vi "界面-新.vi"() -> ()   [LabVIEW 2018]
panel:
  out "已开盖次数":dbl
  in  "保存文件名":string
  in  "保存路径":path
  out "状态记录":string
  in  "保存时间":bool
  out "关盖缓冲异常":bool
  out "字符串 9":string
  out "开盖缓冲异常":bool
  out "字符串 8":string
  in  "开盖次数设置":dbl
  in  "退出系统":bool
  in  "锁定":bool
  in  "压紧":bool
  in  "开盖":bool
  in  "关盖":bool
  in  "解锁":bool
  in  "松开":bool
  in  "井盖 8":bool
  in  "井盖 7":bool
  in  "井盖 6":bool
  in  "井盖 5":bool
  in  "井盖 4":bool
  in  "井盖 3":bool
  in  "井盖 2":bool
  in  "井盖1":bool
  out "字符串 7":string
  out "字符串 6":string
  out "字符串 5":string
  out "字符串 4":string
  out "字符串 3":string
  out "字符串 2":string
  out "解锁异常":bool
  out "压紧时间":dbl
  out "锁定时间":dbl
  out "松开时间":dbl
  out "开盖时间":dbl
  out "解锁时间":dbl
  out "关盖时间":dbl
  out "压紧异常":bool
  out "关盖异常":bool
  out "锁定异常":bool
  out "开盖异常":bool
  out "松开异常":bool
  in  "显示/保存数据":bool
  in  "numsamples":i32=1000
  in  "IP Port 2":string="22222" caption="IP Port"
  in  "IP Address 2":string="192.168.0.10" caption="IP Address"
  in  "间隔时间4s":bool
  in  "间隔时间3s":bool
  in  "间隔时间2s":bool
  in  "调试模式":bool
  in  "自动操作":bool
  in  "手动操作":bool
  in  "系统启动":bool
  out "压紧换向阀":bool
  out "压紧到位":bool
  out "锁定到位":bool
  out "松开换向阀":bool
  out "开盖指令2":bool
  out "开盖指令1":bool
  out "开盖换向阀":bool
  out "开盖缓冲":bool
  out "开盖到位2":bool
  out "解锁到位":bool
  out "关盖指令2":bool
  out "关盖指令1":bool
  out "关盖换向阀":bool
  out "关盖到位2":bool
  out "关盖到位1":bool
  out "松开到位":bool
  out "关盖缓冲":bool
  out "开盖到位1":bool
  out "时间":string
  out "日期":string
  # "数 据 分 析 平 台 监 控 界 面"
  # "动 作 指 令"
  # "状 态 显 示"
  # "报 警 信 息"
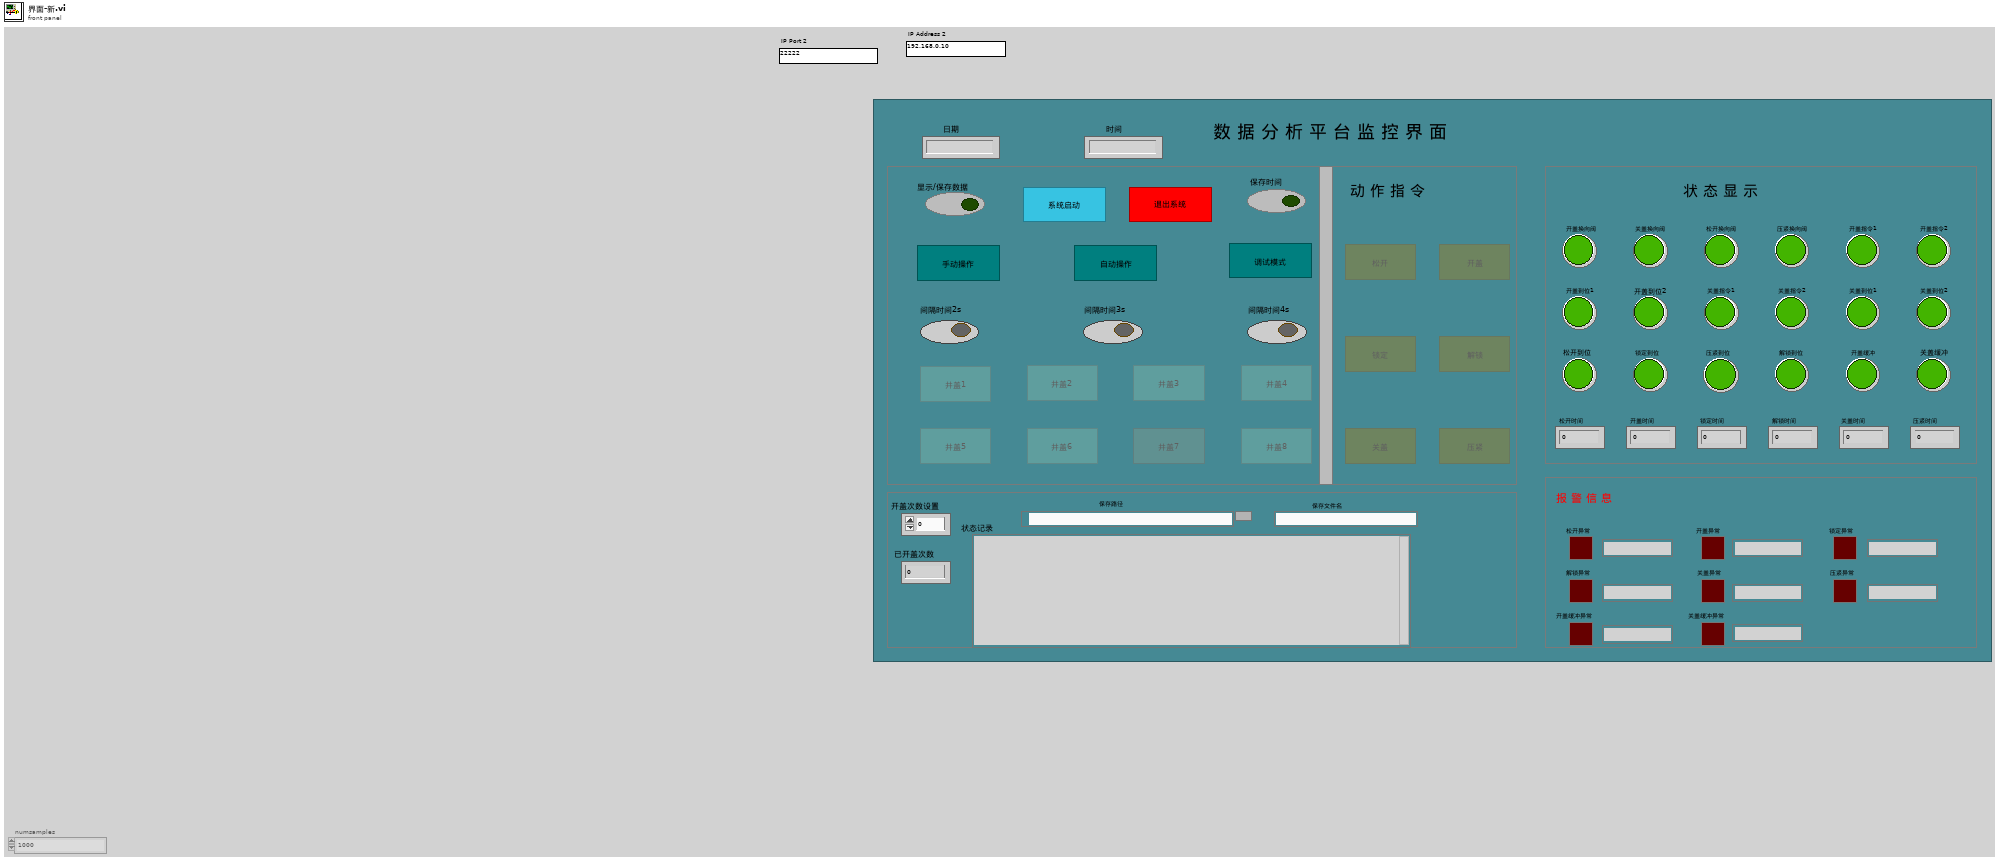
[diagram p1: front panel]
types:
  T1 = enum8{"Enabled", "Disabled", "Disabled and Grayed Out"}
  T2 = enum16{"open", "replace", "create", "open or create", "replace or create", "replace or create with confirmation"}
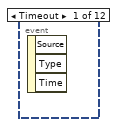
[diagram p17: hidden frame]
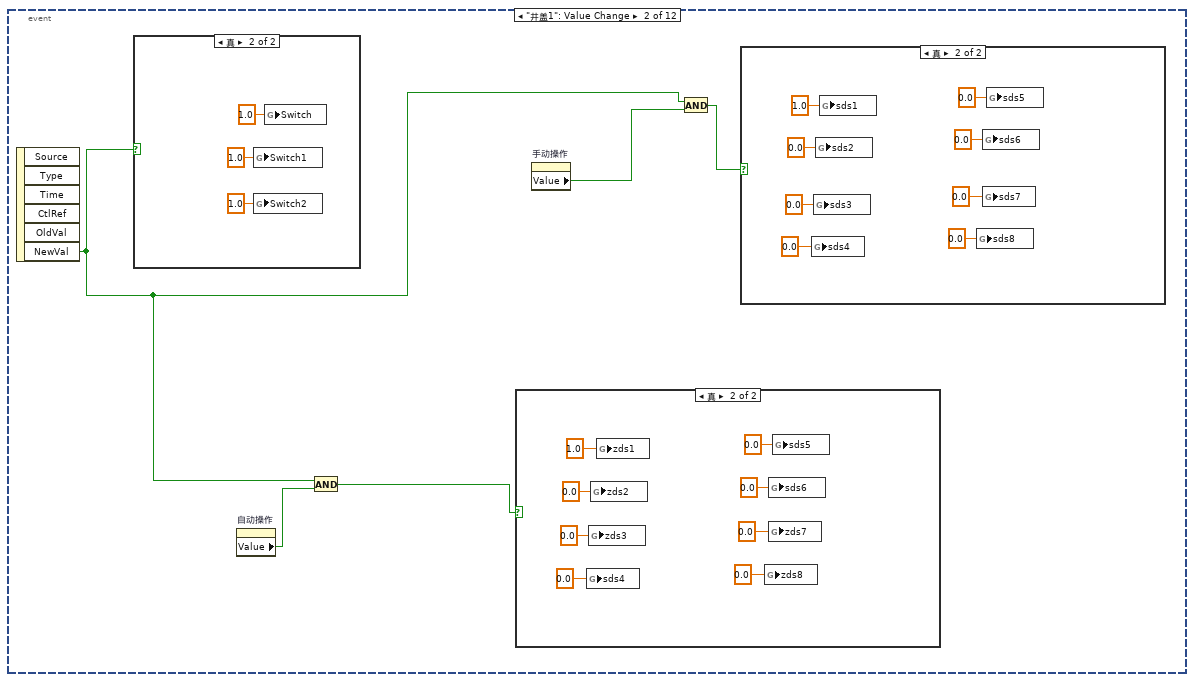
[diagram p18: hidden frame]
diagram:
  w182 = FALSE
  w181 = FALSE
  w171 = FALSE
  w172 = FALSE
  w173 = FALSE
  w174 = FALSE
  w199 = FALSE
  w175 = FALSE
  w176 = FALSE
  w177 = FALSE
  w178 = FALSE
  w179 = FALSE
  w180 = FALSE
  w201 = FALSE
  w202 = FALSE
  w203 = FALSE
  w204 = FALSE
  w205 = FALSE
  w206 = FALSE
  w207 = FALSE
  w200 = FALSE
  w208 = FALSE
  w209 = FALSE
  w210 = FALSE
  w211 = FALSE
  w212 = FALSE
  w213 = FALSE
  w214 = FALSE
  w215 = FALSE
  w216 = FALSE
  w217 = FALSE
  n1 = call "xPCOpenTcpIpPort.vi"("port"="IP Port 2", "address"="IP Address 2") -> ("error out"=w102:errorcluster, "Port"=w93:i32)
  n2 = Unbundle By Name(w102) -> ("status"=w106:bool)
  n3 = call "xPCLoadApp.vi"("pathstr"="C:\\Users\\zczg\\Desktop\\kaigguangai\\remake", "filename"="kaiguangai1108", "port"=w93) -> ("error out"=w103:errorcluster, "port copy"=w92:i32)  [unwired: 1 in]
  n4 = Unbundle By Name(w103) -> ()  [unwired: 1 out]
  n5 = Select(t="上下位机连接失败!" ("message"), s=w106, f="上下位机建立连接!" ("message")) -> ()  [unwired: 1 out]
  n6 = call "xPCStartApp.vi"("port"=w92) -> ("port copy"=w3:i32)  [unwired: 1 in, 1 out]
  n7 = call "xPCGetParamIdx.vi"("blockpath"="shoudongcaozuo/s6", "parametername"="Value", "port"=w3) -> ("identifier"=w382:i32, "port copy"=w383:i32)  [unwired: 1 in, 1 out]
  n8 = call "xPCGetParamIdx.vi"("blockpath"="shoudongcaozuo/s5", "parametername"="Value", "port"=w3) -> ("identifier"=w377:i32, "port copy"=w380:i32)  [unwired: 1 in, 1 out]
  n9 = call "xPCGetParamIdx.vi"("blockpath"="shoudongcaozuo/s3", "parametername"="Value", "port"=w3) -> ("identifier"=w6:i32, "port copy"=w7:i32)  [unwired: 1 in, 1 out]
  n10 = call "xPCGetParamIdx.vi"("blockpath"="shoudongcaozuo/s4", "parametername"="Value", "port"=w3) -> ("identifier"=w373:i32, "port copy"=w374:i32)  [unwired: 1 in, 1 out]
  n11 = for {
    N: 1 -> [_]
    tunnel: [w389] -> w2 mode=indexing
    tunnel: [w388] -> w1 mode=indexing
    tunnel: string[] ["Subsystem1/Data Type Conversion2", "", "", "", "", "", "", "", "", ""] -> [w387] mode=indexing
    tunnel: w3 -> [w386]
    n12 = call "xPCGetSigIdx.vi"("blockpath"=w387, "port"=w386) -> ("identifier"=w388:i32, "port copy"=w389:i32)  [unwired: 1 in, 1 out]
  }
  n13 = call "xPCGetParamIdx.vi"("blockpath"="shoudongcaozuo/s2", "parametername"="Value", "port"=w3) -> ("identifier"=w366:i32, "port copy"=w367:i32)  [unwired: 1 in, 1 out]
  n14 = for {
    N: 6 -> [_]
    tunnel: [w393] -> w114 mode=indexing
    tunnel: [w392] -> w113 mode=indexing
    tunnel: string[] ["Subsystem1/shoudong/Data Type Conversion7/s1", "Subsystem1/shoudong/Data Type Conversion7/s2", "Subsystem1/shoudong/Data Type Conversion7/s3", "Subsystem1/shoudong/Data Type Conversion7/s4", "Subsystem1/shoudong/Data Type Conversion7/s5", "Subsystem1/shoudong/Data Type Conversion7/s6", "", "", "", ""] -> [w391] mode=indexing
    tunnel: w3 -> [w390]
    n15 = call "xPCGetSigIdx.vi"("blockpath"=w391, "port"=w390) -> ("identifier"=w392:i32, "port copy"=w393:i32)  [unwired: 1 in, 1 out]
  }
  n16 = for {
    N: 6 -> [_]
    tunnel: [w397] -> w116 mode=indexing
    tunnel: [w396] -> w115 mode=indexing
    tunnel: string[] ["Subsystem1/shoudong/Data Type Conversion8/s1", "Subsystem1/shoudong/Data Type Conversion8/s2", "Subsystem1/shoudong/Data Type Conversion8/s3", "Subsystem1/shoudong/Data Type Conversion8/s4", "Subsystem1/shoudong/Data Type Conversion8/s5", "Subsystem1/shoudong/Data Type Conversion8/s6", "", "", "", ""] -> [w395] mode=indexing
    tunnel: w3 -> [w394]
    n17 = call "xPCGetSigIdx.vi"("blockpath"=w395, "port"=w394) -> ("identifier"=w396:i32, "port copy"=w397:i32)  [unwired: 1 in, 1 out]
  }
  n18 = for {
    N: 6 -> [_]
    tunnel: [w401] -> w118 mode=indexing
    tunnel: [w400] -> w117 mode=indexing
    tunnel: string[] ["Subsystem1/shoudong/Data Type Conversion9/s1", "Subsystem1/shoudong/Data Type Conversion9/s2", "Subsystem1/shoudong/Data Type Conversion9/s3", "Subsystem1/shoudong/Data Type Conversion9/s4", "Subsystem1/shoudong/Data Type Conversion9/s5", "Subsystem1/shoudong/Data Type Conversion9/s6", "", "", "", ""] -> [w399] mode=indexing
    tunnel: w3 -> [w398]
    n19 = call "xPCGetSigIdx.vi"("blockpath"=w399, "port"=w398) -> ("identifier"=w400:i32, "port copy"=w401:i32)  [unwired: 1 in, 1 out]
  }
  n20 = call "xPCGetParamIdx.vi"("blockpath"="tiaoshidongzuo/yajin", "parametername"="Value", "port"=w3) -> ("identifier"=w17:i32, "port copy"=w18:i32)  [unwired: 1 in, 1 out]
  n21 = for {
    N: 1 -> [_]
    tunnel: [w405] -> w13 mode=indexing
    tunnel: [w404] -> w12 mode=indexing
    tunnel: string[] ["Subsystem1/Data Type Conversion1", "", "", "", "", "", "", "", "", ""] -> [w403] mode=indexing
    tunnel: w3 -> [w402]
    n22 = call "xPCGetSigIdx.vi"("blockpath"=w403, "port"=w402) -> ("identifier"=w404:i32, "port copy"=w405:i32)  [unwired: 1 in, 1 out]
  }
  n23 = call "xPCGetParamIdx.vi"("blockpath"="shoudongcaozuo/s1", "parametername"="Value", "port"=w3) -> ("identifier"=w361:i32, "port copy"=w362:i32)  [unwired: 1 in, 1 out]
  n24 = for {
    N: 1 -> [_]
    tunnel: [w409] -> w9 mode=indexing
    tunnel: [w408] -> w8 mode=indexing
    tunnel: string[] ["Subsystem1/Data Type Conversion2", "", "", "", "", "", "", "", "", ""] -> [w407] mode=indexing
    tunnel: w3 -> [w406]
    n25 = call "xPCGetSigIdx.vi"("blockpath"=w407, "port"=w406) -> ("identifier"=w408:i32, "port copy"=w409:i32)  [unwired: 1 in, 1 out]
  }
  n26 = for {
    N: 6 -> [_]
    tunnel: [w413] -> w120 mode=indexing
    tunnel: [w412] -> w119 mode=indexing
    tunnel: string[] ["Subsystem1/shoudong/Data Type Conversion10/s1", "Subsystem1/shoudong/Data Type Conversion10/s2", "Subsystem1/shoudong/Data Type Conversion10/s3", "Subsystem1/shoudong/Data Type Conversion10/s4", "Subsystem1/shoudong/Data Type Conversion10/s5", "Subsystem1/shoudong/Data Type Conversion10/s6", "", "", "", ""] -> [w411] mode=indexing
    tunnel: w3 -> [w410]
    n27 = call "xPCGetSigIdx.vi"("blockpath"=w411, "port"=w410) -> ("identifier"=w412:i32, "port copy"=w413:i32)  [unwired: 1 in, 1 out]
  }
  n28 = call "xPCGetParamIdx.vi"("blockpath"="tiaoshidongzuo/jiesuo", "parametername"="Value", "port"=w3) -> ("identifier"=w29:i32, "port copy"=w30:i32)  [unwired: 1 in, 1 out]
  n29 = call "xPCGetParamIdx.vi"("blockpath"="shoudongcaozuo/s7", "parametername"="Value", "port"=w3) -> ("identifier"=w194:i32, "port copy"=w195:i32)  [unwired: 1 in, 1 out]
  n30 = call "xPCGetParamIdx.vi"("blockpath"="tiaoshidongzuo/kaigai", "parametername"="Value", "port"=w3) -> ("identifier"=w26:i32, "port copy"=w27:i32)  [unwired: 1 in, 1 out]
  n31 = for {
    N: 6 -> [_]
    tunnel: [w417] -> w112 mode=indexing
    tunnel: [w416] -> w111 mode=indexing
    tunnel: string[] ["Subsystem1/shoudong/Data Type Conversion6/s1", "Subsystem1/shoudong/Data Type Conversion6/s2", "Subsystem1/shoudong/Data Type Conversion6/s3", "Subsystem1/shoudong/Data Type Conversion6/s4", "Subsystem1/shoudong/Data Type Conversion6/s5", "Subsystem1/shoudong/Data Type Conversion6/s6", "", "", "", ""] -> [w415] mode=indexing
    tunnel: w3 -> [w414]
    n32 = call "xPCGetSigIdx.vi"("blockpath"=w415, "port"=w414) -> ("identifier"=w416:i32, "port copy"=w417:i32)  [unwired: 1 in, 1 out]
  }
  n33 = for {
    N: 6 -> [_]
    tunnel: [w421] -> w160 mode=indexing
    tunnel: [w420] -> w159 mode=indexing
    tunnel: string[] ["Subsystem1/zidong/Data Type Conversion3/s1", "Subsystem1/zidong/Data Type Conversion3/s2", "Subsystem1/zidong/Data Type Conversion3/s3", "Subsystem1/zidong/Data Type Conversion3/s4", "Subsystem1/zidong/Data Type Conversion3/s5", "Subsystem1/zidong/Data Type Conversion3/s6", "", "", "", ""] -> [w419] mode=indexing
    tunnel: w3 -> [w418]
    n34 = call "xPCGetSigIdx.vi"("blockpath"=w419, "port"=w418) -> ("identifier"=w420:i32, "port copy"=w421:i32)  [unwired: 1 in, 1 out]
  }
  n35 = for {
    N: 6 -> [_]
    tunnel: [w425] -> w144 mode=indexing
    tunnel: [w424] -> w143 mode=indexing
    tunnel: string[] ["Subsystem1/zidong/Data Type Conversion5/s1", "Subsystem1/zidong/Data Type Conversion5/s2", "Subsystem1/zidong/Data Type Conversion5/s3", "Subsystem1/zidong/Data Type Conversion5/s4", "Subsystem1/zidong/Data Type Conversion5/s5", "Subsystem1/zidong/Data Type Conversion5/s6", "", "", "", ""] -> [w423] mode=indexing
    tunnel: w3 -> [w422]
    n36 = call "xPCGetSigIdx.vi"("blockpath"=w423, "port"=w422) -> ("identifier"=w424:i32, "port copy"=w425:i32)  [unwired: 1 in, 1 out]
  }
  n37 = call "xPCGetParamIdx.vi"("blockpath"="tiaoshidongzuo/suoding", "parametername"="Value", "port"=w3) -> ("identifier"=w20:i32, "port copy"=w21:i32)  [unwired: 1 in, 1 out]
  n38 = call "xPCGetParamIdx.vi"("blockpath"="shoudongcaozuo/jiesuo", "parametername"="Value", "port"=w3) -> ("identifier"=w346:i32, "port copy"=w347:i32)  [unwired: 1 in, 1 out]
  n39 = call "xPCGetParamIdx.vi"("blockpath"="shoudongcaozuo/suoding", "parametername"="Value", "port"=w3) -> ("identifier"=w341:i32, "port copy"=w342:i32)  [unwired: 1 in, 1 out]
  n40 = for {
    N: 6 -> [_]
    tunnel: [w429] -> w138 mode=indexing
    tunnel: [w428] -> w137 mode=indexing
    tunnel: string[] ["Subsystem1/zidong/Data Type Conversion8/s1", "Subsystem1/zidong/Data Type Conversion8/s2", "Subsystem1/zidong/Data Type Conversion8/s3", "Subsystem1/zidong/Data Type Conversion8/s4", "Subsystem1/zidong/Data Type Conversion8/s5", "Subsystem1/zidong/Data Type Conversion8/s6", "", "", "", ""] -> [w427] mode=indexing
    tunnel: w3 -> [w426]
    n41 = call "xPCGetSigIdx.vi"("blockpath"=w427, "port"=w426) -> ("identifier"=w428:i32, "port copy"=w429:i32)  [unwired: 1 in, 1 out]
  }
  n42 = for {
    N: 6 -> [_]
    tunnel: [w433] -> w164 mode=indexing
    tunnel: [w432] -> w163 mode=indexing
    tunnel: string[] ["Subsystem1/zidong/Data Type Conversion1/s1", "Subsystem1/zidong/Data Type Conversion1/s2", "Subsystem1/zidong/Data Type Conversion1/s3", "Subsystem1/zidong/Data Type Conversion1/s4", "Subsystem1/zidong/Data Type Conversion1/s5", "Subsystem1/zidong/Data Type Conversion1/s6", "", "", "", ""] -> [w431] mode=indexing
    tunnel: w3 -> [w430]
    n43 = call "xPCGetSigIdx.vi"("blockpath"=w431, "port"=w430) -> ("identifier"=w432:i32, "port copy"=w433:i32)  [unwired: 1 in, 1 out]
  }
  n44 = for {
    N: 6 -> [_]
    tunnel: [w437] -> w156 mode=indexing
    tunnel: [w436] -> w155 mode=indexing
    tunnel: string[] ["Subsystem1/zidong/Data Type Conversion4/s1", "Subsystem1/zidong/Data Type Conversion4/s2", "Subsystem1/zidong/Data Type Conversion4/s3", "Subsystem1/zidong/Data Type Conversion4/s4", "Subsystem1/zidong/Data Type Conversion4/s5", "Subsystem1/zidong/Data Type Conversion4/s6", "", "", "", ""] -> [w435] mode=indexing
    tunnel: w3 -> [w434]
    n45 = call "xPCGetSigIdx.vi"("blockpath"=w435, "port"=w434) -> ("identifier"=w436:i32, "port copy"=w437:i32)  [unwired: 1 in, 1 out]
  }
  n46 = call "xPCGetParamIdx.vi"("blockpath"="shoudongcaozuo/yajin", "parametername"="Value", "port"=w3) -> ("identifier"=w355:i32, "port copy"=w356:i32)  [unwired: 1 in, 1 out]
  n47 = call "xPCGetParamIdx.vi"("blockpath"="shoudongcaozuo/kaigai", "parametername"="Value", "port"=w3) -> ("identifier"=w336:i32, "port copy"=w337:i32)  [unwired: 1 in, 1 out]
  n48 = for {
    N: 4 -> [_]
    tunnel: [w441] -> w219 mode=indexing
    tunnel: [w440] -> w218 mode=indexing
    tunnel: string[] ["Subsystem1/Data Type Conversion1/s1", "Subsystem1/Data Type Conversion1/s2", "Subsystem1/Data Type Conversion1/s3", "Subsystem1/Data Type Conversion1/s4"] -> [w439] mode=indexing
    tunnel: w3 -> [w438]
    n49 = call "xPCGetSigIdx.vi"("blockpath"=w439, "port"=w438) -> ("identifier"=w440:i32, "port copy"=w441:i32)  [unwired: 1 in, 1 out]
  }
  n50 = call "xPCGetParamIdx.vi"("blockpath"="shoudongcaozuo/guangai", "parametername"="Value", "port"=w3) -> ("identifier"=w352:i32, "port copy"=w353:i32)  [unwired: 1 in, 1 out]
  n51 = for {
    N: 6 -> [_]
    tunnel: [w445] -> w136 mode=indexing
    tunnel: [w444] -> w135 mode=indexing
    tunnel: string[] ["Subsystem1/shoudong/Data Type Conversion1/s1", "Subsystem1/shoudong/Data Type Conversion1/s2", "Subsystem1/shoudong/Data Type Conversion1/s3", "Subsystem1/shoudong/Data Type Conversion1/s4", "Subsystem1/shoudong/Data Type Conversion1/s5", "Subsystem1/shoudong/Data Type Conversion1/s6", "", "", "", ""] -> [w443] mode=indexing
    tunnel: w3 -> [w442]
    n52 = call "xPCGetSigIdx.vi"("blockpath"=w443, "port"=w442) -> ("identifier"=w444:i32, "port copy"=w445:i32)  [unwired: 1 in, 1 out]
  }
  n53 = for {
    N: 6 -> [_]
    tunnel: [w449] -> w140 mode=indexing
    tunnel: [w448] -> w139 mode=indexing
    tunnel: string[] ["Subsystem1/zidong/Data Type Conversion7/s1", "Subsystem1/zidong/Data Type Conversion7/s2", "Subsystem1/zidong/Data Type Conversion7/s3", "Subsystem1/zidong/Data Type Conversion7/s4", "Subsystem1/zidong/Data Type Conversion7/s5", "Subsystem1/zidong/Data Type Conversion7/s6", "", "", "", ""] -> [w447] mode=indexing
    tunnel: w3 -> [w446]
    n54 = call "xPCGetSigIdx.vi"("blockpath"=w447, "port"=w446) -> ("identifier"=w448:i32, "port copy"=w449:i32)  [unwired: 1 in, 1 out]
  }
  n55 = call "xPCGetParamIdx.vi"("blockpath"="tiaoshidongzuo/songkai", "parametername"="Value", "port"=w3) -> ("identifier"=w23:i32, "port copy"=w24:i32)  [unwired: 1 in, 1 out]
  n56 = for {
    N: 6 -> [_]
    tunnel: [w453] -> w142 mode=indexing
    tunnel: [w452] -> w141 mode=indexing
    tunnel: string[] ["Subsystem1/zidong/Data Type Conversion6/s1", "Subsystem1/zidong/Data Type Conversion6/s2", "Subsystem1/zidong/Data Type Conversion6/s3", "Subsystem1/zidong/Data Type Conversion6/s4", "Subsystem1/zidong/Data Type Conversion6/s5", "Subsystem1/zidong/Data Type Conversion6/s6", "", "", "", ""] -> [w451] mode=indexing
    tunnel: w3 -> [w450]
    n57 = call "xPCGetSigIdx.vi"("blockpath"=w451, "port"=w450) -> ("identifier"=w452:i32, "port copy"=w453:i32)  [unwired: 1 in, 1 out]
  }
  n58 = for {
    N: 6 -> [_]
    tunnel: [w457] -> w110 mode=indexing
    tunnel: [w456] -> w109 mode=indexing
    tunnel: string[] ["Subsystem1/shoudong/Data Type Conversion5/s1", "Subsystem1/shoudong/Data Type Conversion5/s2", "Subsystem1/shoudong/Data Type Conversion5/s3", "Subsystem1/shoudong/Data Type Conversion5/s4", "Subsystem1/shoudong/Data Type Conversion5/s5", "Subsystem1/shoudong/Data Type Conversion5/s6", "", "", "", ""] -> [w455] mode=indexing
    tunnel: w3 -> [w454]
    n59 = call "xPCGetSigIdx.vi"("blockpath"=w455, "port"=w454) -> ("identifier"=w456:i32, "port copy"=w457:i32)  [unwired: 1 in, 1 out]
  }
  n60 = call "xPCGetParamIdx.vi"("blockpath"="tiaoshidongzuo/guangai", "parametername"="Value", "port"=w3) -> ("identifier"=w32:i32, "port copy"=w33:i32)  [unwired: 1 in, 1 out]
  n61 = for {
    N: 6 -> [_]
    tunnel: [w461] -> w108 mode=indexing
    tunnel: [w460] -> w107 mode=indexing
    tunnel: string[] ["Subsystem1/shoudong/Data Type Conversion2/s1", "Subsystem1/shoudong/Data Type Conversion2/s2", "Subsystem1/shoudong/Data Type Conversion2/s3", "Subsystem1/shoudong/Data Type Conversion2/s4", "Subsystem1/shoudong/Data Type Conversion2/s5", "Subsystem1/shoudong/Data Type Conversion2/s6", "", "", "", ""] -> [w459] mode=indexing
    tunnel: w3 -> [w458]
    n62 = call "xPCGetSigIdx.vi"("blockpath"=w459, "port"=w458) -> ("identifier"=w460:i32, "port copy"=w461:i32)  [unwired: 1 in, 1 out]
  }
  n63 = call "xPCGetParamIdx.vi"("blockpath"="shoudongcaozuo/s8", "parametername"="Value", "port"=w3) -> ("identifier"=w95:i32, "port copy"=w96:i32)  [unwired: 1 in, 1 out]
  n64 = for {
    N: 4 -> [_]
    tunnel: [w465] -> w225 mode=indexing
    tunnel: [w464] -> w224 mode=indexing
    tunnel: string[] ["Data Type Conversion2/s1", "Data Type Conversion2/s2", "Data Type Conversion2/s3", "Data Type Conversion2/s4", "", "", "", ""] -> [w463] mode=indexing
    tunnel: w3 -> [w462]
    n65 = call "xPCGetSigIdx.vi"("blockpath"=w463, "port"=w462) -> ("identifier"=w464:i32, "port copy"=w465:i32)  [unwired: 1 in, 1 out]
  }
  n66 = for {
    N: 6 -> [_]
    tunnel: [w469] -> w222 mode=indexing
    tunnel: [w468] -> w221 mode=indexing
    tunnel: string[] ["Data Type Conversion/s1", "Data Type Conversion/s2", "Data Type Conversion/s3", "Data Type Conversion/s4", "Data Type Conversion/s5", "Data Type Conversion/s6"] -> [w467] mode=indexing
    tunnel: w3 -> [w466]
    n67 = call "xPCGetSigIdx.vi"("blockpath"=w467, "port"=w466) -> ("identifier"=w468:i32, "port copy"=w469:i32)  [unwired: 1 in, 1 out]
  }
  n68 = for {
    N: 6 -> [_]
    tunnel: [w473] -> w168 mode=indexing
    tunnel: [w472] -> w167 mode=indexing
    tunnel: string[] ["Subsystem1/zidong/Data Type Conversion2/s1", "Subsystem1/zidong/Data Type Conversion2/s2", "Subsystem1/zidong/Data Type Conversion2/s3", "Subsystem1/zidong/Data Type Conversion2/s4", "Subsystem1/zidong/Data Type Conversion2/s5", "Subsystem1/zidong/Data Type Conversion2/s6", "", "", "", ""] -> [w471] mode=indexing
    tunnel: w3 -> [w470]
    n69 = call "xPCGetSigIdx.vi"("blockpath"=w471, "port"=w470) -> ("identifier"=w472:i32, "port copy"=w473:i32)  [unwired: 1 in, 1 out]
  }
  n70 = call "xPCGetParamIdx.vi"("blockpath"="Switch2", "parametername"="Value", "port"=w3) -> ("identifier"=w327:i32, "port copy"=w328:i32)  [unwired: 1 in, 1 out]
  n71 = call "xPCGetParamIdx.vi"("blockpath"="tiaoshidongzuo/s3", "parametername"="Value", "port"=w3) -> ("identifier"=w62:i32, "port copy"=w63:i32)  [unwired: 1 in, 1 out]
  n72 = for {
    N: 10 -> [_]
    tunnel: [w477] -> w228 mode=indexing
    tunnel: [w476] -> w227 mode=indexing
    tunnel: string[] ["Data Type Conversion1/s1", "Data Type Conversion1/s2", "Data Type Conversion1/s3", "Data Type Conversion1/s4", "Data Type Conversion1/s5", "Data Type Conversion1/s6", "Data Type Conversion1/s7", "Data Type Conversion1/s8", "Data Type Conversion1/s9", "Data Type Conversion1/s10"] -> [w475] mode=indexing
    tunnel: w3 -> [w474]
    n73 = call "xPCGetSigIdx.vi"("blockpath"=w475, "port"=w474) -> ("identifier"=w476:i32, "port copy"=w477:i32)  [unwired: 1 in, 1 out]
  }
  n74 = call "xPCGetParamIdx.vi"("blockpath"="tiaoshidongzuo/s4", "parametername"="Value", "port"=w3) -> ("identifier"=w59:i32, "port copy"=w60:i32)  [unwired: 1 in, 1 out]
  n75 = call "xPCGetParamIdx.vi"("blockpath"="shoudongcaozuo/songkai", "parametername"="Value", "port"=w3) -> ("identifier"=w331:i32, "port copy"=w332:i32)  [unwired: 1 in, 1 out]
  n76 = call "xPCGetParamIdx.vi"("blockpath"="tiaoshidongzuo/s1", "parametername"="Value", "port"=w3) -> ("identifier"=w68:i32, "port copy"=w69:i32)  [unwired: 1 in, 1 out]
  n77 = call "xPCGetParamIdx.vi"("blockpath"="Switch1", "parametername"="Value", "port"=w3) -> ("identifier"=w323:i32, "port copy"=w324:i32)  [unwired: 1 in, 1 out]
  n78 = call "xPCGetParamIdx.vi"("blockpath"="tiaoshidongzuo/s2", "parametername"="Value", "port"=w3) -> ("identifier"=w65:i32, "port copy"=w66:i32)  [unwired: 1 in, 1 out]
  n79 = call "xPCGetParamIdx.vi"("blockpath"="Switch", "parametername"="Value", "port"=w3) -> ("identifier"=w317:i32, "port copy"=w318:i32)  [unwired: 1 in, 1 out]
  n80 = call "xPCGetParamIdx.vi"("blockpath"="tiaoshi", "parametername"="Value", "port"=w3) -> ("identifier"=w86:i32, "port copy"=w87:i32)  [unwired: 1 in, 1 out]
  n81 = call "xPCGetParamIdx.vi"("blockpath"="tiaoshidongzuo/s7", "parametername"="Value", "port"=w3) -> ("identifier"=w50:i32, "port copy"=w51:i32)  [unwired: 1 in, 1 out]
  n82 = call "xPCGetParamIdx.vi"("blockpath"="tiaoshidongzuo/s6", "parametername"="Value", "port"=w3) -> ("identifier"=w53:i32, "port copy"=w54:i32)  [unwired: 1 in, 1 out]
  n83 = call "xPCGetParamIdx.vi"("blockpath"="tiaoshidongzuo/s8", "parametername"="Value", "port"=w3) -> ("identifier"=w47:i32, "port copy"=w48:i32)  [unwired: 1 in, 1 out]
  n84 = call "xPCGetParamIdx.vi"("blockpath"="tiaoshidongzuo/s5", "parametername"="Value", "port"=w3) -> ("identifier"=w56:i32, "port copy"=w57:i32)  [unwired: 1 in, 1 out]
  n85 = call "xPCGetParamIdx.vi"("blockpath"="zidong_jiangeshijian/t1", "parametername"="Value", "port"=w3) -> ("identifier"=w313:i32, "port copy"=w314:i32)  [unwired: 1 in, 1 out]
  n86 = call "xPCGetParamIdx.vi"("blockpath"="zidong_jiangeshijian/t9", "parametername"="Value", "port"=w3) -> ("identifier"=w292:i32, "port copy"=w293:i32)  [unwired: 1 in, 1 out]
  n87 = call "xPCGetParamIdx.vi"("blockpath"="zidong_jiangeshijian/t7", "parametername"="Value", "port"=w3) -> ("identifier"=w295:i32, "port copy"=w296:i32)  [unwired: 1 in, 1 out]
  n88 = call "xPCGetParamIdx.vi"("blockpath"="zidong_jiangeshijian/t3", "parametername"="Value", "port"=w3) -> ("identifier"=w307:i32, "port copy"=w308:i32)  [unwired: 1 in, 1 out]
  n89 = call "xPCGetParamIdx.vi"("blockpath"="zidong_jiangeshijian/t5", "parametername"="Value", "port"=w3) -> ("identifier"=w302:i32, "port copy"=w303:i32)  [unwired: 1 in, 1 out]
  n90 = call "xPCGetParamIdx.vi"("blockpath"="zidong_jiangeshijian/t11", "parametername"="Value", "port"=w3) -> ("identifier"=w288:i32, "port copy"=w289:i32)  [unwired: 1 in, 1 out]
  n91 = call "xPCGetParamIdx.vi"("blockpath"="start", "parametername"="Value", "port"=w3) -> ("identifier"=w231:i32, "port copy"=w232:i32)  [unwired: 1 in, 1 out]
  n92 = call "xPCGetParamIdx.vi"("blockpath"="Subsystem1/jinggaixuanze/jinggai1", "parametername"="Value", "port"=w3) -> ("identifier"=w281:i32, "port copy"=w282:i32)  [unwired: 1 in, 1 out]
  n93 = call "xPCGetParamIdx.vi"("blockpath"="Subsystem1/jinggaixuanze/jinggai5", "parametername"="Value", "port"=w3) -> ("identifier"=w261:i32, "port copy"=w262:i32)  [unwired: 1 in, 1 out]
  n94 = call "xPCGetParamIdx.vi"("blockpath"="Subsystem1/jinggaixuanze/jinggai4", "parametername"="Value", "port"=w3) -> ("identifier"=w266:i32, "port copy"=w267:i32)  [unwired: 1 in, 1 out]
  n95 = call "xPCGetParamIdx.vi"("blockpath"="Subsystem1/jinggaixuanze/jinggai8", "parametername"="Value", "port"=w3) -> ("identifier"=w248:i32, "port copy"=w249:i32)  [unwired: 1 in, 1 out]
  n96 = call "xPCGetParamIdx.vi"("blockpath"="Subsystem1/jinggaixuanze/jinggai2", "parametername"="Value", "port"=w3) -> ("identifier"=w277:i32, "port copy"=w278:i32)  [unwired: 1 in, 1 out]
  n97 = call "xPCGetParamIdx.vi"("blockpath"="jieshu", "parametername"="Value", "port"=w3) -> ("identifier"=w241:i32, "port copy"=w242:i32)  [unwired: 1 in, 1 out]
  n98 = call "xPCGetParamIdx.vi"("blockpath"="Subsystem1/jinggaixuanze/jinggai6", "parametername"="Value", "port"=w3) -> ("identifier"=w256:i32, "port copy"=w257:i32)  [unwired: 1 in, 1 out]
  n99 = call "xPCGetParamIdx.vi"("blockpath"="qiehuan", "parametername"="Value", "port"=w3) -> ("identifier"=w184:i32, "port copy"=w185:i32)  [unwired: 1 in, 1 out]
  n100 = call "xPCGetParamIdx.vi"("blockpath"="zidong_shedingcishu", "parametername"="Value", "port"=w3) -> ("identifier"=w238:i32, "port copy"=w239:i32)  [unwired: 1 in, 1 out]
  n101 = call "xPCGetParamIdx.vi"("blockpath"="Subsystem1/jinggaixuanze/jinggai7", "parametername"="Value", "port"=w3) -> ("identifier"=w253:i32, "port copy"=w254:i32)  [unwired: 1 in, 1 out]
  n102 = call "xPCGetParamIdx.vi"("blockpath"="Subsystem1/jinggaixuanze/jinggai3", "parametername"="Value", "port"=w3) -> ("identifier"=w271:i32, "port copy"=w272:i32)  [unwired: 1 in, 1 out]
  n103 = while {
    tunnel: w69 -> [w564]
    tunnel: w68 -> [w563]
    shift-right: [w561] -> _
    shift-left: 0.0 -> [w562]
    tunnel: w66 -> [w560]
    tunnel: w65 -> [w559]
    shift-right: [w557] -> _
    shift-left: 0.0 -> [w558]
    tunnel: w63 -> [w556]
    tunnel: w62 -> [w555]
    shift-right: [w553] -> _
    shift-left: 0.0 -> [w554]
    tunnel: w60 -> [w552]
    tunnel: w59 -> [w551]
    shift-right: [w549] -> _
    shift-left: 0.0 -> [w550]
    tunnel: w57 -> [w548]
    tunnel: w56 -> [w547]
    shift-right: [w545] -> _
    shift-left: 0.0 -> [w546]
    tunnel: w54 -> [w544]
    tunnel: w53 -> [w543]
    shift-right: [w541] -> _
    shift-left: 0.0 -> [w542]
    tunnel: w51 -> [w540]
    tunnel: w50 -> [w539]
    shift-right: [w537] -> _
    shift-left: 0.0 -> [w538]
    tunnel: w48 -> [w536]
    tunnel: w47 -> [w535]
    shift-right: [w533] -> _
    shift-left: 0.0 -> [w534]
    tunnel: w33 -> [w520]
    tunnel: w32 -> [w519]
    shift-right: [w517] -> _
    shift-left: 0.0 -> [w518]
    tunnel: w30 -> [w516]
    tunnel: w29 -> [w515]
    shift-right: [w513] -> _
    shift-left: 0.0 -> [w514]
    tunnel: w27 -> [w512]
    tunnel: w26 -> [w511]
    shift-right: [w509] -> _
    shift-left: 0.0 -> [w510]
    tunnel: w24 -> [w508]
    tunnel: w23 -> [w507]
    shift-right: [w505] -> _
    shift-left: 0.0 -> [w506]
    tunnel: w21 -> [w504]
    tunnel: w20 -> [w503]
    shift-right: [w501] -> _
    shift-left: 0.0 -> [w502]
    tunnel: w18 -> [w500]
    tunnel: w17 -> [w499]
    shift-right: [w497] -> _
    shift-left: 0.0 -> [w498]
    tunnel: w13 -> [w491]
    tunnel: w12 -> [w490]
    tunnel: w9 -> [w484]
    tunnel: w8 -> [w483]
    tunnel: w2 -> [w479]
    tunnel: w1 -> [w478]
    stop <- w581 stop-if-true
    n104 = for {
      tunnel: [w591] -> w492 mode=indexing
      tunnel: w491 -> [w590] mode=indexing
      tunnel: w490 -> [w589] mode=indexing
      n105 = call "xPCGetSignal.vi"("signal"=w589, "port"=w590) -> ("Output Value"=w591:dbl)  [unwired: 1 in, 2 out]
    }
    n106 = for {
      tunnel: [w588] -> w485 mode=indexing
      tunnel: w484 -> [w587] mode=indexing
      tunnel: w483 -> [w586] mode=indexing
      n107 = call "xPCGetSignal.vi"("signal"=w586, "port"=w587) -> ("Output Value"=w588:dbl)  [unwired: 1 in, 2 out]
    }
    n108 = for {
      tunnel: [w585] -> w481 mode=indexing
      tunnel: w479 -> [w584] mode=indexing
      tunnel: w478 -> [w583] mode=indexing
      n109 = call "xPCGetSignal.vi"("signal"=w583, "port"=w584) -> ("Output Value"=w585:dbl)  [unwired: 1 in, 2 out]
    }
    n110 = global read "全局变量.vi" "tskaishi4"() -> (w549:dbl)
    n111 = Index Array(array=w492, index=0 ("索引")) -> (element=w495:dbl)
    n112 = global read "全局变量.vi" "tskaishi1"() -> (w561:dbl)
    n113 = global read "全局变量.vi" "tskaishi3"() -> (w553:dbl)
    n114 = global read "全局变量.vi" "tskaishi2"() -> (w557:dbl)
    n115 = Index Array(array=w485, index=0 ("索引")) -> (element=w488:dbl)
    n116 = global read "全局变量.vi" "tskaishi8"() -> (w533:dbl)
    n117 = Equal?(x=w495, y=1.0) -> (x = y?=w493:bool)
    n118 = global read "全局变量.vi" "tskaishi5"() -> (w545:dbl)
    n119 = global read "全局变量.vi" "tskaishi7"() -> (w537:dbl)
    n120 = global read "全局变量.vi" "tskaishi6"() -> (w541:dbl)
    n121 = global read "全局变量.vi" "tssongkai"() -> (w505:dbl)
    n122 = Equal?(x=w488, y=1.0) -> (x = y?=w486:bool)
    n123 = global read "全局变量.vi" "tsguangai"() -> (w517:dbl)
    n124 = Index Array(array=w481, index=0 ("索引")) -> (element=w480:dbl)
    n125 = global read "全局变量.vi" "tskaigai"() -> (w509:dbl)
    n126 = global read "全局变量.vi" "tsjiesuo"() -> (w513:dbl)
    n127 = global write "全局变量.vi" "开盖缓冲异常"(w493) -> ()
    n128 = Not Equal?(x=w550, y=w549) -> (x != y?=w574:bool)
    n129 = Not Equal?(x=w554, y=w553) -> (x != y?=w576:bool)
    n130 = Not Equal?(x=w558, y=w557) -> (x != y?=w578:bool)
    n131 = Not Equal?(x=w562, y=w561) -> (x != y?=w580:bool)
    n132 = global write "全局变量.vi" "关盖缓冲异常"(w486) -> ()
    n133 = global read "全局变量.vi" "tssuoding"() -> (w501:dbl)
    n134 = global read "全局变量.vi" "tsyajin"() -> (w497:dbl)
    n135 = global write "全局变量.vi" "已开盖次数"(w480) -> ()
    n136 = Not Equal?(x=w534, y=w533) -> (x != y?=w566:bool)
    n137 = Not Equal?(x=w538, y=w537) -> (x != y?=w568:bool)
    n138 = Not Equal?(x=w542, y=w541) -> (x != y?=w570:bool)
    n139 = Not Equal?(x=w546, y=w545) -> (x != y?=w572:bool)
    n140 = Build Array(w557) -> (w577:dbl[])
    n141 = Not Equal?(x=w506, y=w505) -> (x != y?=w526:bool)
    n142 = Not Equal?(x=w510, y=w509) -> (x != y?=w528:bool)
    n143 = Build Array(w553) -> (w575:dbl[])
    n144 = Not Equal?(x=w514, y=w513) -> (x != y?=w530:bool)
    n145 = Not Equal?(x=w518, y=w517) -> (x != y?=w532:bool)
    n146 = Build Array(w561) -> (w579:dbl[])
    n147 = Build Array(w549) -> (w573:dbl[])
    n148 = Build Array(w541) -> (w569:dbl[])
    n149 = Build Array(w537) -> (w567:dbl[])
    n150 = Not Equal?(x=w498, y=w497) -> (x != y?=w522:bool)
    n151 = case shown="真" w580 {
      tunnel: w579 -> [_ w633]
      tunnel: w564 -> [_ w632]
      tunnel: w563 -> [_ w631]
      frame False {
      }
      frame True {
        n152 = call "xPCSetParam.vi"("value"=w633, "index"=w631, "port"=w632) -> ()  [unwired: 1 in, 2 out]
      }
    }
    n153 = Not Equal?(x=w502, y=w501) -> (x != y?=w524:bool)
    n154 = Build Array(w513) -> (w529:dbl[])
    n155 = case shown="真" w578 {
      tunnel: w577 -> [_ w630]
      tunnel: w560 -> [_ w629]
      tunnel: w559 -> [_ w628]
      frame False {
      }
      frame True {
        n156 = call "xPCSetParam.vi"("value"=w630, "index"=w628, "port"=w629) -> ()  [unwired: 1 in, 2 out]
      }
    }
    n157 = Build Array(w545) -> (w571:dbl[])
    n158 = case shown="真" w574 {
      tunnel: w573 -> [_ w624]
      tunnel: w552 -> [_ w623]
      tunnel: w551 -> [_ w622]
      frame False {
      }
      frame True {
        n159 = call "xPCSetParam.vi"("value"=w624, "index"=w622, "port"=w623) -> ()  [unwired: 1 in, 2 out]
      }
    }
    n160 = case shown="真" w576 {
      tunnel: w575 -> [_ w627]
      tunnel: w556 -> [_ w626]
      tunnel: w555 -> [_ w625]
      frame False {
      }
      frame True {
        n161 = call "xPCSetParam.vi"("value"=w627, "index"=w625, "port"=w626) -> ()  [unwired: 1 in, 2 out]
      }
    }
    n162 = Build Array(w533) -> (w565:dbl[])
    n163 = Build Array(w509) -> (w527:dbl[])
    n164 = Build Array(w505) -> (w525:dbl[])
    n165 = Build Array(w517) -> (w531:dbl[])
    n166 = case shown="真" w572 {
      tunnel: w571 -> [_ w621]
      tunnel: w548 -> [_ w620]
      tunnel: w547 -> [_ w619]
      frame False {
      }
      frame True {
        n167 = call "xPCSetParam.vi"("value"=w621, "index"=w619, "port"=w620) -> ()  [unwired: 1 in, 2 out]
      }
    }
    n168 = Build Array(w497) -> (w521:dbl[])
    n169 = case shown="真" w570 {
      tunnel: w569 -> [_ w618]
      tunnel: w544 -> [_ w617]
      tunnel: w543 -> [_ w616]
      frame False {
      }
      frame True {
        n170 = call "xPCSetParam.vi"("value"=w618, "index"=w616, "port"=w617) -> ()  [unwired: 1 in, 2 out]
      }
    }
    n171 = case shown="真" w566 {
      tunnel: w565 -> [_ w612]
      tunnel: w536 -> [_ w611]
      tunnel: w535 -> [_ w610]
      frame False {
      }
      frame True {
        n172 = call "xPCSetParam.vi"("value"=w612, "index"=w610, "port"=w611) -> ()  [unwired: 1 in, 2 out]
      }
    }
    n173 = case shown="真" w568 {
      tunnel: w567 -> [_ w615]
      tunnel: w540 -> [_ w614]
      tunnel: w539 -> [_ w613]
      frame False {
      }
      frame True {
        n174 = call "xPCSetParam.vi"("value"=w615, "index"=w613, "port"=w614) -> ()  [unwired: 1 in, 2 out]
      }
    }
    n175 = case shown="真" w532 {
      tunnel: w531 -> [_ w609]
      tunnel: w520 -> [_ w608]
      tunnel: w519 -> [_ w607]
      frame False {
      }
      frame True {
        n176 = call "xPCSetParam.vi"("value"=w609, "index"=w607, "port"=w608) -> ()  [unwired: 1 in, 2 out]
      }
    }
    n177 = case shown="真" w530 {
      tunnel: w529 -> [_ w606]
      tunnel: w516 -> [_ w605]
      tunnel: w515 -> [_ w604]
      frame False {
      }
      frame True {
        n178 = call "xPCSetParam.vi"("value"=w606, "index"=w604, "port"=w605) -> ()  [unwired: 1 in, 2 out]
      }
    }
    n179 = Build Array(w501) -> (w523:dbl[])
    n180 = case shown="真" w526 {
      tunnel: w525 -> [_ w600]
      tunnel: w508 -> [_ w599]
      tunnel: w507 -> [_ w598]
      frame False {
      }
      frame True {
        n181 = call "xPCSetParam.vi"("value"=w600, "index"=w598, "port"=w599) -> ()  [unwired: 1 in, 2 out]
      }
    }
    n182 = case shown="真" w528 {
      tunnel: w527 -> [_ w603]
      tunnel: w512 -> [_ w602]
      tunnel: w511 -> [_ w601]
      frame False {
      }
      frame True {
        n183 = call "xPCSetParam.vi"("value"=w603, "index"=w601, "port"=w602) -> ()  [unwired: 1 in, 2 out]
      }
    }
    n184 = case shown="真" w524 {
      tunnel: w523 -> [_ w597]
      tunnel: w504 -> [_ w596]
      tunnel: w503 -> [_ w595]
      frame False {
      }
      frame True {
        n185 = call "xPCSetParam.vi"("value"=w597, "index"=w595, "port"=w596) -> ()  [unwired: 1 in, 2 out]
      }
    }
    n186 = case shown="真" w522 {
      tunnel: w521 -> [_ w594]
      tunnel: w500 -> [_ w593]
      tunnel: w499 -> [_ w592]
      frame False {
      }
      frame True {
        n187 = call "xPCSetParam.vi"("value"=w594, "index"=w592, "port"=w593) -> ()  [unwired: 1 in, 2 out]
      }
    }
    n188 = global read "全局变量.vi" "jieshu"() -> (w582:dbl)
    n189 = Not Equal To 0?(x=w582) -> (x != 0?=w581:bool)
  }
  n190 = while {
    tunnel: w383 -> [w1378]
    tunnel: w382 -> [w1377]
    shift-right: [w1375] -> _
    shift-left: 0.0 -> [w1376]
    tunnel: w380 -> [w639]
    shift-right: [w1371] -> _
    shift-left: 0.0 -> [w1374]
    tunnel: w377 -> [w1370]
    shift-right: [w1367] -> _
    shift-left: 0.0 -> [w1369]
    tunnel: w374 -> [w1365]
    tunnel: w373 -> [w1364]
    shift-right: [w1361] -> _
    shift-left: 0.0 -> [w1363]
    shift-right: [w1357] -> _
    shift-left: 0.0 -> [w1359]
    tunnel: w367 -> [w1355]
    tunnel: w366 -> [w1354]
    shift-right: [w1352] -> _
    shift-left: 0.0 -> [w1353]
    tunnel: w362 -> [w1349]
    tunnel: w361 -> [w1348]
    shift-right: [w1343] -> _
    shift-left: 0.0 -> [w1345]
    tunnel: w356 -> [w1347]
    tunnel: w355 -> [w1346]
    shift-right: [w1337] -> _
    shift-left: 0.0 -> [w1339]
    tunnel: w353 -> [w1341]
    tunnel: w352 -> [w1340]
    shift-right: [w1332] -> _
    shift-left: 0.0 -> [w1335]
    tunnel: w347 -> [w1331]
    tunnel: w346 -> [w1330]
    shift-right: [w1327] -> _
    shift-left: 0.0 -> [w1329]
    tunnel: w342 -> [w1301]
    tunnel: w341 -> [w1326]
    shift-right: [w1320] -> _
    shift-left: 0.0 -> [w1325]
    tunnel: w337 -> [w649]
    tunnel: w336 -> [w1321]
    shift-right: [w1315] -> _
    shift-left: 0.0 -> [w1319]
    tunnel: w332 -> [w1317]
    tunnel: w331 -> [w1316]
    shift-right: [w1309] -> _
    shift-left: 0.0 -> [w1311]
    tunnel: w328 -> [w1313]
    tunnel: w327 -> [w1312]
    shift-right: [w1305] -> _
    shift-left: 0.0 -> [w1307]
    tunnel: w324 -> [w1303]
    tunnel: w323 -> [w1302]
    shift-right: [w1296] -> _
    shift-left: 0.0 -> [w1298]
    tunnel: w318 -> [w1300]
    tunnel: w317 -> [w1299]
    shift-right: [w1291] -> _
    shift-left: 0.0 -> [w1294]
    tunnel: w314 -> [w1290]
    tunnel: w313 -> [w1289]
    shift-right: [w1284] -> _
    shift-left: _ -> [w1286]
    tunnel: w308 -> [w1288]
    tunnel: w307 -> [w1287]
    shift-right: [w1280] -> _
    shift-left: 0.0 -> [w1282]
    tunnel: w303 -> [w1279]
    tunnel: w302 -> [w1278]
    shift-right: [w1272] -> _
    shift-left: 0.0 -> [w1274]
    tunnel: w296 -> [w1276]
    tunnel: w295 -> [w1275]
    shift-right: [w1268] -> _
    shift-left: 0.0 -> [w1270]
    tunnel: w293 -> [w1267]
    tunnel: w292 -> [w1266]
    shift-right: [w1259] -> _
    shift-left: 0.0 -> [w1262]
    tunnel: w289 -> [w1264]
    tunnel: w288 -> [w1263]
    shift-right: [w1254] -> _
    shift-left: 0.0 -> [w1256]
    tunnel: w282 -> [w1258]
    tunnel: w281 -> [w1257]
    shift-right: [w1250] -> _
    shift-left: 0.0 -> [w1252]
    tunnel: w278 -> [w1249]
    tunnel: w277 -> [w1248]
    shift-right: [w1242] -> _
    shift-left: 0.0 -> [w1244]
    tunnel: w272 -> [w1246]
    tunnel: w271 -> [w1245]
    shift-right: [w1236] -> _
    shift-left: 0.0 -> [w1238]
    tunnel: w267 -> [w1240]
    tunnel: w266 -> [w1239]
    shift-right: [w1230] -> _
    shift-left: 0.0 -> [w1232]
    tunnel: w262 -> [w1234]
    tunnel: w261 -> [w1233]
    shift-right: [w1224] -> _
    shift-left: 0.0 -> [w1226]
    tunnel: w257 -> [w1228]
    tunnel: w256 -> [w1227]
    shift-right: [w1218] -> _
    shift-left: 0.0 -> [w1220]
    tunnel: w254 -> [w1222]
    tunnel: w253 -> [w1221]
    shift-right: [w1212] -> _
    shift-left: 0.0 -> [w1214]
    tunnel: w249 -> [w1216]
    tunnel: w248 -> [w1215]
    shift-right: [w1206] -> _
    shift-left: 0.0 -> [w1208]
    tunnel: w242 -> [w1210]
    tunnel: w241 -> [w1209]
    shift-right: [w1200] -> _
    shift-left: 0.0 -> [w1202]
    tunnel: w239 -> [w1204]
    tunnel: w238 -> [w1203]
    shift-right: [w1193] -> _
    shift-left: 0.0 -> [w1196]
    tunnel: w232 -> [w1198]
    tunnel: w231 -> [w1197]
    tunnel: w228 -> [w1192]
    tunnel: w227 -> [w1191]
    tunnel: w225 -> [w1152]
    tunnel: w224 -> [w1151]
    tunnel: w222 -> [w1134]
    tunnel: w221 -> [w1133]
    tunnel: w219 -> [w1118]
    tunnel: w218 -> [w1117]
    shift-right: [w1113] -> _
    shift-left: 0.0 -> [w1115]
    tunnel: w195 -> [w1111]
    tunnel: w194 -> [w1110]
    shift-right: [w1106] -> _
    shift-left: 0.0 -> [w1108]
    tunnel: w96 -> [w1105]
    tunnel: w95 -> [w1104]
    tunnel: w185 -> [w1101]
    tunnel: w184 -> [w1100]
    shift-right: [w1098] -> _
    shift-left: 0.0 -> [w1099]
    tunnel: w168 -> [w1056]
    tunnel: w167 -> [w1055]
    tunnel: w164 -> [w1029]
    tunnel: w163 -> [w1028]
    tunnel: w160 -> [w1002]
    tunnel: w159 -> [w1001]
    tunnel: w156 -> [w975]
    tunnel: w155 -> [w974]
    tunnel: w144 -> [w848]
    tunnel: w143 -> [w847]
    tunnel: w142 -> [w846]
    tunnel: w141 -> [w845]
    tunnel: w140 -> [w844]
    tunnel: w139 -> [w843]
    tunnel: w138 -> [w842]
    tunnel: w137 -> [w841]
    tunnel: w136 -> [w840]
    tunnel: w135 -> [w839]
    tunnel: w120 -> [w663]
    tunnel: w119 -> [w662]
    tunnel: w118 -> [w661]
    tunnel: w117 -> [w660]
    tunnel: w116 -> [w659]
    tunnel: w115 -> [w658]
    tunnel: w114 -> [w657]
    tunnel: w113 -> [w656]
    tunnel: w112 -> [w655]
    tunnel: w111 -> [w654]
    tunnel: w110 -> [w653]
    tunnel: w109 -> [w652]
    tunnel: w108 -> [w651]
    tunnel: w107 -> [w650]
    tunnel: [w649] -> w94
    shift-right: [w642] -> _
    shift-left: 0.0 -> [w643]
    tunnel: w87 -> [w641]
    tunnel: w86 -> [w640]
    tunnel: w7 -> [w638]
    tunnel: w6 -> [w637]
    stop <- w646 stop-if-true
    n191 = for {
      tunnel: [w1386] -> w664 mode=indexing
      tunnel: w663 -> [w1385] mode=indexing
      tunnel: w662 -> [w1384] mode=indexing
      n192 = call "xPCGetSignal.vi"("signal"=w1384, "port"=w1385) -> ("Output Value"=w1386:dbl)  [unwired: 1 in, 2 out]
    }
    n193 = for {
      tunnel: [w1401] -> w789 mode=indexing
      tunnel: w653 -> [w1400] mode=indexing
      tunnel: w652 -> [w1399] mode=indexing
      n194 = call "xPCGetSignal.vi"("signal"=w1399, "port"=w1400) -> ("Output Value"=w1401:dbl)  [unwired: 1 in, 2 out]
    }
    n195 = for {
      tunnel: [w1410] -> w874 mode=indexing
      tunnel: w842 -> [w1409] mode=indexing
      tunnel: w841 -> [w1408] mode=indexing
      n196 = call "xPCGetSignal.vi"("signal"=w1408, "port"=w1409) -> ("Output Value"=w1410:dbl)  [unwired: 1 in, 2 out]
    }
    n197 = for {
      tunnel: [w1407] -> w849 mode=indexing
      tunnel: w840 -> [w1406] mode=indexing
      tunnel: w839 -> [w1405] mode=indexing
      n198 = call "xPCGetSignal.vi"("signal"=w1405, "port"=w1406) -> ("Output Value"=w1407:dbl)  [unwired: 1 in, 2 out]
    }
    n199 = for {
      tunnel: [w1404] -> w814 mode=indexing
      tunnel: w651 -> [w1403] mode=indexing
      tunnel: w650 -> [w1402] mode=indexing
      n200 = call "xPCGetSignal.vi"("signal"=w1402, "port"=w1403) -> ("Output Value"=w1404:dbl)  [unwired: 1 in, 2 out]
    }
    n201 = for {
      tunnel: [w1419] -> w949 mode=indexing
      tunnel: w848 -> [w1418] mode=indexing
      tunnel: w847 -> [w1417] mode=indexing
      n202 = call "xPCGetSignal.vi"("signal"=w1417, "port"=w1418) -> ("Output Value"=w1419:dbl)  [unwired: 1 in, 2 out]
    }
    n203 = for {
      tunnel: [w1422] -> w976 mode=indexing
      tunnel: w975 -> [w1421] mode=indexing
      tunnel: w974 -> [w1420] mode=indexing
      n204 = call "xPCGetSignal.vi"("signal"=w1420, "port"=w1421) -> ("Output Value"=w1422:dbl)  [unwired: 1 in, 2 out]
    }
    n205 = for {
      tunnel: [w1389] -> w689 mode=indexing
      tunnel: w661 -> [w1388] mode=indexing
      tunnel: w660 -> [w1387] mode=indexing
      n206 = call "xPCGetSignal.vi"("signal"=w1387, "port"=w1388) -> ("Output Value"=w1389:dbl)  [unwired: 1 in, 2 out]
    }
    n207 = for {
      tunnel: [w1428] -> w1030 mode=indexing
      tunnel: w1029 -> [w1427] mode=indexing
      tunnel: w1028 -> [w1426] mode=indexing
      n208 = call "xPCGetSignal.vi"("signal"=w1426, "port"=w1427) -> ("Output Value"=w1428:dbl)  [unwired: 1 in, 2 out]
    }
    n209 = for {
      tunnel: [w1416] -> w924 mode=indexing
      tunnel: w846 -> [w1415] mode=indexing
      tunnel: w845 -> [w1414] mode=indexing
      n210 = call "xPCGetSignal.vi"("signal"=w1414, "port"=w1415) -> ("Output Value"=w1416:dbl)  [unwired: 1 in, 2 out]
    }
    n211 = Wait (ms)(milliseconds to wait=u32 40 ("等待时间（毫秒）")) -> ()  [unwired: 1 out]
    n212 = for {
      tunnel: [w1431] -> w1057 mode=indexing
      tunnel: w1056 -> [w1430] mode=indexing
      tunnel: w1055 -> [w1429] mode=indexing
      n213 = call "xPCGetSignal.vi"("signal"=w1429, "port"=w1430) -> ("Output Value"=w1431:dbl)  [unwired: 1 in, 2 out]
    }
    n214 = for {
      tunnel: [w1398] -> w764 mode=indexing
      tunnel: w655 -> [w1397] mode=indexing
      tunnel: w654 -> [w1396] mode=indexing
      n215 = call "xPCGetSignal.vi"("signal"=w1396, "port"=w1397) -> ("Output Value"=w1398:dbl)  [unwired: 1 in, 2 out]
    }
    n216 = for {
      tunnel: [w1395] -> w739 mode=indexing
      tunnel: w657 -> [w1394] mode=indexing
      tunnel: w656 -> [w1393] mode=indexing
      n217 = call "xPCGetSignal.vi"("signal"=w1393, "port"=w1394) -> ("Output Value"=w1395:dbl)  [unwired: 1 in, 2 out]
    }
    n218 = for {
      tunnel: [w1392] -> w714 mode=indexing
      tunnel: w659 -> [w1391] mode=indexing
      tunnel: w658 -> [w1390] mode=indexing
      n219 = call "xPCGetSignal.vi"("signal"=w1390, "port"=w1391) -> ("Output Value"=w1392:dbl)  [unwired: 1 in, 2 out]
    }
    n220 = for {
      tunnel: [w1413] -> w899 mode=indexing
      tunnel: w844 -> [w1412] mode=indexing
      tunnel: w843 -> [w1411] mode=indexing
      n221 = call "xPCGetSignal.vi"("signal"=w1411, "port"=w1412) -> ("Output Value"=w1413:dbl)  [unwired: 1 in, 2 out]
    }
    n222 = for {
      tunnel: [w1425] -> w1003 mode=indexing
      tunnel: w1002 -> [w1424] mode=indexing
      tunnel: w1001 -> [w1423] mode=indexing
      n223 = call "xPCGetSignal.vi"("signal"=w1423, "port"=w1424) -> ("Output Value"=w1425:dbl)  [unwired: 1 in, 2 out]
    }
    n224 = global read "全局变量.vi" "tiaoshimoshi"() -> (w642:dbl)
    n225 = Index Array(array=w664, index=2 ("索引")) -> (element=w679:dbl)
    n226 = Index Array(array=w789, index=2 ("索引")) -> (element=w804:dbl)
    n227 = Index Array(array=w874, index=2 ("索引")) -> (element=w889:dbl)
    n228 = Index Array(array=w664, index=3 ("索引")) -> (element=w675:dbl)
    n229 = Index Array(array=w789, index=3 ("索引")) -> (element=w800:dbl)
    n230 = Index Array(array=w664, index=1 ("索引")) -> (element=w683:dbl)
    n231 = Index Array(array=w789, index=1 ("索引")) -> (element=w808:dbl)
    n232 = Index Array(array=w664, index=0 ("索引")) -> (element=w687:dbl)
    n233 = Index Array(array=w874, index=3 ("索引")) -> (element=w885:dbl)
    n234 = Index Array(array=w789, index=0 ("索引")) -> (element=w812:dbl)
    n235 = Index Array(array=w874, index=1 ("索引")) -> (element=w893:dbl)
    n236 = Index Array(array=w849, index=2 ("索引")) -> (element=w864:dbl)
    n237 = Index Array(array=w874, index=0 ("索引")) -> (element=w897:dbl)
    n238 = Index Array(array=w664, index=4 ("索引")) -> (element=w671:dbl)
    n239 = Index Array(array=w789, index=4 ("索引")) -> (element=w796:dbl)
    n240 = Index Array(array=w849, index=3 ("索引")) -> (element=w860:dbl)
    n241 = Index Array(array=w874, index=4 ("索引")) -> (element=w881:dbl)
    n242 = Index Array(array=w849, index=1 ("索引")) -> (element=w868:dbl)
    n243 = Index Array(array=w814, index=2 ("索引")) -> (element=w829:dbl)
    n244 = Index Array(array=w849, index=0 ("索引")) -> (element=w872:dbl)
    n245 = Index Array(array=w949, index=2 ("索引")) -> (element=w964:dbl)
    n246 = Index Array(array=w814, index=3 ("索引")) -> (element=w825:dbl)
    n247 = Index Array(array=w849, index=4 ("索引")) -> (element=w856:dbl)
    n248 = Index Array(array=w814, index=1 ("索引")) -> (element=w833:dbl)
    n249 = Index Array(array=w976, index=2 ("索引")) -> (element=w991:dbl)
    n250 = Index Array(array=w949, index=3 ("索引")) -> (element=w960:dbl)
    n251 = Index Array(array=w814, index=0 ("索引")) -> (element=w837:dbl)
    n252 = Index Array(array=w949, index=1 ("索引")) -> (element=w968:dbl)
    n253 = Index Array(array=w949, index=0 ("索引")) -> (element=w972:dbl)
    n254 = Index Array(array=w689, index=2 ("索引")) -> (element=w704:dbl)
    n255 = Index Array(array=w976, index=3 ("索引")) -> (element=w987:dbl)
    n256 = Index Array(array=w814, index=4 ("索引")) -> (element=w821:dbl)
    n257 = Index Array(array=w976, index=1 ("索引")) -> (element=w995:dbl)
    n258 = Index Array(array=w1030, index=2 ("索引")) -> (element=w1045:dbl)
    n259 = Index Array(array=w976, index=0 ("索引")) -> (element=w999:dbl)
    n260 = Index Array(array=w949, index=4 ("索引")) -> (element=w956:dbl)
    n261 = Index Array(array=w689, index=3 ("索引")) -> (element=w700:dbl)
    n262 = Index Array(array=w689, index=1 ("索引")) -> (element=w708:dbl)
    n263 = Index Array(array=w689, index=0 ("索引")) -> (element=w712:dbl)
    n264 = Index Array(array=w1030, index=3 ("索引")) -> (element=w1041:dbl)
    n265 = Index Array(array=w976, index=4 ("索引")) -> (element=w983:dbl)
    n266 = Index Array(array=w1030, index=1 ("索引")) -> (element=w1049:dbl)
    n267 = Index Array(array=w1030, index=0 ("索引")) -> (element=w1053:dbl)
    n268 = Index Array(array=w689, index=4 ("索引")) -> (element=w696:dbl)
    n269 = Index Array(array=w1030, index=4 ("索引")) -> (element=w1037:dbl)
    n270 = Index Array(array=w924, index=2 ("索引")) -> (element=w939:dbl)
    n271 = Index Array(array=w1057, index=2 ("索引")) -> (element=w1072:dbl)
    n272 = Index Array(array=w924, index=3 ("索引")) -> (element=w935:dbl)
    n273 = Index Array(array=w924, index=1 ("索引")) -> (element=w943:dbl)
    n274 = Index Array(array=w1057, index=3 ("索引")) -> (element=w1068:dbl)
    n275 = Index Array(array=w924, index=0 ("索引")) -> (element=w947:dbl)
    n276 = Index Array(array=w1057, index=1 ("索引")) -> (element=w1076:dbl)
    n277 = Index Array(array=w1057, index=0 ("索引")) -> (element=w1080:dbl)
    n278 = Index Array(array=w764, index=2 ("索引")) -> (element=w779:dbl)
    n279 = Index Array(array=w924, index=4 ("索引")) -> (element=w931:dbl)
    n280 = Index Array(array=w739, index=2 ("索引")) -> (element=w754:dbl)
    n281 = Index Array(array=w1057, index=4 ("索引")) -> (element=w1064:dbl)
    n282 = Index Array(array=w764, index=3 ("索引")) -> (element=w775:dbl)
    n283 = Index Array(array=w764, index=1 ("索引")) -> (element=w783:dbl)
    n284 = Index Array(array=w739, index=3 ("索引")) -> (element=w750:dbl)
    n285 = Index Array(array=w764, index=0 ("索引")) -> (element=w787:dbl)
    n286 = Index Array(array=w739, index=1 ("索引")) -> (element=w758:dbl)
    n287 = Index Array(array=w739, index=0 ("索引")) -> (element=w762:dbl)
    n288 = Index Array(array=w764, index=4 ("索引")) -> (element=w771:dbl)
    n289 = Index Array(array=w739, index=4 ("索引")) -> (element=w746:dbl)
    n290 = Index Array(array=w714, index=2 ("索引")) -> (element=w729:dbl)
    n291 = global read "全局变量.vi" "sds6"() -> (w1375:dbl)
    n292 = Index Array(array=w714, index=3 ("索引")) -> (element=w725:dbl)
    n293 = Index Array(array=w899, index=2 ("索引")) -> (element=w914:dbl)
    n294 = Index Array(array=w714, index=1 ("索引")) -> (element=w733:dbl)
    n295 = Index Array(array=w714, index=0 ("索引")) -> (element=w737:dbl)
    n296 = Index Array(array=w899, index=3 ("索引")) -> (element=w910:dbl)
    n297 = Index Array(array=w899, index=1 ("索引")) -> (element=w918:dbl)
    n298 = Index Array(array=w714, index=4 ("索引")) -> (element=w721:dbl)
    n299 = Index Array(array=w899, index=0 ("索引")) -> (element=w922:dbl)
    n300 = Index Array(array=w899, index=4 ("索引")) -> (element=w906:dbl)
    n301 = Index Array(array=w1003, index=2 ("索引")) -> (element=w1018:dbl)
    n302 = Index Array(array=w1003, index=3 ("索引")) -> (element=w1014:dbl)
    n303 = Index Array(array=w1003, index=1 ("索引")) -> (element=w1022:dbl)
    n304 = Index Array(array=w1003, index=0 ("索引")) -> (element=w1026:dbl)
    n305 = Equal?(x=w679, y=1.0) -> (x = y?=w677:bool)
    n306 = Index Array(array=w1003, index=4 ("索引")) -> (element=w1010:dbl)
    n307 = Equal?(x=w804, y=1.0) -> (x = y?=w802:bool)
    n308 = Equal?(x=w889, y=1.0) -> (x = y?=w887:bool)
    n309 = Equal?(x=w675, y=1.0) -> (x = y?=w673:bool)
    n310 = Equal?(x=w800, y=1.0) -> (x = y?=w798:bool)
    n311 = Equal?(x=w683, y=1.0) -> (x = y?=w681:bool)
    n312 = Equal?(x=w808, y=1.0) -> (x = y?=w806:bool)
    n313 = Equal?(x=w687, y=1.0) -> (x = y?=w685:bool)
    n314 = global read "全局变量.vi" "sds4"() -> (w1367:dbl)
    n315 = Equal?(x=w885, y=1.0) -> (x = y?=w883:bool)
    n316 = Equal?(x=w812, y=1.0) -> (x = y?=w810:bool)
    n317 = global read "全局变量.vi" "sds5"() -> (w1371:dbl)
    n318 = Equal?(x=w893, y=1.0) -> (x = y?=w891:bool)
    n319 = Equal?(x=w864, y=1.0) -> (x = y?=w862:bool)
    n320 = Equal?(x=w897, y=1.0) -> (x = y?=w895:bool)
    n321 = Equal?(x=w671, y=1.0) -> (x = y?=w669:bool)
    n322 = Equal?(x=w796, y=1.0) -> (x = y?=w794:bool)
    n323 = Equal?(x=w860, y=1.0) -> (x = y?=w858:bool)
    n324 = Equal?(x=w881, y=1.0) -> (x = y?=w879:bool)
    n325 = Equal?(x=w868, y=1.0) -> (x = y?=w866:bool)
    n326 = Equal?(x=w829, y=1.0) -> (x = y?=w827:bool)
    n327 = Equal?(x=w872, y=1.0) -> (x = y?=w870:bool)
    n328 = global read "全局变量.vi" "sds2"() -> (w1357:dbl)
    n329 = Equal?(x=w964, y=1.0) -> (x = y?=w962:bool)
    n330 = global read "全局变量.vi" "sds1"() -> (w1352:dbl)
    n331 = Equal?(x=w825, y=1.0) -> (x = y?=w823:bool)
    n332 = Equal?(x=w856, y=1.0) -> (x = y?=w854:bool)
    n333 = Equal?(x=w833, y=1.0) -> (x = y?=w831:bool)
    n334 = Equal?(x=w991, y=1.0) -> (x = y?=w989:bool)
    n335 = Equal?(x=w960, y=1.0) -> (x = y?=w958:bool)
    n336 = Equal?(x=w837, y=1.0) -> (x = y?=w835:bool)
    n337 = Equal?(x=w968, y=1.0) -> (x = y?=w966:bool)
    n338 = Equal?(x=w972, y=1.0) -> (x = y?=w970:bool)
    n339 = Equal?(x=w704, y=1.0) -> (x = y?=w702:bool)
    n340 = Equal?(x=w987, y=1.0) -> (x = y?=w985:bool)
    n341 = Equal?(x=w821, y=1.0) -> (x = y?=w819:bool)
    n342 = Equal?(x=w995, y=1.0) -> (x = y?=w993:bool)
    n343 = Equal?(x=w1045, y=1.0) -> (x = y?=w1043:bool)
    n344 = Equal?(x=w999, y=1.0) -> (x = y?=w997:bool)
    n345 = Equal?(x=w956, y=1.0) -> (x = y?=w954:bool)
    n346 = Equal?(x=w700, y=1.0) -> (x = y?=w698:bool)
    n347 = Equal?(x=w708, y=1.0) -> (x = y?=w706:bool)
    n348 = global read "全局变量.vi" "qiehuan"() -> (w1098:dbl)
    n349 = Equal?(x=w712, y=1.0) -> (x = y?=w710:bool)
    n350 = Equal?(x=w1041, y=1.0) -> (x = y?=w1039:bool)
    n351 = Equal?(x=w983, y=1.0) -> (x = y?=w981:bool)
    n352 = Equal?(x=w1049, y=1.0) -> (x = y?=w1047:bool)
    n353 = Equal?(x=w1053, y=1.0) -> (x = y?=w1051:bool)
    n354 = Equal?(x=w696, y=1.0) -> (x = y?=w694:bool)
    n355 = Equal?(x=w1037, y=1.0) -> (x = y?=w1035:bool)
    n356 = Equal?(x=w939, y=1.0) -> (x = y?=w937:bool)
    n357 = global read "全局变量.vi" "sds8"() -> (w1106:dbl)
    n358 = Equal?(x=w1072, y=1.0) -> (x = y?=w1070:bool)
    n359 = Equal?(x=w935, y=1.0) -> (x = y?=w933:bool)
    n360 = Equal?(x=w943, y=1.0) -> (x = y?=w941:bool)
    n361 = global read "全局变量.vi" "sds7"() -> (w1113:dbl)
    n362 = Equal?(x=w1068, y=1.0) -> (x = y?=w1066:bool)
    n363 = Equal?(x=w947, y=1.0) -> (x = y?=w945:bool)
    n364 = Equal?(x=w1076, y=1.0) -> (x = y?=w1074:bool)
    n365 = Equal?(x=w1080, y=1.0) -> (x = y?=w1078:bool)
    n366 = Equal?(x=w779, y=1.0) -> (x = y?=w777:bool)
    n367 = Equal?(x=w931, y=1.0) -> (x = y?=w929:bool)
    n368 = Equal?(x=w754, y=1.0) -> (x = y?=w752:bool)
    n369 = Equal?(x=w1064, y=1.0) -> (x = y?=w1062:bool)
    n370 = Equal?(x=w775, y=1.0) -> (x = y?=w773:bool)
    n371 = Equal?(x=w783, y=1.0) -> (x = y?=w781:bool)
    n372 = Equal?(x=w750, y=1.0) -> (x = y?=w748:bool)
    n373 = global read "全局变量.vi" "suoding"() -> (w1327:dbl)
    n374 = global read "全局变量.vi" "kaigai"() -> (w1320:dbl)
    n375 = Equal?(x=w787, y=1.0) -> (x = y?=w785:bool)
    n376 = Equal?(x=w758, y=1.0) -> (x = y?=w756:bool)
    n377 = Equal?(x=w762, y=1.0) -> (x = y?=w760:bool)
    n378 = global read "全局变量.vi" "sds3"() -> (w1361:dbl)
    n379 = Equal?(x=w771, y=1.0) -> (x = y?=w769:bool)
    n380 = Equal?(x=w746, y=1.0) -> (x = y?=w744:bool)
    n381 = Equal?(x=w729, y=1.0) -> (x = y?=w727:bool)
    n382 = global read "全局变量.vi" "songkai"() -> (w1315:dbl)
    n383 = global read "全局变量.vi" "guangai"() -> (w1337:dbl)
    n384 = Equal?(x=w725, y=1.0) -> (x = y?=w723:bool)
    n385 = Equal?(x=w914, y=1.0) -> (x = y?=w912:bool)
    n386 = Equal?(x=w733, y=1.0) -> (x = y?=w731:bool)
    n387 = global read "全局变量.vi" "jiesuo"() -> (w1332:dbl)
    n388 = Equal?(x=w737, y=1.0) -> (x = y?=w735:bool)
    n389 = global read "全局变量.vi" "Switch2"() -> (w1309:dbl)
    n390 = Equal?(x=w910, y=1.0) -> (x = y?=w908:bool)
    n391 = Equal?(x=w918, y=1.0) -> (x = y?=w916:bool)
    n392 = Equal?(x=w721, y=1.0) -> (x = y?=w719:bool)
    n393 = Equal?(x=w922, y=1.0) -> (x = y?=w920:bool)
    n394 = Equal?(x=w906, y=1.0) -> (x = y?=w904:bool)
    n395 = global write "全局变量.vi" "sd锁定异常"(w677) -> ()
    n396 = global write "全局变量.vi" "sd锁定异常"(w802) -> ()
    n397 = Equal?(x=w1018, y=1.0) -> (x = y?=w1016:bool)
    n398 = global write "全局变量.vi" "sd解锁异常"(w673) -> ()
    n399 = global write "全局变量.vi" "sd解锁异常"(w798) -> ()
    n400 = global write "全局变量.vi" "sd开盖异常"(w681) -> ()
    n401 = Equal?(x=w1014, y=1.0) -> (x = y?=w1012:bool)
    n402 = global write "全局变量.vi" "zd锁定异常"(w887) -> ()
    n403 = global write "全局变量.vi" "sd开盖异常"(w806) -> ()
    n404 = Equal?(x=w1022, y=1.0) -> (x = y?=w1020:bool)
    n405 = global write "全局变量.vi" "zd解锁异常"(w883) -> ()
    n406 = Equal?(x=w1026, y=1.0) -> (x = y?=w1024:bool)
    n407 = global write "全局变量.vi" "zd开盖异常"(w891) -> ()
    n408 = global write "全局变量.vi" "sd锁定异常"(w862) -> ()
    n409 = global write "全局变量.vi" "sd松开异常"(w685) -> ()
    n410 = Not Equal?(x=w643, y=w642) -> (x != y?=w644:bool)
    n411 = global write "全局变量.vi" "sd松开异常"(w810) -> ()
    n412 = global write "全局变量.vi" "sd关盖异常"(w669) -> ()
    n413 = global read "全局变量.vi" "yajin"() -> (w1343:dbl)
    n414 = global write "全局变量.vi" "sd关盖异常"(w794) -> ()
    n415 = Equal?(x=w1010, y=1.0) -> (x = y?=w1008:bool)
    n416 = global write "全局变量.vi" "zd松开异常"(w895) -> ()
    n417 = global write "全局变量.vi" "sd解锁异常"(w858) -> ()
    n418 = global write "全局变量.vi" "zd关盖异常"(w879) -> ()
    n419 = global write "全局变量.vi" "sd开盖异常"(w866) -> ()
    n420 = global write "全局变量.vi" "sd锁定异常"(w827) -> ()
    n421 = global read "全局变量.vi" "Switch1"() -> (w1305:dbl)
    n422 = global write "全局变量.vi" "sd松开异常"(w870) -> ()
    n423 = global write "全局变量.vi" "sd解锁异常"(w823) -> ()
    n424 = global write "全局变量.vi" "zd锁定异常"(w962) -> ()
    n425 = global write "全局变量.vi" "sd关盖异常"(w854) -> ()
    n426 = global write "全局变量.vi" "sd开盖异常"(w831) -> ()
    n427 = global write "全局变量.vi" "zd解锁异常"(w958) -> ()
    n428 = global write "全局变量.vi" "zd开盖异常"(w966) -> ()
    n429 = for {
      tunnel: [w1443] -> w1082 mode=indexing
      tunnel: w1118 -> [w1442] mode=indexing
      tunnel: w1117 -> [w1441] mode=indexing
      n430 = call "xPCGetSignal.vi"("signal"=w1441, "port"=w1442) -> ("Output Value"=w1443:dbl)  [unwired: 1 in, 2 out]
    }
    n431 = global write "全局变量.vi" "zd锁定异常"(w989) -> ()
    n432 = global write "全局变量.vi" "sd松开异常"(w835) -> ()
    n433 = global write "全局变量.vi" "sd锁定异常"(w702) -> ()
    n434 = for {
      tunnel: [w1446] -> w1119 mode=indexing
      tunnel: w1134 -> [w1445] mode=indexing
      tunnel: w1133 -> [w1444] mode=indexing
      n435 = call "xPCGetSignal.vi"("signal"=w1444, "port"=w1445) -> ("Output Value"=w1446:dbl)  [unwired: 1 in, 2 out]
    }
    n436 = global write "全局变量.vi" "zd解锁异常"(w985) -> ()
    n437 = global write "全局变量.vi" "sd关盖异常"(w819) -> ()
    n438 = global write "全局变量.vi" "zd开盖异常"(w993) -> ()
    n439 = global write "全局变量.vi" "zd松开异常"(w970) -> ()
    n440 = global write "全局变量.vi" "zd关盖异常"(w954) -> ()
    n441 = global write "全局变量.vi" "sd解锁异常"(w698) -> ()
    n442 = global write "全局变量.vi" "sd开盖异常"(w706) -> ()
    n443 = global write "全局变量.vi" "zd锁定异常"(w1043) -> ()
    n444 = global write "全局变量.vi" "zd松开异常"(w997) -> ()
    n445 = global write "全局变量.vi" "zd解锁异常"(w1039) -> ()
    n446 = global write "全局变量.vi" "zd关盖异常"(w981) -> ()
    n447 = global write "全局变量.vi" "zd开盖异常"(w1047) -> ()
    n448 = global write "全局变量.vi" "sd松开异常"(w710) -> ()
    n449 = global write "全局变量.vi" "sd关盖异常"(w694) -> ()
    n450 = global write "全局变量.vi" "zd松开异常"(w1051) -> ()
    n451 = global write "全局变量.vi" "zd关盖异常"(w1035) -> ()
    n452 = Build Array(w642) -> (w645:dbl[])
    n453 = global read "全局变量.vi" "zds8"() -> (w1212:dbl)
    n454 = global write "全局变量.vi" "zd锁定异常"(w937) -> ()
    n455 = global write "全局变量.vi" "zd解锁异常"(w933) -> ()
    n456 = global write "全局变量.vi" "zd锁定异常"(w1070) -> ()
    n457 = global write "全局变量.vi" "zd开盖异常"(w941) -> ()
    n458 = global write "全局变量.vi" "zd解锁异常"(w1066) -> ()
    n459 = for {
      tunnel: [w1449] -> w1135 mode=indexing
      tunnel: w1152 -> [w1448] mode=indexing
      tunnel: w1151 -> [w1447] mode=indexing
      n460 = call "xPCGetSignal.vi"("signal"=w1447, "port"=w1448) -> ("Output Value"=w1449:dbl)  [unwired: 1 in, 2 out]
    }
    n461 = global write "全局变量.vi" "zd开盖异常"(w1074) -> ()
    n462 = global write "全局变量.vi" "zd松开异常"(w945) -> ()
    n463 = global write "全局变量.vi" "sd锁定异常"(w777) -> ()
    n464 = global write "全局变量.vi" "zd关盖异常"(w929) -> ()
    n465 = global write "全局变量.vi" "sd锁定异常"(w752) -> ()
    n466 = global write "全局变量.vi" "zd松开异常"(w1078) -> ()
    n467 = global write "全局变量.vi" "zd关盖异常"(w1062) -> ()
    n468 = global write "全局变量.vi" "sd解锁异常"(w773) -> ()
    n469 = global write "全局变量.vi" "sd开盖异常"(w781) -> ()
    n470 = global write "全局变量.vi" "sd解锁异常"(w748) -> ()
    n471 = global write "全局变量.vi" "sd开盖异常"(w756) -> ()
    n472 = global write "全局变量.vi" "sd松开异常"(w785) -> ()
    n473 = global write "全局变量.vi" "sd关盖异常"(w769) -> ()
    n474 = global write "全局变量.vi" "sd松开异常"(w760) -> ()
    n475 = global write "全局变量.vi" "sd关盖异常"(w744) -> ()
    n476 = global write "全局变量.vi" "sd锁定异常"(w727) -> ()
    n477 = Not Equal?(x=w1374, y=w1371) -> (x != y?=w1373:bool)
    n478 = global read "全局变量.vi" "zds7"() -> (w1218:dbl)
    n479 = global write "全局变量.vi" "sd解锁异常"(w723) -> ()
    n480 = Not Equal?(x=w1108, y=w1106) -> (x != y?=w1107:bool)
    n481 = global read "全局变量.vi" "t3"() -> (w1280:dbl)
    n482 = global write "全局变量.vi" "sd开盖异常"(w731) -> ()
    n483 = global read "全局变量.vi" "t1"() -> (w1291:dbl)
    n484 = global write "全局变量.vi" "zd锁定异常"(w912) -> ()
    n485 = Build Array(w1371) -> (w1372:dbl[])
    n486 = global write "全局变量.vi" "zd解锁异常"(w908) -> ()
    n487 = global write "全局变量.vi" "sd松开异常"(w735) -> ()
    n488 = global write "全局变量.vi" "zd开盖异常"(w916) -> ()
    n489 = global write "全局变量.vi" "sd关盖异常"(w719) -> ()
    n490 = global read "全局变量.vi" "zds4"() -> (w1236:dbl)
    n491 = Not Equal?(x=w1369, y=w1367) -> (x != y?=w1366:bool)
    n492 = global write "全局变量.vi" "zd松开异常"(w920) -> ()
    n493 = Build Array(w1375) -> (w1379:dbl[])
    n494 = global write "全局变量.vi" "zd关盖异常"(w904) -> ()
    n495 = Not Equal?(x=w1099, y=w1098) -> (x != y?=w1103:bool)
    n496 = Build Array(w1367) -> (w1368:dbl[])
    n497 = global read "全局变量.vi" "Switch"() -> (w1296:dbl)
    n498 = global read "全局变量.vi" "zds6"() -> (w1224:dbl)
    n499 = global write "全局变量.vi" "zd锁定异常"(w1016) -> ()
    n500 = global read "全局变量.vi" "t4"() -> (w1272:dbl)
    n501 = global write "全局变量.vi" "zd解锁异常"(w1012) -> ()
    n502 = Not Equal?(x=w1353, y=w1352) -> (x != y?=w1350:bool)
    n503 = global write "全局变量.vi" "zd开盖异常"(w1020) -> ()
    n504 = Not Equal?(x=w1376, y=w1375) -> (x != y?=w1380:bool)
    n505 = Not Equal?(x=w1363, y=w1361) -> (x != y?=w1362:bool)
    n506 = global read "全局变量.vi" "t5"() -> (w1268:dbl)
    n507 = global write "全局变量.vi" "zd松开异常"(w1024) -> ()
    n508 = global read "全局变量.vi" "t2"() -> (w1284:dbl)
    n509 = global write "全局变量.vi" "zd关盖异常"(w1008) -> ()
    n510 = Build Array(w1106) -> (w1109:dbl[])
    n511 = global read "全局变量.vi" "zds5"() -> (w1230:dbl)
    n512 = Build Array(w1361) -> (w1360:dbl[])
    n513 = Not Equal?(x=w1115, y=w1113) -> (x != y?=w1112:bool)
    n514 = global read "全局变量.vi" "zds1"() -> (w1254:dbl)
    n515 = global read "全局变量.vi" "zds3"() -> (w1242:dbl)
    n516 = global read "全局变量.vi" "zds2"() -> (w1250:dbl)
    n517 = for {
      tunnel: [w1452] -> w1153 mode=indexing
      tunnel: w1192 -> [w1451] mode=indexing
      tunnel: w1191 -> [w1450] mode=indexing
      n518 = call "xPCGetSignal.vi"("signal"=w1450, "port"=w1451) -> ("Output Value"=w1452:dbl)  [unwired: 1 in, 2 out]
    }
    n519 = Build Array(w1352) -> (w1351:dbl[])
    n520 = global read "全局变量.vi" "t6"() -> (w1259:dbl)
    n521 = global read "全局变量.vi" "jieshu"() -> (w1206:dbl)
    n522 = Not Equal?(x=w1359, y=w1357) -> (x != y?=w1358:bool)
    n523 = global read "全局变量.vi" "start"() -> (w1193:dbl)
    n524 = Build Array(w1357) -> (w1356:dbl[])
    n525 = global read "全局变量.vi" "kaigaicishu"() -> (w1200:dbl)
    n526 = Build Array(w1113) -> (w1114:dbl[])
    n527 = Not Equal?(x=w1345, y=w1343) -> (x != y?=w1344:bool)
    n528 = Not Equal?(x=w1339, y=w1337) -> (x != y?=w1338:bool)
    n529 = Build Array(w1343) -> (w1342:dbl[])
    n530 = Not Equal?(x=w1335, y=w1332) -> (x != y?=w1334:bool)
    n531 = case shown="真" w644 {
      tunnel: w645 -> [_ w1383]
      tunnel: w641 -> [_ w1382]
      tunnel: w640 -> [_ w1381]
      frame False {
      }
      frame True {
        n532 = call "xPCSetParam.vi"("value"=w1383, "index"=w1381, "port"=w1382) -> ()  [unwired: 1 in, 2 out]
      }
    }
    n533 = Build Array(w1332) -> (w1333:dbl[])
    n534 = Build Array(w1337) -> (w1336:dbl[])
    n535 = Build Array(w1098) -> (w1102:dbl[])
    n536 = Not Equal?(x=w1329, y=w1327) -> (x != y?=w1328:bool)
    n537 = Build Array(w1327) -> (w1323:dbl[])
    n538 = Not Equal?(x=w1319, y=w1315) -> (x != y?=w1318:bool)
    n539 = Not Equal?(x=w1320, y=w1325) -> (x != y?=w1324:bool)
    n540 = Not Equal?(x=w1282, y=w1280) -> (x != y?=w1281:bool)
    n541 = Not Equal?(x=w1270, y=w1268) -> (x != y?=w1269:bool)
    n542 = Not Equal?(x=w1294, y=w1291) -> (x != y?=w1293:bool)
    n543 = Not Equal?(x=w1307, y=w1305) -> (x != y?=w1306:bool)
    n544 = Build Array(w1320) -> (w1322:dbl[])
    n545 = Not Equal?(x=w1311, y=w1309) -> (x != y?=w1310:bool)
    n546 = Build Array(w1309) -> (w1308:dbl[])
    n547 = Not Equal?(x=w1274, y=w1272) -> (x != y?=w1273:bool)
    n548 = Build Array(w1315) -> (w1314:dbl[])
    n549 = Not Equal?(x=w1262, y=w1259) -> (x != y?=w1261:bool)
    n550 = Not Equal?(x=w1286, y=w1284) -> (x != y?=w1285:bool)
    n551 = case shown="真" w1358 {
      tunnel: w1356 -> [_ w1536]
      tunnel: w1355 -> [_ w1535]
      tunnel: w1354 -> [_ w1534]
      frame False {
      }
      frame True {
        n552 = call "xPCSetParam.vi"("value"=w1536, "index"=w1534, "port"=w1535) -> ()  [unwired: 1 in, 2 out]
      }
    }
    n553 = Not Equal?(x=w1298, y=w1296) -> (x != y?=w1297:bool)
    n554 = case shown="真" w1350 {
      tunnel: w1351 -> [_ w1533]
      tunnel: w1349 -> [_ w1532]
      tunnel: w1348 -> [_ w1531]
      frame False {
      }
      frame True {
        n555 = call "xPCSetParam.vi"("value"=w1533, "index"=w1531, "port"=w1532) -> ()  [unwired: 1 in, 2 out]
      }
    }
    n556 = Not Equal?(x=w1196, y=w1193) -> (x != y?=w1195:bool)
    n557 = Build Array(w1305) -> (w1304:dbl[])
    n558 = Not Equal?(x=w1238, y=w1236) -> (x != y?=w1237:bool)
    n559 = case shown="真" w1373 {
      tunnel: w639 -> [_ w1545]
      tunnel: w1372 -> [_ w1544]
      tunnel: w1370 -> [_ w1543]
      frame False {
      }
      frame True {
        n560 = call "xPCSetParam.vi"("value"=w1544, "index"=w1543, "port"=w1545) -> ()  [unwired: 1 in, 2 out]
      }
    }
    n561 = case shown="真" w1366 {
      tunnel: w1368 -> [_ w1542]
      tunnel: w1365 -> [_ w1541]
      tunnel: w1364 -> [_ w1540]
      frame False {
      }
      frame True {
        n562 = call "xPCSetParam.vi"("value"=w1542, "index"=w1540, "port"=w1541) -> ()  [unwired: 1 in, 2 out]
      }
    }
    n563 = Not Equal?(x=w1244, y=w1242) -> (x != y?=w1243:bool)
    n564 = case shown="真" w1380 {
      tunnel: w1379 -> [_ w1548]
      tunnel: w1378 -> [_ w1547]
      tunnel: w1377 -> [_ w1546]
      frame False {
      }
      frame True {
        n565 = call "xPCSetParam.vi"("value"=w1548, "index"=w1546, "port"=w1547) -> ()  [unwired: 1 in, 2 out]
      }
    }
    n566 = Not Equal?(x=w1202, y=w1200) -> (x != y?=w1201:bool)
    n567 = Build Array(w1291) -> (w1292:dbl[])
    n568 = Not Equal?(x=w1232, y=w1230) -> (x != y?=w1231:bool)
    n569 = Not Equal?(x=w1252, y=w1250) -> (x != y?=w1251:bool)
    n570 = case shown="真" w1362 {
      tunnel: w1360 -> [_ w1539]
      tunnel: w638 -> [_ w1538]
      tunnel: w637 -> [_ w1537]
      frame False {
      }
      frame True {
        n571 = call "xPCSetParam.vi"("value"=w1539, "index"=w1537, "port"=w1538) -> ()  [unwired: 1 in, 2 out]
      }
    }
    n572 = Build Array(w1296) -> (w1295:dbl[])
    n573 = Not Equal?(x=w1226, y=w1224) -> (x != y?=w1225:bool)
    n574 = Not Equal?(x=w1214, y=w1212) -> (x != y?=w1213:bool)
    n575 = case shown="真" w1107 {
      tunnel: w1109 -> [_ w1437]
      tunnel: w1105 -> [_ w1436]
      tunnel: w1104 -> [_ w1435]
      frame False {
      }
      frame True {
        n576 = call "xPCSetParam.vi"("value"=w1437, "index"=w1435, "port"=w1436) -> ()  [unwired: 1 in, 2 out]
      }
    }
    n577 = Build Array(w1284) -> (w1283:dbl[])
    n578 = Not Equal?(x=w1208, y=w1206) -> (x != y?=w1207:bool)
    n579 = Not Equal?(x=w1256, y=w1254) -> (x != y?=w1255:bool)
    n580 = Not Equal?(x=w1220, y=w1218) -> (x != y?=w1219:bool)
    n581 = case shown="真" w1112 {
      tunnel: w1114 -> [_ w1440]
      tunnel: w1111 -> [_ w1439]
      tunnel: w1110 -> [_ w1438]
      frame False {
      }
      frame True {
        n582 = call "xPCSetParam.vi"("value"=w1440, "index"=w1438, "port"=w1439) -> ()  [unwired: 1 in, 2 out]
      }
    }
    n583 = Index Array(array=w664, index=5 ("索引")) -> (element=w667:dbl)
    n584 = Index Array(array=w789, index=5 ("索引")) -> (element=w792:dbl)
    n585 = case shown="真" w1344 {
      tunnel: w1347 -> [_ w1530]
      tunnel: w1346 -> [_ w1529]
      tunnel: w1342 -> [_ w1528]
      frame False {
      }
      frame True {
        n586 = call "xPCSetParam.vi"("value"=w1528, "index"=w1529, "port"=w1530) -> ()  [unwired: 1 in, 2 out]
      }
    }
    n587 = Index Array(array=w874, index=5 ("索引")) -> (element=w877:dbl)
    n588 = Index Array(array=w849, index=5 ("索引")) -> (element=w852:dbl)
    n589 = Build Array(w1272) -> (w1271:dbl[])
    n590 = case shown="真" w1338 {
      tunnel: w1341 -> [_ w1527]
      tunnel: w1340 -> [_ w1526]
      tunnel: w1336 -> [_ w1525]
      frame False {
      }
      frame True {
        n591 = call "xPCSetParam.vi"("value"=w1525, "index"=w1526, "port"=w1527) -> ()  [unwired: 1 in, 2 out]
      }
    }
    n592 = case shown="真" w1103 {
      tunnel: w1102 -> [_ w1434]
      tunnel: w1101 -> [_ w1433]
      tunnel: w1100 -> [_ w1432]
      frame False {
      }
      frame True {
        n593 = call "xPCSetParam.vi"("value"=w1434, "index"=w1432, "port"=w1433) -> ()  [unwired: 1 in, 2 out]
      }
    }
    n594 = Build Array(w1280) -> (w1277:dbl[])
    n595 = Index Array(array=w814, index=5 ("索引")) -> (element=w817:dbl)
    n596 = Index Array(array=w949, index=5 ("索引")) -> (element=w952:dbl)
    n597 = Index Array(array=w976, index=5 ("索引")) -> (element=w979:dbl)
    n598 = case shown="真" w1334 {
      tunnel: w1333 -> [_ w1524]
      tunnel: w1331 -> [_ w1523]
      tunnel: w1330 -> [_ w1522]
      frame False {
      }
      frame True {
        n599 = call "xPCSetParam.vi"("value"=w1524, "index"=w1522, "port"=w1523) -> ()  [unwired: 1 in, 2 out]
      }
    }
    n600 = Build Array(w1193) -> (w1194:dbl[])
    n601 = Index Array(array=w689, index=5 ("索引")) -> (element=w692:dbl)
    n602 = Index Array(array=w1030, index=5 ("索引")) -> (element=w1033:dbl)
    n603 = Build Array(w1259) -> (w1260:dbl[])
    n604 = case shown="真" w1324 {
      tunnel: w1322 -> [_ w1518]
      tunnel: w649 -> [_ w1517]
      tunnel: w1321 -> [_ w1516]
      frame False {
      }
      frame True {
        n605 = call "xPCSetParam.vi"("value"=w1518, "index"=w1516, "port"=w1517) -> ()  [unwired: 1 in, 2 out]
      }
    }
    n606 = case shown="真" w1328 {
      tunnel: w1301 -> [_ w1521]
      tunnel: w1326 -> [_ w1520]
      tunnel: w1323 -> [_ w1519]
      frame False {
      }
      frame True {
        n607 = call "xPCSetParam.vi"("value"=w1519, "index"=w1520, "port"=w1521) -> ()  [unwired: 1 in, 2 out]
      }
    }
    n608 = Build Array(w1268) -> (w1265:dbl[])
    n609 = Index Array(array=w924, index=5 ("索引")) -> (element=w927:dbl)
    n610 = Index Array(array=w1057, index=5 ("索引")) -> (element=w1060:dbl)
    n611 = Index Array(array=w764, index=5 ("索引")) -> (element=w767:dbl)
    n612 = Index Array(array=w739, index=5 ("索引")) -> (element=w742:dbl)
    n613 = case shown="真" w1310 {
      tunnel: w1313 -> [_ w1512]
      tunnel: w1312 -> [_ w1511]
      tunnel: w1308 -> [_ w1510]
      frame False {
      }
      frame True {
        n614 = call "xPCSetParam.vi"("value"=w1510, "index"=w1511, "port"=w1512) -> ()  [unwired: 1 in, 2 out]
      }
    }
    n615 = case shown="真" w1306 {
      tunnel: w1304 -> [_ w1509]
      tunnel: w1303 -> [_ w1508]
      tunnel: w1302 -> [_ w1507]
      frame False {
      }
      frame True {
        n616 = call "xPCSetParam.vi"("value"=w1509, "index"=w1507, "port"=w1508) -> ()  [unwired: 1 in, 2 out]
      }
    }
    n617 = Index Array(array=w714, index=5 ("索引")) -> (element=w717:dbl)
    n618 = case shown="真" w1297 {
      tunnel: w1300 -> [_ w1506]
      tunnel: w1299 -> [_ w1505]
      tunnel: w1295 -> [_ w1504]
      frame False {
      }
      frame True {
        n619 = call "xPCSetParam.vi"("value"=w1504, "index"=w1505, "port"=w1506) -> ()  [unwired: 1 in, 2 out]
      }
    }
    n620 = case shown="真" w1318 {
      tunnel: w1317 -> [_ w1515]
      tunnel: w1316 -> [_ w1514]
      tunnel: w1314 -> [_ w1513]
      frame False {
      }
      frame True {
        n621 = call "xPCSetParam.vi"("value"=w1513, "index"=w1514, "port"=w1515) -> ()  [unwired: 1 in, 2 out]
      }
    }
    n622 = Index Array(array=w899, index=5 ("索引")) -> (element=w902:dbl)
    n623 = Index Array(array=w1082, index=0 ("索引")) -> (element=w1096:dbl)
    n624 = Index Array(array=w1003, index=5 ("索引")) -> (element=w1006:dbl)
    n625 = Build Array(w1250) -> (w1247:dbl[])
    n626 = Build Array(w1206) -> (w1205:dbl[])
    n627 = Equal?(x=w667, y=1.0) -> (x = y?=w665:bool)
    n628 = Equal?(x=w792, y=1.0) -> (x = y?=w790:bool)
    n629 = Equal?(x=w877, y=1.0) -> (x = y?=w875:bool)
    n630 = case shown="真" w1293 {
      tunnel: w1292 -> [_ w1503]
      tunnel: w1290 -> [_ w1502]
      tunnel: w1289 -> [_ w1501]
      frame False {
      }
      frame True {
        n631 = call "xPCSetParam.vi"("value"=w1503, "index"=w1501, "port"=w1502) -> ()  [unwired: 1 in, 2 out]
      }
    }
    n632 = Index Array(array=w1119, index=1 ("索引")) -> (element=w1128:dbl)
    n633 = Equal?(x=w852, y=1.0) -> (x = y?=w850:bool)
    n634 = Index Array(array=w1082, index=1 ("索引")) -> (element=w1092:dbl)
    n635 = Build Array(w1242) -> (w1241:dbl[])
    n636 = Build Array(w1200) -> (w1199:dbl[])
    n637 = Index Array(array=w1119, index=0 ("索引")) -> (element=w1130:dbl)
    n638 = Equal?(x=w817, y=1.0) -> (x = y?=w815:bool)
    n639 = Equal?(x=w952, y=1.0) -> (x = y?=w950:bool)
    n640 = Index Array(array=w1119, index=2 ("索引")) -> (element=w1126:dbl)
    n641 = Equal?(x=w979, y=1.0) -> (x = y?=w977:bool)
    n642 = Equal?(x=w692, y=1.0) -> (x = y?=w690:bool)
    n643 = Equal?(x=w1033, y=1.0) -> (x = y?=w1031:bool)
    n644 = case shown="真" w1285 {
      tunnel: w1288 -> [_ w1500]
      tunnel: w1287 -> [_ w1499]
      tunnel: w1283 -> [_ w1498]
      frame False {
      }
      frame True {
        n645 = call "xPCSetParam.vi"("value"=w1498, "index"=w1499, "port"=w1500) -> ()  [unwired: 1 in, 2 out]
      }
    }
    n646 = Index Array(array=w1135, index=2 ("索引")) -> (element=w1141:dbl)
    n647 = Equal?(x=w927, y=1.0) -> (x = y?=w925:bool)
    n648 = case shown="真" w1281 {
      tunnel: w1279 -> [_ w1497]
      tunnel: w1278 -> [_ w1496]
      tunnel: w1277 -> [_ w1495]
      frame False {
      }
      frame True {
        n649 = call "xPCSetParam.vi"("value"=w1495, "index"=w1496, "port"=w1497) -> ()  [unwired: 1 in, 2 out]
      }
    }
    n650 = Index Array(array=w1135, index=3 ("索引")) -> (element=w1138:dbl)
    n651 = Equal?(x=w1060, y=1.0) -> (x = y?=w1058:bool)
    n652 = Index Array(array=w1135, index=1 ("索引")) -> (element=w1145:dbl)
    n653 = Build Array(w1230) -> (w1229:dbl[])
    n654 = Index Array(array=w1135, index=0 ("索引")) -> (element=w1149:dbl)
    n655 = case shown="真" w1273 {
      tunnel: w1276 -> [_ w1494]
      tunnel: w1275 -> [_ w1493]
      tunnel: w1271 -> [_ w1492]
      frame False {
      }
      frame True {
        n656 = call "xPCSetParam.vi"("value"=w1492, "index"=w1493, "port"=w1494) -> ()  [unwired: 1 in, 2 out]
      }
    }
    n657 = Build Array(w1254) -> (w1253:dbl[])
    n658 = Build Array(w1224) -> (w1223:dbl[])
    n659 = Index Array(array=w1153, index=2 ("索引")) -> (element=w1181:dbl)
    n660 = Equal?(x=w767, y=1.0) -> (x = y?=w765:bool)
    n661 = Equal?(x=w742, y=1.0) -> (x = y?=w740:bool)
    n662 = Build Array(w1236) -> (w1235:dbl[])
    n663 = Index Array(array=w1153, index=3 ("索引")) -> (element=w1177:dbl)
    n664 = Index Array(array=w1153, index=1 ("索引")) -> (element=w1185:dbl)
    n665 = case shown="真" w1195 {
      tunnel: w1198 -> [_ w1455]
      tunnel: w1197 -> [_ w1454]
      tunnel: w1194 -> [_ w1453]
      frame False {
      }
      frame True {
        n666 = call "xPCSetParam.vi"("value"=w1453, "index"=w1454, "port"=w1455) -> ()  [unwired: 1 in, 2 out]
      }
    }
    n667 = Index Array(array=w1153, index=0 ("索引")) -> (element=w1189:dbl)
    n668 = Index Array(array=w1153, index=4 ("索引")) -> (element=w1173:dbl)
    n669 = Equal?(x=w717, y=1.0) -> (x = y?=w715:bool)
    n670 = case shown="真" w1269 {
      tunnel: w1267 -> [_ w1491]
      tunnel: w1266 -> [_ w1490]
      tunnel: w1265 -> [_ w1489]
      frame False {
      }
      frame True {
        n671 = call "xPCSetParam.vi"("value"=w1489, "index"=w1490, "port"=w1491) -> ()  [unwired: 1 in, 2 out]
      }
    }
    n672 = case shown="真" w1261 {
      tunnel: w1264 -> [_ w1488]
      tunnel: w1263 -> [_ w1487]
      tunnel: w1260 -> [_ w1486]
      frame False {
      }
      frame True {
        n673 = call "xPCSetParam.vi"("value"=w1486, "index"=w1487, "port"=w1488) -> ()  [unwired: 1 in, 2 out]
      }
    }
    n674 = Build Array(w1218) -> (w1217:dbl[])
    n675 = Equal?(x=w902, y=1.0) -> (x = y?=w900:bool)
    n676 = Build Array(w1212) -> (w1211:dbl[])
    n677 = Equal?(x=w1006, y=1.0) -> (x = y?=w1004:bool)
    n678 = global write "全局变量.vi" "sd压紧异常"(w665) -> ()
    n679 = global write "全局变量.vi" "zd压紧异常"(w875) -> ()
    n680 = global write "全局变量.vi" "sd压紧异常"(w790) -> ()
    n681 = Equal?(x=w1096, y=1.0) -> (x = y?=w1095:bool)
    n682 = global write "全局变量.vi" "sd压紧异常"(w850) -> ()
    n683 = global write "全局变量.vi" "songkaitm"(w1130) -> ()
    n684 = global write "全局变量.vi" "kaigaitm"(w1128) -> ()
    n685 = global write "全局变量.vi" "zd压紧异常"(w950) -> ()
    n686 = global write "全局变量.vi" "sd压紧异常"(w815) -> ()
    n687 = global write "全局变量.vi" "suodingtm"(w1126) -> ()
    n688 = case shown="真" w1207 {
      tunnel: w1210 -> [_ w1461]
      tunnel: w1209 -> [_ w1460]
      tunnel: w1205 -> [_ w1459]
      frame False {
      }
      frame True {
        n689 = call "xPCSetParam.vi"("value"=w1459, "index"=w1460, "port"=w1461) -> ()  [unwired: 1 in, 2 out]
      }
    }
    n690 = global write "全局变量.vi" "zd压紧异常"(w977) -> ()
    n691 = global write "全局变量.vi" "sd压紧异常"(w690) -> ()
    n692 = global write "全局变量.vi" "zd压紧异常"(w1031) -> ()
    n693 = case shown="真" w1201 {
      tunnel: w1204 -> [_ w1458]
      tunnel: w1203 -> [_ w1457]
      tunnel: w1199 -> [_ w1456]
      frame False {
      }
      frame True {
        n694 = call "xPCSetParam.vi"("value"=w1456, "index"=w1457, "port"=w1458) -> ()  [unwired: 1 in, 2 out]
      }
    }
    n695 = Equal?(x=w1092, y=1.0) -> (x = y?=w1091:bool)
    n696 = global write "全局变量.vi" "zd压紧异常"(w925) -> ()
    n697 = global write "全局变量.vi" "zd压紧异常"(w1058) -> ()
    n698 = case shown="真" w1255 {
      tunnel: w1258 -> [_ w1485]
      tunnel: w1257 -> [_ w1484]
      tunnel: w1253 -> [_ w1483]
      frame False {
      }
      frame True {
        n699 = call "xPCSetParam.vi"("value"=w1483, "index"=w1484, "port"=w1485) -> ()  [unwired: 1 in, 2 out]
      }
    }
    n700 = Equal?(x=w1141, y=1.0) -> (x = y?=w1139:bool)
    n701 = global write "全局变量.vi" "sd压紧异常"(w765) -> ()
    n702 = Equal?(x=w1138, y=1.0) -> (x = y?=w1136:bool)
    n703 = global write "全局变量.vi" "sd压紧异常"(w740) -> ()
    n704 = Equal?(x=w1145, y=1.0) -> (x = y?=w1143:bool)
    n705 = Equal?(x=w1149, y=1.0) -> (x = y?=w1147:bool)
    n706 = case shown="真" w1251 {
      tunnel: w1249 -> [_ w1482]
      tunnel: w1248 -> [_ w1481]
      tunnel: w1247 -> [_ w1480]
      frame False {
      }
      frame True {
        n707 = call "xPCSetParam.vi"("value"=w1480, "index"=w1481, "port"=w1482) -> ()  [unwired: 1 in, 2 out]
      }
    }
    n708 = Equal?(x=w1181, y=1.0) -> (x = y?=w1179:bool)
    n709 = case shown="真" w1237 {
      tunnel: w1240 -> [_ w1476]
      tunnel: w1239 -> [_ w1475]
      tunnel: w1235 -> [_ w1474]
      frame False {
      }
      frame True {
        n710 = call "xPCSetParam.vi"("value"=w1474, "index"=w1475, "port"=w1476) -> ()  [unwired: 1 in, 2 out]
      }
    }
    n711 = Equal?(x=w1177, y=1.0) -> (x = y?=w1175:bool)
    n712 = global write "全局变量.vi" "sd压紧异常"(w715) -> ()
    n713 = case shown="真" w1243 {
      tunnel: w1246 -> [_ w1479]
      tunnel: w1245 -> [_ w1478]
      tunnel: w1241 -> [_ w1477]
      frame False {
      }
      frame True {
        n714 = call "xPCSetParam.vi"("value"=w1477, "index"=w1478, "port"=w1479) -> ()  [unwired: 1 in, 2 out]
      }
    }
    n715 = Equal?(x=w1185, y=1.0) -> (x = y?=w1183:bool)
    n716 = Equal?(x=w1189, y=1.0) -> (x = y?=w1187:bool)
    n717 = global write "全局变量.vi" "zd压紧异常"(w900) -> ()
    n718 = Equal?(x=w1173, y=1.0) -> (x = y?=w1171:bool)
    n719 = global write "全局变量.vi" "zd压紧异常"(w1004) -> ()
    n720 = case shown="真" w1231 {
      tunnel: w1234 -> [_ w1473]
      tunnel: w1233 -> [_ w1472]
      tunnel: w1229 -> [_ w1471]
      frame False {
      }
      frame True {
        n721 = call "xPCSetParam.vi"("value"=w1471, "index"=w1472, "port"=w1473) -> ()  [unwired: 1 in, 2 out]
      }
    }
    n722 = case shown="真" w1225 {
      tunnel: w1228 -> [_ w1470]
      tunnel: w1227 -> [_ w1469]
      tunnel: w1223 -> [_ w1468]
      frame False {
      }
      frame True {
        n723 = call "xPCSetParam.vi"("value"=w1468, "index"=w1469, "port"=w1470) -> ()  [unwired: 1 in, 2 out]
      }
    }
    n724 = case shown="真" w1213 {
      tunnel: w1216 -> [_ w1464]
      tunnel: w1215 -> [_ w1463]
      tunnel: w1211 -> [_ w1462]
      frame False {
      }
      frame True {
        n725 = call "xPCSetParam.vi"("value"=w1462, "index"=w1463, "port"=w1464) -> ()  [unwired: 1 in, 2 out]
      }
    }
    n726 = case shown="真" w1219 {
      tunnel: w1222 -> [_ w1467]
      tunnel: w1221 -> [_ w1466]
      tunnel: w1217 -> [_ w1465]
      frame False {
      }
      frame True {
        n727 = call "xPCSetParam.vi"("value"=w1465, "index"=w1466, "port"=w1467) -> ()  [unwired: 1 in, 2 out]
      }
    }
    n728 = global write "全局变量.vi" "松开换向阀"(w1095) -> ()
    n729 = global write "全局变量.vi" "开盖换向阀"(w1091) -> ()
    n730 = global write "全局变量.vi" "关盖指令1"(w1139) -> ()
    n731 = global write "全局变量.vi" "关盖指令2"(w1136) -> ()
    n732 = global write "全局变量.vi" "开盖指令2"(w1143) -> ()
    n733 = global write "全局变量.vi" "开盖指令1"(w1147) -> ()
    n734 = global write "全局变量.vi" "关盖到位1"(w1179) -> ()
    n735 = global write "全局变量.vi" "开盖到位2"(w1183) -> ()
    n736 = global write "全局变量.vi" "关盖到位2"(w1175) -> ()
    n737 = global write "全局变量.vi" "开盖到位1"(w1187) -> ()
    n738 = global write "全局变量.vi" "开盖缓冲"(w1171) -> ()
    n739 = global read "全局变量.vi" "jieshu"() -> (w647:dbl)
    n740 = Index Array(array=w1119, index=4 ("索引")) -> (element=w1122:dbl)
    n741 = Index Array(array=w1119, index=5 ("索引")) -> (element=w1120:dbl)
    n742 = Index Array(array=w1119, index=3 ("索引")) -> (element=w1124:dbl)
    n743 = Index Array(array=w1082, index=3 ("索引")) -> (element=w1084:dbl)
    n744 = Index Array(array=w1082, index=2 ("索引")) -> (element=w1088:dbl)
    n745 = Index Array(array=w1153, index=5 ("索引")) -> (element=w1169:dbl)
    n746 = global write "全局变量.vi" "guangaitm"(w1122) -> ()
    n747 = Index Array(array=w1153, index=6 ("索引")) -> (element=w1165:dbl)
    n748 = Index Array(array=w1153, index=7 ("索引")) -> (element=w1161:dbl)
    n749 = global write "全局变量.vi" "jiesuotm"(w1124) -> ()
    n750 = global write "全局变量.vi" "yajintm"(w1120) -> ()
    n751 = Index Array(array=w1153, index=8 ("索引")) -> (element=w1158:dbl)
    n752 = Index Array(array=w1153, index=9 ("索引")) -> (element=w1155:dbl)
    n753 = Equal?(x=w1084, y=1.0) -> (x = y?=w1083:bool)
    n754 = Not Equal To 0?(x=w647) -> (x != 0?=w646:bool)
    n755 = Equal?(x=w1088, y=1.0) -> (x = y?=w1087:bool)
    n756 = Equal?(x=w1169, y=1.0) -> (x = y?=w1167:bool)
    n757 = Equal?(x=w1165, y=1.0) -> (x = y?=w1163:bool)
    n758 = Equal?(x=w1161, y=1.0) -> (x = y?=w635:bool)
    n759 = Equal?(x=w1158, y=1.0) -> (x = y?=w636:bool)
    n760 = Equal?(x=w1155, y=1.0) -> (x = y?=w634:bool)
    n761 = global write "全局变量.vi" "关盖换向阀"(w1083) -> ()
    n762 = global write "全局变量.vi" "压紧换向阀"(w1087) -> ()
    n763 = global write "全局变量.vi" "关盖缓冲"(w1167) -> ()
    n764 = global write "全局变量.vi" "解锁到位"(w635) -> ()
    n765 = global write "全局变量.vi" "锁定到位"(w1163) -> ()
    n766 = global write "全局变量.vi" "松开到位"(w634) -> ()
    n767 = global write "全局变量.vi" "压紧到位"(w636) -> ()
  }
  n768 = stacked-sequence {
    tunnel: w94 -> [w1549]
    frame #0 {
      n769 = call "xPCStopApp.vi"("port"=w1549) -> ("port copy"=w1550:i32)  [unwired: 1 in, 1 out]
      n770 = call "xPCClosePort.vi"("port"=w1550) -> ()  [unwired: 1 in, 2 out]
    }
  }
  n771 = flat-sequence {
    frame #0 {
      n772 = global write "全局变量.vi" "s8"(0.0 ("s1")) -> ()
      n773 = global write "全局变量.vi" "sds3"(0.0 ("s1")) -> ()
      n774 = global write "全局变量.vi" "s4"(0.0 ("s1")) -> ()
      n775 = global write "全局变量.vi" "s7"(0.0 ("s1")) -> ()
      n776 = global write "全局变量.vi" "sds2"(0.0 ("s1")) -> ()
      n777 = global write "全局变量.vi" "s6"(0.0 ("s1")) -> ()
      n778 = global write "全局变量.vi" "sds1"(0.0 ("s1")) -> ()
      n779 = global write "全局变量.vi" "suodingtm"(0.0 ("s1")) -> ()
      n780 = global write "全局变量.vi" "s5"(0.0 ("s1")) -> ()
      n781 = global write "全局变量.vi" "guangaitm"(0.0 ("s1")) -> ()
      n782 = global write "全局变量.vi" "jiesuotm"(0.0 ("s1")) -> ()
      n783 = global write "全局变量.vi" "kaigaitm"(0.0 ("s1")) -> ()
      n784 = global write "全局变量.vi" "yajintm"(0.0 ("s1")) -> ()
      n785 = global write "全局变量.vi" "songkaitm"(0.0 ("s1")) -> ()
      n786 = global write "全局变量.vi" "guan2"(0.0 ("s1")) -> ()
      n787 = global write "全局变量.vi" "ya2"(0.0 ("s1")) -> ()
      n788 = global write "全局变量.vi" "kai2"(0.0 ("s1")) -> ()
      n789 = global write "全局变量.vi" "guan1"(0.0 ("s1")) -> ()
      n790 = global write "全局变量.vi" "song1"(0.0 ("s1")) -> ()
      n791 = global write "全局变量.vi" "time1"(0.0 ("s1")) -> ()
      n792 = global write "全局变量.vi" "kai1"(0.0 ("s1")) -> ()
      n793 = global write "全局变量.vi" "ya1"(0.0 ("s1")) -> ()
      n794 = global write "全局变量.vi" "zds8"(0.0 ("s1")) -> ()
      n795 = global write "全局变量.vi" "sds6"(0.0 ("s1")) -> ()
      n796 = global write "全局变量.vi" "zds7"(0.0 ("s1")) -> ()
      n797 = global write "全局变量.vi" "zds4"(0.0 ("s1")) -> ()
      n798 = global write "全局变量.vi" "sds5"(0.0 ("s1")) -> ()
      n799 = global write "全局变量.vi" "t6"(0.0 ("s1")) -> ()
      n800 = global write "全局变量.vi" "t5"(0.0 ("s1")) -> ()
      n801 = global write "全局变量.vi" "t4"(0.0 ("s1")) -> ()
      n802 = global write "全局变量.vi" "t3"(0.0 ("s1")) -> ()
      n803 = global write "全局变量.vi" "zds3"(0.0 ("s1")) -> ()
      n804 = global write "全局变量.vi" "zds2"(0.0 ("s1")) -> ()
      n805 = global write "全局变量.vi" "t2"(0.0 ("s1")) -> ()
      n806 = global write "全局变量.vi" "t1"(0.0 ("s1")) -> ()
      n807 = global write "全局变量.vi" "zds1"(0.0 ("s1")) -> ()
      n808 = global write "全局变量.vi" "guan5"(0.0 ("s1")) -> ()
      n809 = global write "全局变量.vi" "song4"(0.0 ("s1")) -> ()
      n810 = global write "全局变量.vi" "guan4"(0.0 ("s1")) -> ()
      n811 = global write "全局变量.vi" "kai4"(0.0 ("s1")) -> ()
      n812 = global write "全局变量.vi" "ya4"(0.0 ("s1")) -> ()
      n813 = global write "全局变量.vi" "ya5"(0.0 ("s1")) -> ()
      n814 = global write "全局变量.vi" "已开盖次数"(0.0 ("Switch1")) -> ()
      n815 = global write "全局变量.vi" "guan3"(0.0 ("s1")) -> ()
      n816 = global write "全局变量.vi" "song3"(0.0 ("s1")) -> ()
      n817 = global write "全局变量.vi" "song2"(0.0 ("s1")) -> ()
      n818 = global write "全局变量.vi" "kai3"(0.0 ("s1")) -> ()
      n819 = global write "全局变量.vi" "ya3"(0.0 ("s1")) -> ()
      n820 = global write "全局变量.vi" "tskaishi1"(0.0 ("s1")) -> ()
      n821 = global write "全局变量.vi" "tskaishi4"(0.0 ("s1")) -> ()
      n822 = global write "全局变量.vi" "tskaishi3"(0.0 ("s1")) -> ()
      n823 = global write "全局变量.vi" "tskaishi2"(0.0 ("s1")) -> ()
      n824 = global write "全局变量.vi" "tiaoshimoshi"(0.0 ("s1")) -> ()
      n825 = global write "全局变量.vi" "start"(0.0 ("s1")) -> ()
      n826 = global write "全局变量.vi" "guan7"(0.0 ("s1")) -> ()
      n827 = global write "全局变量.vi" "ya7"(0.0 ("s1")) -> ()
      n828 = global write "全局变量.vi" "song7"(0.0 ("s1")) -> ()
      n829 = global write "全局变量.vi" "kai7"(0.0 ("s1")) -> ()
      n830 = global write "全局变量.vi" "zidong"(0.0 ("s1")) -> ()
      n831 = global write "全局变量.vi" "tskaishi8"(0.0 ("s1")) -> ()
      n832 = global write "全局变量.vi" "tskaishi7"(0.0 ("s1")) -> ()
      n833 = global write "全局变量.vi" "tskaishi6"(0.0 ("s1")) -> ()
      n834 = global write "全局变量.vi" "Switch1"(0.0 ("s1")) -> ()
      n835 = global write "全局变量.vi" "tskaishi5"(0.0 ("s1")) -> ()
      n836 = global write "全局变量.vi" "Switch2"(0.0 ("s1")) -> ()
      n837 = global write "全局变量.vi" "Switch"(0.0 ("s1")) -> ()
      n838 = global write "全局变量.vi" "kaigaicishu"(0.0 ("s1")) -> ()
      n839 = global write "全局变量.vi" "kaishi1"(0.0 ("s1")) -> ()
      n840 = global write "全局变量.vi" "kaishi4"(0.0 ("s1")) -> ()
      n841 = global write "全局变量.vi" "jieshu"(0.0 ("s1")) -> ()
      n842 = global write "全局变量.vi" "jiesuo"(0.0 ("s1")) -> ()
      n843 = global write "全局变量.vi" "qidongsd"(0.0 ("s1")) -> ()
      n844 = global write "全局变量.vi" "qidongzd"(0.0 ("s1")) -> ()
      n845 = global write "全局变量.vi" "kaishi5"(0.0 ("s1")) -> ()
      n846 = global write "全局变量.vi" "kaishi8"(0.0 ("s1")) -> ()
      n847 = global write "全局变量.vi" "kaishi6"(0.0 ("s1")) -> ()
      n848 = global write "全局变量.vi" "kaishi3"(0.0 ("s1")) -> ()
      n849 = global write "全局变量.vi" "kaishi7"(0.0 ("s1")) -> ()
      n850 = global write "全局变量.vi" "songkai"(0.0 ("s1")) -> ()
      n851 = global write "全局变量.vi" "kaishi2"(0.0 ("s1")) -> ()
      n852 = global write "全局变量.vi" "tssongkai"(0.0 ("s1")) -> ()
      n853 = global write "全局变量.vi" "tsguangai"(0.0 ("s1")) -> ()
      n854 = global write "全局变量.vi" "tskaigai"(0.0 ("s1")) -> ()
      n855 = global write "全局变量.vi" "tsjiesuo"(0.0 ("s1")) -> ()
      n856 = property on="开盖次数设置" class="DigNum (严格)"("Value"=0.0 ("开盖次数")) -> ()  [unwired: 2 in, 2 out]
      n857 = global write "全局变量.vi" "关盖到位1"(FALSE ("解锁到位")) -> ()
      n858 = global write "全局变量.vi" "suoding"(0.0 ("s1")) -> ()
      n859 = global write "全局变量.vi" "开盖缓冲"(FALSE ("解锁到位")) -> ()
      n860 = global write "全局变量.vi" "关盖到位2"(FALSE ("解锁到位")) -> ()
      n861 = global write "全局变量.vi" "开盖到位2"(FALSE ("解锁到位")) -> ()
      n862 = global write "全局变量.vi" "kaigai"(0.0 ("s1")) -> ()
      n863 = global write "全局变量.vi" "开盖到位1"(FALSE ("解锁到位")) -> ()
      n864 = global write "全局变量.vi" "松开到位"(FALSE ("解锁到位")) -> ()
      n865 = global write "全局变量.vi" "压紧到位"(FALSE ("解锁到位")) -> ()
      n866 = global write "全局变量.vi" "yajin"(0.0 ("s1")) -> ()
      n867 = global write "全局变量.vi" "解锁到位"(FALSE ("解锁到位")) -> ()
      n868 = global write "全局变量.vi" "关盖缓冲"(FALSE ("解锁到位")) -> ()
      n869 = global write "全局变量.vi" "锁定到位"(FALSE ("解锁到位")) -> ()
      n870 = global write "全局变量.vi" "tssuoding"(0.0 ("s1")) -> ()
      n871 = global write "全局变量.vi" "guangai"(0.0 ("s1")) -> ()
      n872 = global write "全局变量.vi" "tsyajin"(0.0 ("s1")) -> ()
    }
  }
  n873 = while {
    stop <- FALSE stop-if-true
    n874 = global read "全局变量.vi" "zd松开异常"() -> (w1671:bool)
    n875 = global read "全局变量.vi" "zd锁定异常"() -> (w1662:bool)
    n876 = global read "全局变量.vi" "sd锁定异常"() -> (w1663:bool)
    n877 = global read "全局变量.vi" "sd松开异常"() -> (w1672:bool)
    n878 = global read "全局变量.vi" "开盖缓冲异常"() -> (w1653:bool)
    n879 = Or(x=w1663, y=w1662) -> (x .or. y?=w1661:bool)
    n880 = Or(x=w1672, y=w1671) -> (x .or. y?=w1670:bool)
    n881 = case shown="真" w1670 {
      frame False {
      }
      frame True {
        "松开异常" <- TRUE ("松开异常")
        "字符串 2" <- "松开换向异常"
      }
    }
    n882 = case shown="真" w1661 {
      frame False {
      }
      frame True {
        "锁定异常" <- TRUE ("锁定异常")
        "字符串 5" <- "锁定换向异常"
      }
    }
    n883 = case shown="真" w1653 {
      frame False {
      }
      frame True {
        "开盖缓冲异常" <- TRUE ("锁定异常")
        "字符串 8" <- "开盖缓冲异常"
      }
    }
    n884 = global read "全局变量.vi" "sd开盖异常"() -> (w1668:bool)
    n885 = global read "全局变量.vi" "zd开盖异常"() -> (w1667:bool)
    n886 = global read "全局变量.vi" "zd压紧异常"() -> (w1659:bool)
    n887 = global read "全局变量.vi" "sd压紧异常"() -> (w1658:bool)
    n888 = global read "全局变量.vi" "关盖缓冲异常"() -> (w1652:bool)
    n889 = Or(x=w1668, y=w1667) -> (x .or. y?=w1669:bool)
    n890 = Or(x=w1658, y=w1659) -> (x .or. y?=w1660:bool)
    n891 = case shown="真" w1669 {
      frame False {
      }
      frame True {
        "开盖异常" <- TRUE ("开盖异常")
        "字符串 3" <- "开盖换向异常"
      }
    }
    n892 = case shown="真" w1660 {
      frame False {
      }
      frame True {
        "压紧异常" <- TRUE ("压紧异常")
        "字符串 6" <- "压紧换向异常"
      }
    }
    n893 = case shown="真" w1652 {
      frame False {
      }
      frame True {
        "关盖缓冲异常" <- TRUE ("锁定异常")
        "字符串 9" <- "关盖缓冲异常"
      }
    }
    n894 = global read "全局变量.vi" "zd关盖异常"() -> (w1665:bool)
    n895 = global read "全局变量.vi" "sd解锁异常"() -> (w1656:bool)
    n896 = global read "全局变量.vi" "sd关盖异常"() -> (w1664:bool)
    n897 = global read "全局变量.vi" "zd解锁异常"() -> (w1655:bool)
    n898 = Or(x=w1664, y=w1665) -> (x .or. y?=w1666:bool)
    n899 = Or(x=w1656, y=w1655) -> (x .or. y?=w1657:bool)
    n900 = case shown="真" w1657 {
      frame False {
      }
      frame True {
        "解锁异常" <- TRUE ("解锁异常")
        "字符串 7" <- "解锁换向异常"
      }
    }
    n901 = case shown="真" w1666 {
      frame False {
      }
      frame True {
        "关盖异常" <- TRUE ("关盖异常")
        "字符串 4" <- "关盖换向异常"
      }
    }
  }
  n902 = flat-sequence {
    frame #0 {
      n903 = property on="松开异常" class="Bool (严格)"("Value"=FALSE ("松开异常")) -> ()  [unwired: 2 in, 2 out]
      n904 = property on="锁定异常" class="Bool (严格)"("Value"=FALSE ("锁定异常")) -> ()  [unwired: 2 in, 2 out]
      n905 = property on="开盖异常" class="Bool (严格)"("Value"=FALSE ("开盖异常")) -> ()  [unwired: 2 in, 2 out]
      n906 = property on="压紧异常" class="Bool (严格)"("Value"=FALSE ("压紧异常")) -> ()  [unwired: 2 in, 2 out]
      n907 = property on="关盖异常" class="Bool (严格)"("Value"=FALSE ("关盖异常")) -> ()  [unwired: 2 in, 2 out]
      n908 = property on="解锁异常" class="Bool (严格)"("Value"=FALSE ("解锁异常")) -> ()  [unwired: 2 in, 2 out]
      n909 = property on="字符串 8" class="Str"("Value"="" ("字符串 8")) -> ()  [unwired: 2 in, 2 out]
      n910 = property on="字符串 2" class="Str"("Value"="" ("字符串 2")) -> ()  [unwired: 2 in, 2 out]
      n911 = property on="字符串 9" class="Str"("Value"="" ("字符串 9")) -> ()  [unwired: 2 in, 2 out]
      n912 = property on="字符串 3" class="Str"("Value"="" ("字符串 3")) -> ()  [unwired: 2 in, 2 out]
      n913 = property on="字符串 4" class="Str"("Value"="" ("字符串 4")) -> ()  [unwired: 2 in, 2 out]
      n914 = property on="字符串 5" class="Str"("Value"="" ("字符串 5")) -> ()  [unwired: 2 in, 2 out]
      n915 = property on="字符串 6" class="Str"("Value"="" ("字符串 6")) -> ()  [unwired: 2 in, 2 out]
      n916 = property on="字符串 7" class="Str"("Value"="" ("字符串 7")) -> ()  [unwired: 2 in, 2 out]
    }
  }
  n917 = while {
    stop <- FALSE stop-if-true
    n918 = event shown="[11] \"退出系统\": 值改变" {
      selector: _ -> [_ _ _ _ _ _ _ _ _ _ _ _]
      dyn-events: _ -> [_ _ _ _ _ _ _ _ _ _ _ _]
      timeout: 10 -> [_ _ _ _ _ _ _ _ _ _ _ _]
      event Timeout {
        n919 = event-data() -> ()  [unwired: 1 in, 3 out]
      }
      event "井盖1": Value Change {
        n920 = event-data() -> ("NewVal"=w1707:bool)  [unwired: 1 in, 5 out]
        n921 = case shown="真" w1707 {
          frame False {
          }
          frame True {
            n922 = global write "全局变量.vi" "Switch1"(1.0 ("Switch1")) -> ()
            n923 = global write "全局变量.vi" "Switch2"(1.0 ("Switch2")) -> ()
            n924 = global write "全局变量.vi" "Switch"(1.0 ("Switch")) -> ()
          }
        }
        n925 = property on="自动操作" class="Bool (严格)"() -> ("Value"=w1706:bool)  [unwired: 2 in, 2 out]
        n926 = And(x=w1707, y=w1706) -> (x .and. y?=w1705:bool)
        n927 = case shown="真" w1705 {
          frame False {
          }
          frame True {
            n928 = global write "全局变量.vi" "sds4"(0.0 ("Switch")) -> ()
            n929 = global write "全局变量.vi" "zds3"(0.0 ("Switch")) -> ()
            n930 = global write "全局变量.vi" "zds2"(0.0 ("Switch")) -> ()
            n931 = global write "全局变量.vi" "zds1"(1.0 ("Switch")) -> ()
            n932 = global write "全局变量.vi" "zds8"(0.0 ("Switch")) -> ()
            n933 = global write "全局变量.vi" "sds6"(0.0 ("Switch")) -> ()
            n934 = global write "全局变量.vi" "zds7"(0.0 ("Switch")) -> ()
            n935 = global write "全局变量.vi" "sds5"(0.0 ("Switch")) -> ()
          }
        }
        n936 = property on="手动操作" class="Bool (严格)"() -> ("Value"=w1709:bool)  [unwired: 2 in, 2 out]
        n937 = And(x=w1707, y=w1709) -> (x .and. y?=w1708:bool)
        n938 = case shown="真" w1708 {
          frame False {
          }
          frame True {
            n939 = global write "全局变量.vi" "sds4"(0.0 ("Switch")) -> ()
            n940 = global write "全局变量.vi" "sds3"(0.0 ("Switch")) -> ()
            n941 = global write "全局变量.vi" "sds2"(0.0 ("Switch")) -> ()
            n942 = global write "全局变量.vi" "sds1"(1.0 ("Switch")) -> ()
            n943 = global write "全局变量.vi" "sds8"(0.0 ("Switch")) -> ()
            n944 = global write "全局变量.vi" "sds6"(0.0 ("Switch")) -> ()
            n945 = global write "全局变量.vi" "sds7"(0.0 ("Switch")) -> ()
            n946 = global write "全局变量.vi" "sds5"(0.0 ("Switch")) -> ()
          }
        }
      }
      event "井盖 2": Value Change {
        n947 = event-data() -> ("NewVal"=w1731:bool)  [unwired: 1 in, 5 out]
        n948 = case shown="真" w1731 {
          frame False {
          }
          frame True {
            n949 = global write "全局变量.vi" "Switch1"(2.0 ("Switch1")) -> ()
            n950 = global write "全局变量.vi" "Switch2"(2.0 ("Switch2")) -> ()
            n951 = global write "全局变量.vi" "Switch"(2.0 ("Switch")) -> ()
          }
        }
        n952 = property on="自动操作" class="Bool (严格)"() -> ("Value"=w1729:bool)  [unwired: 2 in, 2 out]
        n953 = property on="手动操作" class="Bool (严格)"() -> ("Value"=w1732:bool)  [unwired: 2 in, 2 out]
        n954 = And(x=w1731, y=w1729) -> (x .and. y?=w1730:bool)
        n955 = And(x=w1732, y=w1731) -> (x .and. y?=w1733:bool)
        n956 = case shown="真" w1730 {
          frame False {
          }
          frame True {
            n957 = global write "全局变量.vi" "sds4"(0.0 ("Switch")) -> ()
            n958 = global write "全局变量.vi" "zds3"(0.0 ("Switch")) -> ()
            n959 = global write "全局变量.vi" "zds2"(1.0 ("Switch")) -> ()
            n960 = global write "全局变量.vi" "zds1"(0.0 ("Switch")) -> ()
            n961 = global write "全局变量.vi" "zds8"(0.0 ("Switch")) -> ()
            n962 = global write "全局变量.vi" "sds6"(0.0 ("Switch")) -> ()
            n963 = global write "全局变量.vi" "zds7"(0.0 ("Switch")) -> ()
            n964 = global write "全局变量.vi" "sds5"(0.0 ("Switch")) -> ()
          }
        }
        n965 = case shown="真" w1733 {
          frame False {
          }
          frame True {
            n966 = global write "全局变量.vi" "sds4"(0.0 ("Switch")) -> ()
            n967 = global write "全局变量.vi" "sds3"(0.0 ("Switch")) -> ()
            n968 = global write "全局变量.vi" "sds2"(1.0 ("Switch")) -> ()
            n969 = global write "全局变量.vi" "sds1"(0.0 ("Switch")) -> ()
            n970 = global write "全局变量.vi" "sds8"(0.0 ("Switch")) -> ()
            n971 = global write "全局变量.vi" "sds6"(0.0 ("Switch")) -> ()
            n972 = global write "全局变量.vi" "sds7"(0.0 ("Switch")) -> ()
            n973 = global write "全局变量.vi" "sds5"(0.0 ("Switch")) -> ()
          }
        }
      }
      event "井盖 3": Value Change {
        n974 = event-data() -> ("NewVal"=w1753:bool)  [unwired: 1 in, 5 out]
        n975 = case shown="真" w1753 {
          frame False {
          }
          frame True {
            n976 = global write "全局变量.vi" "Switch1"(3.0 ("Switch1")) -> ()
            n977 = global write "全局变量.vi" "Switch2"(3.0 ("Switch2")) -> ()
            n978 = global write "全局变量.vi" "Switch"(3.0 ("Switch")) -> ()
          }
        }
        n979 = property on="自动操作" class="Bool (严格)"() -> ("Value"=w1755:bool)  [unwired: 2 in, 2 out]
        n980 = And(x=w1753, y=w1755) -> (x .and. y?=w1754:bool)
        n981 = property on="手动操作" class="Bool (严格)"() -> ("Value"=w1757:bool)  [unwired: 2 in, 2 out]
        n982 = And(x=w1757, y=w1753) -> (x .and. y?=w1756:bool)
        n983 = case shown="真" w1754 {
          frame False {
          }
          frame True {
            n984 = global write "全局变量.vi" "sds4"(0.0 ("Switch")) -> ()
            n985 = global write "全局变量.vi" "zds3"(1.0 ("Switch")) -> ()
            n986 = global write "全局变量.vi" "zds2"(0.0 ("Switch")) -> ()
            n987 = global write "全局变量.vi" "zds1"(0.0 ("Switch")) -> ()
            n988 = global write "全局变量.vi" "zds8"(0.0 ("Switch")) -> ()
            n989 = global write "全局变量.vi" "sds6"(0.0 ("Switch")) -> ()
            n990 = global write "全局变量.vi" "zds7"(0.0 ("Switch")) -> ()
            n991 = global write "全局变量.vi" "sds5"(0.0 ("Switch")) -> ()
          }
        }
        n992 = case shown="真" w1756 {
          frame False {
          }
          frame True {
            n993 = global write "全局变量.vi" "sds4"(0.0 ("Switch")) -> ()
            n994 = global write "全局变量.vi" "sds3"(1.0 ("Switch")) -> ()
            n995 = global write "全局变量.vi" "sds2"(0.0 ("Switch")) -> ()
            n996 = global write "全局变量.vi" "sds1"(0.0 ("Switch")) -> ()
            n997 = global write "全局变量.vi" "sds8"(0.0 ("Switch")) -> ()
            n998 = global write "全局变量.vi" "sds6"(0.0 ("Switch")) -> ()
            n999 = global write "全局变量.vi" "sds7"(0.0 ("Switch")) -> ()
            n1000 = global write "全局变量.vi" "sds5"(0.0 ("Switch")) -> ()
          }
        }
      }
      event "井盖 4": Value Change {
        n1001 = event-data() -> ("NewVal"=w1778:bool)  [unwired: 1 in, 5 out]
        n1002 = case shown="真" w1778 {
          frame False {
          }
          frame True {
            n1003 = global write "全局变量.vi" "Switch1"(4.0 ("Switch1")) -> ()
            n1004 = global write "全局变量.vi" "Switch2"(4.0 ("Switch2")) -> ()
            n1005 = global write "全局变量.vi" "Switch"(4.0 ("Switch")) -> ()
          }
        }
        n1006 = property on="自动操作" class="Bool (严格)"() -> ("Value"=w1779:bool)  [unwired: 2 in, 2 out]
        n1007 = property on="手动操作" class="Bool (严格)"() -> ("Value"=w1781:bool)  [unwired: 2 in, 2 out]
        n1008 = And(x=w1781, y=w1778) -> (x .and. y?=w1780:bool)
        n1009 = And(x=w1778, y=w1779) -> (x .and. y?=w1777:bool)
        n1010 = case shown="真" w1780 {
          frame False {
          }
          frame True {
            n1011 = global write "全局变量.vi" "sds4"(1.0 ("Switch")) -> ()
            n1012 = global write "全局变量.vi" "sds3"(0.0 ("Switch")) -> ()
            n1013 = global write "全局变量.vi" "sds2"(0.0 ("Switch")) -> ()
            n1014 = global write "全局变量.vi" "sds1"(0.0 ("Switch")) -> ()
            n1015 = global write "全局变量.vi" "sds8"(0.0 ("Switch")) -> ()
            n1016 = global write "全局变量.vi" "sds6"(0.0 ("Switch")) -> ()
            n1017 = global write "全局变量.vi" "sds7"(0.0 ("Switch")) -> ()
            n1018 = global write "全局变量.vi" "sds5"(0.0 ("Switch")) -> ()
          }
        }
        n1019 = case shown="真" w1777 {
          frame False {
          }
          frame True {
            n1020 = global write "全局变量.vi" "sds4"(1.0 ("Switch")) -> ()
            n1021 = global write "全局变量.vi" "zds3"(0.0 ("Switch")) -> ()
            n1022 = global write "全局变量.vi" "zds2"(0.0 ("Switch")) -> ()
            n1023 = global write "全局变量.vi" "zds1"(0.0 ("Switch")) -> ()
            n1024 = global write "全局变量.vi" "zds8"(0.0 ("Switch")) -> ()
            n1025 = global write "全局变量.vi" "sds6"(0.0 ("Switch")) -> ()
            n1026 = global write "全局变量.vi" "zds7"(0.0 ("Switch")) -> ()
            n1027 = global write "全局变量.vi" "sds5"(0.0 ("Switch")) -> ()
          }
        }
      }
      event "井盖 5": Value Change {
        n1028 = event-data() -> ("NewVal"=w1801:bool)  [unwired: 1 in, 5 out]
        n1029 = case shown="真" w1801 {
          frame False {
          }
          frame True {
            n1030 = global write "全局变量.vi" "Switch1"(5.0 ("Switch1")) -> ()
            n1031 = global write "全局变量.vi" "Switch2"(5.0 ("Switch2")) -> ()
            n1032 = global write "全局变量.vi" "Switch"(5.0 ("Switch")) -> ()
          }
        }
        n1033 = property on="自动操作" class="Bool (严格)"() -> ("Value"=w1803:bool)  [unwired: 2 in, 2 out]
        n1034 = And(x=w1801, y=w1803) -> (x .and. y?=w1802:bool)
        n1035 = property on="手动操作" class="Bool (严格)"() -> ("Value"=w1805:bool)  [unwired: 2 in, 2 out]
        n1036 = And(x=w1805, y=w1801) -> (x .and. y?=w1804:bool)
        n1037 = case shown="真" w1802 {
          frame False {
          }
          frame True {
            n1038 = global write "全局变量.vi" "sds4"(0.0 ("Switch")) -> ()
            n1039 = global write "全局变量.vi" "zds3"(0.0 ("Switch")) -> ()
            n1040 = global write "全局变量.vi" "zds2"(0.0 ("Switch")) -> ()
            n1041 = global write "全局变量.vi" "zds1"(0.0 ("Switch")) -> ()
            n1042 = global write "全局变量.vi" "zds8"(0.0 ("Switch")) -> ()
            n1043 = global write "全局变量.vi" "sds6"(0.0 ("Switch")) -> ()
            n1044 = global write "全局变量.vi" "zds7"(0.0 ("Switch")) -> ()
            n1045 = global write "全局变量.vi" "sds5"(1.0 ("Switch")) -> ()
          }
        }
        n1046 = case shown="真" w1804 {
          frame False {
          }
          frame True {
            n1047 = global write "全局变量.vi" "sds4"(0.0 ("Switch")) -> ()
            n1048 = global write "全局变量.vi" "sds3"(0.0 ("Switch")) -> ()
            n1049 = global write "全局变量.vi" "sds2"(0.0 ("Switch")) -> ()
            n1050 = global write "全局变量.vi" "sds1"(0.0 ("Switch")) -> ()
            n1051 = global write "全局变量.vi" "sds8"(0.0 ("Switch")) -> ()
            n1052 = global write "全局变量.vi" "sds6"(0.0 ("Switch")) -> ()
            n1053 = global write "全局变量.vi" "sds7"(0.0 ("Switch")) -> ()
            n1054 = global write "全局变量.vi" "sds5"(1.0 ("Switch")) -> ()
          }
        }
      }
      event "井盖 6": Value Change {
        n1055 = event-data() -> ("NewVal"=w1826:bool)  [unwired: 1 in, 5 out]
        n1056 = case shown="真" w1826 {
          frame False {
          }
          frame True {
            n1057 = global write "全局变量.vi" "Switch1"(6.0 ("Switch1")) -> ()
            n1058 = global write "全局变量.vi" "Switch2"(6.0 ("Switch2")) -> ()
            n1059 = global write "全局变量.vi" "Switch"(6.0 ("Switch")) -> ()
          }
        }
        n1060 = property on="自动操作" class="Bool (严格)"() -> ("Value"=w1827:bool)  [unwired: 2 in, 2 out]
        n1061 = And(x=w1826, y=w1827) -> (x .and. y?=w1825:bool)
        n1062 = property on="手动操作" class="Bool (严格)"() -> ("Value"=w1829:bool)  [unwired: 2 in, 2 out]
        n1063 = And(x=w1829, y=w1826) -> (x .and. y?=w1828:bool)
        n1064 = case shown="真" w1825 {
          frame False {
          }
          frame True {
            n1065 = global write "全局变量.vi" "sds4"(0.0 ("Switch")) -> ()
            n1066 = global write "全局变量.vi" "zds3"(0.0 ("Switch")) -> ()
            n1067 = global write "全局变量.vi" "zds2"(0.0 ("Switch")) -> ()
            n1068 = global write "全局变量.vi" "zds1"(0.0 ("Switch")) -> ()
            n1069 = global write "全局变量.vi" "zds8"(0.0 ("Switch")) -> ()
            n1070 = global write "全局变量.vi" "sds6"(1.0 ("Switch")) -> ()
            n1071 = global write "全局变量.vi" "zds7"(0.0 ("Switch")) -> ()
            n1072 = global write "全局变量.vi" "sds5"(0.0 ("Switch")) -> ()
          }
        }
        n1073 = case shown="真" w1828 {
          frame False {
          }
          frame True {
            n1074 = global write "全局变量.vi" "sds4"(0.0 ("Switch")) -> ()
            n1075 = global write "全局变量.vi" "sds3"(0.0 ("Switch")) -> ()
            n1076 = global write "全局变量.vi" "sds2"(0.0 ("Switch")) -> ()
            n1077 = global write "全局变量.vi" "sds1"(0.0 ("Switch")) -> ()
            n1078 = global write "全局变量.vi" "sds8"(0.0 ("Switch")) -> ()
            n1079 = global write "全局变量.vi" "sds6"(1.0 ("Switch")) -> ()
            n1080 = global write "全局变量.vi" "sds7"(0.0 ("Switch")) -> ()
            n1081 = global write "全局变量.vi" "sds5"(0.0 ("Switch")) -> ()
          }
        }
      }
      event "井盖 7": Value Change {
        n1082 = event-data() -> ("NewVal"=w1851:bool)  [unwired: 1 in, 5 out]
        n1083 = case shown="真" w1851 {
          frame False {
          }
          frame True {
            n1084 = global write "全局变量.vi" "Switch1"(7.0 ("Switch1")) -> ()
            n1085 = global write "全局变量.vi" "Switch2"(7.0 ("Switch2")) -> ()
            n1086 = global write "全局变量.vi" "Switch"(7.0 ("Switch")) -> ()
          }
        }
        n1087 = property on="自动操作" class="Bool (严格)"() -> ("Value"=w1850:bool)  [unwired: 2 in, 2 out]
        n1088 = property on="手动操作" class="Bool (严格)"() -> ("Value"=w1853:bool)  [unwired: 2 in, 2 out]
        n1089 = And(x=w1851, y=w1850) -> (x .and. y?=w1849:bool)
        n1090 = And(x=w1853, y=w1851) -> (x .and. y?=w1852:bool)
        n1091 = case shown="真" w1849 {
          frame False {
          }
          frame True {
            n1092 = global write "全局变量.vi" "sds4"(0.0 ("Switch")) -> ()
            n1093 = global write "全局变量.vi" "zds3"(0.0 ("Switch")) -> ()
            n1094 = global write "全局变量.vi" "zds2"(0.0 ("Switch")) -> ()
            n1095 = global write "全局变量.vi" "zds1"(0.0 ("Switch")) -> ()
            n1096 = global write "全局变量.vi" "zds8"(0.0 ("Switch")) -> ()
            n1097 = global write "全局变量.vi" "sds6"(0.0 ("Switch")) -> ()
            n1098 = global write "全局变量.vi" "zds7"(1.0 ("Switch")) -> ()
            n1099 = global write "全局变量.vi" "sds5"(0.0 ("Switch")) -> ()
          }
        }
        n1100 = case shown="真" w1852 {
          frame False {
          }
          frame True {
            n1101 = global write "全局变量.vi" "sds4"(0.0 ("Switch")) -> ()
            n1102 = global write "全局变量.vi" "sds3"(0.0 ("Switch")) -> ()
            n1103 = global write "全局变量.vi" "sds2"(0.0 ("Switch")) -> ()
            n1104 = global write "全局变量.vi" "sds1"(0.0 ("Switch")) -> ()
            n1105 = global write "全局变量.vi" "sds8"(0.0 ("Switch")) -> ()
            n1106 = global write "全局变量.vi" "sds6"(0.0 ("Switch")) -> ()
            n1107 = global write "全局变量.vi" "sds7"(1.0 ("Switch")) -> ()
            n1108 = global write "全局变量.vi" "sds5"(0.0 ("Switch")) -> ()
          }
        }
      }
      event "井盖 8": Value Change {
        n1109 = event-data() -> ("NewVal"=w1873:bool)  [unwired: 1 in, 5 out]
        n1110 = case shown="真" w1873 {
          frame False {
          }
          frame True {
            n1111 = global write "全局变量.vi" "Switch1"(8.0 ("Switch1")) -> ()
            n1112 = global write "全局变量.vi" "Switch2"(8.0 ("Switch2")) -> ()
            n1113 = global write "全局变量.vi" "Switch"(8.0 ("Switch")) -> ()
          }
        }
        n1114 = property on="自动操作" class="Bool (严格)"() -> ("Value"=w1875:bool)  [unwired: 2 in, 2 out]
        n1115 = And(x=w1873, y=w1875) -> (x .and. y?=w1874:bool)
        n1116 = property on="手动操作" class="Bool (严格)"() -> ("Value"=w1877:bool)  [unwired: 2 in, 2 out]
        n1117 = And(x=w1877, y=w1873) -> (x .and. y?=w1876:bool)
        n1118 = case shown="真" w1874 {
          frame False {
          }
          frame True {
            n1119 = global write "全局变量.vi" "sds4"(0.0 ("Switch")) -> ()
            n1120 = global write "全局变量.vi" "zds3"(0.0 ("Switch")) -> ()
            n1121 = global write "全局变量.vi" "zds2"(0.0 ("Switch")) -> ()
            n1122 = global write "全局变量.vi" "zds1"(0.0 ("Switch")) -> ()
            n1123 = global write "全局变量.vi" "zds8"(1.0 ("Switch")) -> ()
            n1124 = global write "全局变量.vi" "sds6"(0.0 ("Switch")) -> ()
            n1125 = global write "全局变量.vi" "zds7"(0.0 ("Switch")) -> ()
            n1126 = global write "全局变量.vi" "sds5"(0.0 ("Switch")) -> ()
          }
        }
        n1127 = case shown="真" w1876 {
          frame False {
          }
          frame True {
            n1128 = global write "全局变量.vi" "sds4"(0.0 ("Switch")) -> ()
            n1129 = global write "全局变量.vi" "sds3"(0.0 ("Switch")) -> ()
            n1130 = global write "全局变量.vi" "sds2"(0.0 ("Switch")) -> ()
            n1131 = global write "全局变量.vi" "sds1"(0.0 ("Switch")) -> ()
            n1132 = global write "全局变量.vi" "sds8"(1.0 ("Switch")) -> ()
            n1133 = global write "全局变量.vi" "sds6"(0.0 ("Switch")) -> ()
            n1134 = global write "全局变量.vi" "sds7"(0.0 ("Switch")) -> ()
            n1135 = global write "全局变量.vi" "sds5"(0.0 ("Switch")) -> ()
          }
        }
      }
      event "手动操作": Value Change {
        n1136 = event-data() -> ("NewVal"=w1897:bool)  [unwired: 1 in, 5 out]
        n1137 = case shown="真" w1897 {
          frame False {
          }
          frame True {
            n1138 = global write "全局变量.vi" "qiehuan"(1.0 ("qiehuan")) -> ()
          }
        }
      }
      event "自动操作": Value Change {
        n1139 = event-data() -> ("NewVal"=w1899:bool)  [unwired: 1 in, 5 out]
        n1140 = case shown="真" w1899 {
          frame False {
          }
          frame True {
            n1141 = global write "全局变量.vi" "qiehuan"(0.0 ("qiehuan")) -> ()
          }
        }
      }
      event "退出系统": Value Change {
        n1142 = event-data() -> ("NewVal"=w1901:bool)  [unwired: 1 in, 5 out]
        n1143 = case shown="真" w1901 {
          frame False {
          }
          frame True {
            n1144 = flat-sequence {
              frame #0 {
                n1145 = Boolean To (0,1)(Boolean="退出系统") -> (0, 1=w1903:i16)
                n1146 = global write "全局变量.vi" "jieshu"(w1903) -> ()
                n1147 = global write "全局变量.vi" "退出系统"("退出系统") -> ()
                n1148 = call "时间延迟"() -> ()  [unwired: 11 in, 1 out]
              }
              frame #1 {
                n1149 = global write "全局变量.vi" "jieshu"(0.0 ("jieshu")) -> ()
              }
              frame #2 {
                n1150 = Stop(stop? (T)=TRUE ("停止？(T)")) -> ()
              }
            }
          }
        }
      }
    }
  }
  n1151 = while {
    stop <- FALSE stop-if-true
    n1152 = event shown="[2] \"间隔时间4s\": 值改变" {
      selector: _ -> [_ _ _]
      dyn-events: _ -> [_ _ _]
      timeout: _ -> [_ _ _]
      event "间隔时间2s": Value Change {
        n1153 = event-data() -> ("NewVal"=w1909:bool)  [unwired: 1 in, 5 out]
        n1154 = case shown="假" w1909 {
          tunnel: [FALSE ("井盖1") FALSE ("井盖1")] -> w1908
          tunnel: [T1."Disabled and Grayed Out" ("禁用") T1."Disabled and Grayed Out" ("禁用")] -> w1907
          frame False {
          }
          frame True {
          }
        }
        n1155 = property on="井盖1" class="Bool (严格)"("Value"=w1908, "DisabledEnum"=w1907) -> ()  [unwired: 2 in, 2 out]
        n1156 = property on="井盖 3" class="Bool (严格)"("Value"=w1908, "DisabledEnum"=w1907) -> ()  [unwired: 2 in, 2 out]
        n1157 = property on="井盖 2" class="Bool (严格)"("Value"=w1908, "DisabledEnum"=w1907) -> ()  [unwired: 2 in, 2 out]
        n1158 = property on="井盖 4" class="Bool (严格)"("Value"=w1908, "DisabledEnum"=w1907) -> ()  [unwired: 2 in, 2 out]
        n1159 = property on="井盖 6" class="Bool (严格)"("Value"=w1908, "DisabledEnum"=w1907) -> ()  [unwired: 2 in, 2 out]
        n1160 = property on="井盖 5" class="Bool (严格)"("Value"=w1908, "DisabledEnum"=w1907) -> ()  [unwired: 2 in, 2 out]
        n1161 = property on="井盖 8" class="Bool (严格)"("Value"=w1908, "DisabledEnum"=w1907) -> ()  [unwired: 2 in, 2 out]
        n1162 = property on="井盖 7" class="Bool (严格)"("Value"=w1908, "DisabledEnum"=w1907) -> ()  [unwired: 2 in, 2 out]
        n1163 = property on="解锁" class="Bool (严格)"("Value"=w1908, "DisabledEnum"=w1907) -> ()  [unwired: 2 in, 2 out]
        n1164 = property on="开盖" class="Bool (严格)"("Value"=w1908, "DisabledEnum"=w1907) -> ()  [unwired: 2 in, 2 out]
        n1165 = property on="关盖" class="Bool (严格)"("Value"=w1908, "DisabledEnum"=w1907) -> ()  [unwired: 2 in, 2 out]
        n1166 = property on="压紧" class="Bool (严格)"("Value"=w1908, "DisabledEnum"=w1907) -> ()  [unwired: 2 in, 2 out]
        n1167 = property on="锁定" class="Bool (严格)"("Value"=w1908, "DisabledEnum"=w1907) -> ()  [unwired: 2 in, 2 out]
        n1168 = property on="松开" class="Bool (严格)"("Value"=w1908, "DisabledEnum"=w1907) -> ()  [unwired: 2 in, 2 out]
      }
      event "间隔时间3s": Value Change {
        n1169 = event-data() -> ("NewVal"=w1918:bool)  [unwired: 1 in, 5 out]
        n1170 = case shown="假" w1918 {
          tunnel: [w1919 w1921] -> w1915
          tunnel: [w1920 w1922] -> w1914
          tunnel: [w1919 w1921] -> w1917
          tunnel: [w1920 w1922] -> w1916
          frame False {
            (unwired) T1."Disabled and Grayed Out" ("禁用")
            w1919 = FALSE ("井盖1")
            w1920 = T1."Disabled and Grayed Out" ("禁用")
          }
          frame True {
            w1922 = T1."Disabled and Grayed Out" ("禁用")
            w1921 = FALSE ("井盖1")
          }
        }
        n1171 = property on="井盖 3" class="Bool (严格)"("Value"=w1915, "DisabledEnum"=w1914) -> ()  [unwired: 2 in, 2 out]
        n1172 = property on="井盖 2" class="Bool (严格)"("Value"=w1915, "DisabledEnum"=w1914) -> ()  [unwired: 2 in, 2 out]
        n1173 = property on="井盖1" class="Bool (严格)"("Value"=w1915, "DisabledEnum"=w1914) -> ()  [unwired: 2 in, 2 out]
        n1174 = property on="井盖 5" class="Bool (严格)"("Value"=w1915, "DisabledEnum"=w1914) -> ()  [unwired: 2 in, 2 out]
        n1175 = property on="井盖 6" class="Bool (严格)"("Value"=w1915, "DisabledEnum"=w1914) -> ()  [unwired: 2 in, 2 out]
        n1176 = property on="井盖 4" class="Bool (严格)"("Value"=w1915, "DisabledEnum"=w1914) -> ()  [unwired: 2 in, 2 out]
        n1177 = property on="井盖 7" class="Bool (严格)"("Value"=w1915, "DisabledEnum"=w1914) -> ()  [unwired: 2 in, 2 out]
        n1178 = property on="井盖 8" class="Bool (严格)"("Value"=w1915, "DisabledEnum"=w1914) -> ()  [unwired: 2 in, 2 out]
        n1179 = property on="解锁" class="Bool (严格)"("Value"=w1917, "DisabledEnum"=w1916) -> ()  [unwired: 2 in, 2 out]
        n1180 = property on="开盖" class="Bool (严格)"("Value"=w1917, "DisabledEnum"=w1916) -> ()  [unwired: 2 in, 2 out]
        n1181 = property on="关盖" class="Bool (严格)"("Value"=w1917, "DisabledEnum"=w1916) -> ()  [unwired: 2 in, 2 out]
        n1182 = property on="松开" class="Bool (严格)"("Value"=w1917, "DisabledEnum"=w1916) -> ()  [unwired: 2 in, 2 out]
        n1183 = property on="压紧" class="Bool (严格)"("Value"=w1917, "DisabledEnum"=w1916) -> ()  [unwired: 2 in, 2 out]
        n1184 = property on="锁定" class="Bool (严格)"("Value"=w1917, "DisabledEnum"=w1916) -> ()  [unwired: 2 in, 2 out]
      }
      event "间隔时间4s": Value Change {
        n1185 = event-data() -> ("NewVal"=w1929:bool)  [unwired: 1 in, 5 out]
        n1186 = case shown="真" w1929 {
          tunnel: [w1931 w1933] -> w1926
          tunnel: [w1931 w1933] -> w1923
          tunnel: [w1931 w1933] -> w1928
          tunnel: [w1930 w1932] -> w1925
          tunnel: [w1930 w1932] -> w1924
          tunnel: [w1930 w1932] -> w1927
          frame False {
            w1930 = T1."Disabled and Grayed Out" ("禁用")
            w1931 = FALSE ("井盖1")
          }
          frame True {
            w1932 = T1."Disabled and Grayed Out" ("禁用")
            w1933 = FALSE ("井盖1")
          }
        }
        n1187 = property on="井盖 3" class="Bool (严格)"("Value"=w1926, "DisabledEnum"=w1925) -> ()  [unwired: 2 in, 2 out]
        n1188 = property on="井盖1" class="Bool (严格)"("Value"=w1926, "DisabledEnum"=w1925) -> ()  [unwired: 2 in, 2 out]
        n1189 = property on="井盖 2" class="Bool (严格)"("Value"=w1926, "DisabledEnum"=w1925) -> ()  [unwired: 2 in, 2 out]
        n1190 = property on="井盖 4" class="Bool (严格)"("Value"=w1926, "DisabledEnum"=w1925) -> ()  [unwired: 2 in, 2 out]
        n1191 = property on="井盖 8" class="Bool (严格)"("Value"=w1923, "DisabledEnum"=w1924) -> ()  [unwired: 2 in, 2 out]
        n1192 = property on="井盖 7" class="Bool (严格)"("Value"=w1923, "DisabledEnum"=w1924) -> ()  [unwired: 2 in, 2 out]
        n1193 = property on="井盖 6" class="Bool (严格)"("Value"=w1923, "DisabledEnum"=w1924) -> ()  [unwired: 2 in, 2 out]
        n1194 = property on="井盖 5" class="Bool (严格)"("Value"=w1923, "DisabledEnum"=w1924) -> ()  [unwired: 2 in, 2 out]
        n1195 = property on="松开" class="Bool (严格)"("Value"=w1928, "DisabledEnum"=w1927) -> ()  [unwired: 2 in, 2 out]
        n1196 = property on="解锁" class="Bool (严格)"("Value"=w1928, "DisabledEnum"=w1927) -> ()  [unwired: 2 in, 2 out]
        n1197 = property on="关盖" class="Bool (严格)"("Value"=w1928, "DisabledEnum"=w1927) -> ()  [unwired: 2 in, 2 out]
        n1198 = property on="开盖" class="Bool (严格)"("Value"=w1928, "DisabledEnum"=w1927) -> ()  [unwired: 2 in, 2 out]
        n1199 = property on="压紧" class="Bool (严格)"("Value"=w1928, "DisabledEnum"=w1927) -> ()  [unwired: 2 in, 2 out]
        n1200 = property on="锁定" class="Bool (严格)"("Value"=w1928, "DisabledEnum"=w1927) -> ()  [unwired: 2 in, 2 out]
      }
    }
  }
  n1201 = while {
    stop <- FALSE stop-if-true
    n1202 = event shown="[2] \"间隔时间3s\": 值改变" {
      selector: _ -> [_ _ _ _]
      dyn-events: _ -> [_ _ _ _]
      timeout: _ -> [_ _ _ _]
      event Timeout {
        n1203 = event-data() -> ()  [unwired: 1 in, 3 out]
      }
      event "间隔时间2s": Value Change {
        n1204 = event-data() -> ("NewVal"=w1937:bool)  [unwired: 1 in, 5 out]
        n1205 = case shown="真" w1937 {
          tunnel: [FALSE ("间隔时间3s") FALSE ("间隔时间3s")] -> w1935
          tunnel: [T1."Enabled" ("禁用") T1."Disabled and Grayed Out" ("禁用")] -> w1936
          frame False {
          }
          frame True {
            # "压紧延迟"
            # "关盖延迟"
            # "解锁延迟"
            # "锁定延迟"
            # "开盖延迟"
            # "松开延迟"
            n1206 = global write "全局变量.vi" "t2"(2.0 ("t2")) -> ()
            n1207 = global write "全局变量.vi" "t3"(2.0 ("t3")) -> ()
            n1208 = global write "全局变量.vi" "t1"(2.0 ("t1")) -> ()
            n1209 = global write "全局变量.vi" "t6"(2.0 ("t6")) -> ()
            n1210 = global write "全局变量.vi" "t4"(2.0 ("t4")) -> ()
            n1211 = global write "全局变量.vi" "t5"(2.0 ("t5")) -> ()
          }
        }
        n1212 = property on="间隔时间3s" class="Bool (严格)"("Value"=w1935, "DisabledEnum"=w1936) -> ()  [unwired: 2 in, 2 out]
        n1213 = property on="间隔时间4s" class="Bool (严格)"("Value"=w1935, "DisabledEnum"=w1936) -> ()  [unwired: 2 in, 2 out]
      }
      event "间隔时间3s": Value Change {
        n1214 = event-data() -> ("NewVal"=w1950:bool)  [unwired: 1 in, 5 out]
        n1215 = case shown="真" w1950 {
          tunnel: [FALSE ("间隔时间2s") FALSE ("间隔时间2s")] -> w1948
          tunnel: [T1."Enabled" ("禁用") T1."Disabled and Grayed Out" ("禁用")] -> w1949
          frame False {
          }
          frame True {
            n1216 = global write "全局变量.vi" "t2"(3.0 ("t2")) -> ()
            n1217 = global write "全局变量.vi" "t3"(3.0 ("t3")) -> ()
            n1218 = global write "全局变量.vi" "t1"(3.0 ("t1")) -> ()
            n1219 = global write "全局变量.vi" "t6"(3.0 ("t6")) -> ()
            n1220 = global write "全局变量.vi" "t4"(3.0 ("t4")) -> ()
            n1221 = global write "全局变量.vi" "t5"(3.0 ("t5")) -> ()
          }
        }
        n1222 = property on="间隔时间2s" class="Bool (严格)"("Value"=w1948, "DisabledEnum"=w1949) -> ()  [unwired: 2 in, 2 out]
        n1223 = property on="间隔时间4s" class="Bool (严格)"("Value"=w1948, "DisabledEnum"=w1949) -> ()  [unwired: 2 in, 2 out]
      }
      event "间隔时间4s": Value Change {
        n1224 = event-data() -> ("NewVal"=w1963:bool)  [unwired: 1 in, 5 out]
        n1225 = case shown="假" w1963 {
          tunnel: [FALSE ("间隔时间2s") FALSE ("间隔时间2s")] -> w1962
          tunnel: [T1."Enabled" ("禁用") T1."Disabled and Grayed Out" ("禁用")] -> w1961
          frame False {
          }
          frame True {
            n1226 = global write "全局变量.vi" "t2"(4.0 ("t2")) -> ()
            n1227 = global write "全局变量.vi" "t3"(4.0 ("t3")) -> ()
            n1228 = global write "全局变量.vi" "t1"(4.0 ("t1")) -> ()
            n1229 = global write "全局变量.vi" "t6"(4.0 ("t6")) -> ()
            n1230 = global write "全局变量.vi" "t4"(4.0 ("t4")) -> ()
            n1231 = global write "全局变量.vi" "t5"(4.0 ("t5")) -> ()
          }
        }
        n1232 = property on="间隔时间2s" class="Bool (严格)"("Value"=w1962, "DisabledEnum"=w1961) -> ()  [unwired: 2 in, 2 out]
        n1233 = property on="间隔时间3s" class="Bool (严格)"("Value"=w1962, "DisabledEnum"=w1961) -> ()  [unwired: 2 in, 2 out]
      }
    }
  }
  n1234 = while {
    stop <- FALSE stop-if-true
    n1235 = Boolean To (0,1)(Boolean="系统启动") -> (0, 1=w1987:i16)
    n1236 = global write "全局变量.vi" "start"(w1987) -> ()
    n1237 = case shown="真" "系统启动" {
      frame False {
      }
      frame True {
        n1238 = global read "全局变量.vi" "关盖换向阀"() -> (→"关盖换向阀":bool)
        n1239 = global read "全局变量.vi" "关盖指令2"() -> (→"关盖指令2":bool)
        n1240 = global read "全局变量.vi" "解锁到位"() -> (→"解锁到位":bool)
        n1241 = global read "全局变量.vi" "关盖指令1"() -> (→"关盖指令1":bool)
        n1242 = global read "全局变量.vi" "关盖到位2"() -> (→"关盖到位2":bool)
        n1243 = global read "全局变量.vi" "关盖缓冲"() -> (→"关盖缓冲":bool)
        n1244 = global read "全局变量.vi" "关盖到位1"() -> (→"关盖到位1":bool)
        n1245 = global read "全局变量.vi" "开盖到位1"() -> (→"开盖到位1":bool)
        n1246 = global read "全局变量.vi" "松开到位"() -> (→"松开到位":bool)
        n1247 = Boolean To (0,1)(Boolean="调试模式") -> (0, 1=w1990:i16)
        n1248 = case shown="真" "调试模式" {
          frame False {
          }
          frame True {
            n1249 = call "调试模式.vi"() -> ()  [unwired: 12 in]
          }
        }
        n1250 = global write "全局变量.vi" "tiaoshimoshi"(w1990) -> ()
        n1251 = global read "全局变量.vi" "松开换向阀"() -> (→"松开换向阀":bool)
        n1252 = global read "全局变量.vi" "开盖指令2"() -> (→"开盖指令2":bool)
        n1253 = global read "全局变量.vi" "压紧换向阀"() -> (→"压紧换向阀":bool)
        n1254 = global read "全局变量.vi" "开盖换向阀"() -> (→"开盖换向阀":bool)
        n1255 = global read "全局变量.vi" "压紧到位"() -> (→"压紧到位":bool)
        n1256 = global read "全局变量.vi" "开盖指令1"() -> (→"开盖指令1":bool)
        n1257 = global read "全局变量.vi" "开盖到位2"() -> (→"开盖到位2":bool)
        n1258 = global read "全局变量.vi" "锁定到位"() -> (→"锁定到位":bool)
        n1259 = global read "全局变量.vi" "开盖缓冲"() -> (→"开盖缓冲":bool)
        n1260 = Boolean To (0,1)(Boolean="自动操作") -> (0, 1=w2013:i16)
        n1261 = global write "全局变量.vi" "qidongzd"(w2013) -> ()
        n1262 = Boolean To (0,1)(Boolean="井盖 7") -> (0, 1=w2016:i16)
        n1263 = Boolean To (0,1)(Boolean="井盖 6") -> (0, 1=w2017:i16)
        n1264 = Boolean To (0,1)(Boolean="井盖 8") -> (0, 1=w2015:i16)
        n1265 = Boolean To (0,1)(Boolean="手动操作") -> (0, 1=w2014:i16)
        n1266 = Boolean To (0,1)(Boolean="井盖 5") -> (0, 1=w2018:i16)
        n1267 = Boolean To (0,1)(Boolean="井盖 3") -> (0, 1=w2020:i16)
        n1268 = Boolean To (0,1)(Boolean="井盖 4") -> (0, 1=w2019:i16)
        n1269 = Boolean To (0,1)(Boolean="井盖 2") -> (0, 1=w2021:i16)
        n1270 = Boolean To (0,1)(Boolean="井盖1") -> (0, 1=w2022:i16)
        n1271 = global write "全局变量.vi" "qidongsd"(w2014) -> ()
        n1272 = global write "全局变量.vi" "kaishi7"(w2016) -> ()
        n1273 = global write "全局变量.vi" "kaishi6"(w2017) -> ()
        n1274 = global write "全局变量.vi" "kaishi8"(w2015) -> ()
        n1275 = global write "全局变量.vi" "kaishi5"(w2018) -> ()
        n1276 = global write "全局变量.vi" "kaishi3"(w2020) -> ()
        n1277 = global write "全局变量.vi" "kaishi4"(w2019) -> ()
        n1278 = global write "全局变量.vi" "kaishi2"(w2021) -> ()
        n1279 = global write "全局变量.vi" "kaishi1"(w2022) -> ()
        n1280 = Boolean To (0,1)(Boolean="解锁") -> (0, 1=w2009:i16)
        n1281 = Boolean To (0,1)(Boolean="关盖") -> (0, 1=w2007:i16)
        n1282 = Boolean To (0,1)(Boolean="松开") -> (0, 1=w2011:i16)
        n1283 = Boolean To (0,1)(Boolean="开盖") -> (0, 1=w2005:i16)
        n1284 = Boolean To (0,1)(Boolean="压紧") -> (0, 1=w2003:i16)
        n1285 = Boolean To (0,1)(Boolean="锁定") -> (0, 1=w2001:i16)
        n1286 = global write "全局变量.vi" "guangai"(w2007) -> ()
        n1287 = global write "全局变量.vi" "songkai"(w2011) -> ()
        n1288 = global write "全局变量.vi" "jiesuo"(w2009) -> ()
        n1289 = global write "全局变量.vi" "suoding"(w2001) -> ()
        n1290 = global write "全局变量.vi" "kaigai"(w2005) -> ()
        n1291 = global write "全局变量.vi" "yajin"(w2003) -> ()
      }
    }
    n1292 = global read "全局变量.vi" "已开盖次数"() -> (→"已开盖次数":dbl)
    n1293 = global read "全局变量.vi" "guangaitm"() -> (→"关盖时间":dbl)
    n1294 = global read "全局变量.vi" "jiesuotm"() -> (→"解锁时间":dbl)
    n1295 = global read "全局变量.vi" "songkaitm"() -> (→"松开时间":dbl)
    n1296 = global read "全局变量.vi" "suodingtm"() -> (→"锁定时间":dbl)
    n1297 = global read "全局变量.vi" "kaigaitm"() -> (→"开盖时间":dbl)
    n1298 = global read "全局变量.vi" "yajintm"() -> (→"压紧时间":dbl)
    n1299 = global write "全局变量.vi" "kaigaicishu"("开盖次数设置") -> ()
    n1300 = Format Date/Time String(time format string (%c)="%Y/%m/%d" ("时间格式字符串(%c)")) -> (date/time string=→"日期":string)  [unwired: 2 in]
    n1301 = Format Date/Time String(time format string (%c)="%H : %M : %S" ("时间格式字符串(%c)")) -> (date/time string=→"时间":string)  [unwired: 2 in]
  }
  n1302 = flat-sequence {
    frame #0 {
      n1303 = property on="系统启动" class="Bool (严格)"("Value"=FALSE ("系统启动"), "DisabledEnum"=T1."Enabled" ("禁用")) -> ()  [unwired: 2 in, 2 out]
      n1304 = property on="自动操作" class="Bool (严格)"("Value"=FALSE ("自动操作"), "DisabledEnum"=T1."Disabled and Grayed Out" ("禁用")) -> ()  [unwired: 2 in, 2 out]
      n1305 = property on="井盖 3" class="Bool (严格)"("Value"=FALSE ("井盖 3"), "DisabledEnum"=T1."Disabled and Grayed Out" ("禁用")) -> ()  [unwired: 2 in, 2 out]
      n1306 = property on="退出系统" class="Bool (严格)"("Value"=FALSE ("退出系统"), "DisabledEnum"=T1."Enabled" ("禁用")) -> ()  [unwired: 2 in, 2 out]
      n1307 = property on="井盖 4" class="Bool (严格)"("Value"=FALSE ("井盖 4"), "DisabledEnum"=T1."Disabled and Grayed Out" ("禁用")) -> ()  [unwired: 2 in, 2 out]
      n1308 = property on="间隔时间2s" class="Bool (严格)"("Value"=FALSE ("间隔时间2s"), "DisabledEnum"=T1."Disabled and Grayed Out" ("禁用")) -> ()  [unwired: 2 in, 2 out]
      n1309 = property on="手动操作" class="Bool (严格)"("Value"=FALSE ("手动操作"), "DisabledEnum"=T1."Disabled and Grayed Out" ("禁用")) -> ()  [unwired: 2 in, 2 out]
      n1310 = property on="井盖1" class="Bool (严格)"("Value"=FALSE ("井盖1"), "DisabledEnum"=T1."Disabled and Grayed Out" ("禁用")) -> ()  [unwired: 2 in, 2 out]
      n1311 = property on="解锁" class="Bool (严格)"("Value"=FALSE ("解锁"), "DisabledEnum"=T1."Disabled and Grayed Out" ("禁用")) -> ()  [unwired: 2 in, 2 out]
      n1312 = property on="井盖 7" class="Bool (严格)"("Value"=FALSE ("井盖 7"), "DisabledEnum"=T1."Disabled and Grayed Out" ("禁用")) -> ()  [unwired: 2 in, 2 out]
      n1313 = property on="松开" class="Bool (严格)"("Value"=FALSE ("松开"), "DisabledEnum"=T1."Disabled and Grayed Out" ("禁用")) -> ()  [unwired: 2 in, 2 out]
      n1314 = property on="间隔时间3s" class="Bool (严格)"("Value"=FALSE ("间隔时间3s"), "DisabledEnum"=T1."Disabled and Grayed Out" ("禁用")) -> ()  [unwired: 2 in, 2 out]
      n1315 = property on="井盖 5" class="Bool (严格)"("Value"=FALSE ("井盖 5"), "DisabledEnum"=T1."Disabled and Grayed Out" ("禁用")) -> ()  [unwired: 2 in, 2 out]
      n1316 = property on="开盖" class="Bool (严格)"("Value"=FALSE ("开盖"), "DisabledEnum"=T1."Disabled and Grayed Out" ("禁用")) -> ()  [unwired: 2 in, 2 out]
      n1317 = property on="调试模式" class="Bool (严格)"("Value"=FALSE ("调试模式"), "DisabledEnum"=T1."Disabled and Grayed Out" ("禁用")) -> ()  [unwired: 2 in, 2 out]
      n1318 = property on="井盖 6" class="Bool (严格)"("Value"=FALSE ("井盖 6"), "DisabledEnum"=T1."Disabled and Grayed Out" ("禁用")) -> ()  [unwired: 2 in, 2 out]
      n1319 = property on="关盖" class="Bool (严格)"("Value"=FALSE ("关盖"), "DisabledEnum"=T1."Disabled and Grayed Out" ("禁用")) -> ()  [unwired: 2 in, 2 out]
      n1320 = property on="间隔时间4s" class="Bool (严格)"("Value"=FALSE ("间隔时间4s"), "DisabledEnum"=T1."Disabled and Grayed Out" ("禁用")) -> ()  [unwired: 2 in, 2 out]
      n1321 = property on="井盖 8" class="Bool (严格)"("Value"=FALSE ("井盖 8"), "DisabledEnum"=T1."Disabled and Grayed Out" ("禁用")) -> ()  [unwired: 2 in, 2 out]
      n1322 = property on="锁定" class="Bool (严格)"("Value"=FALSE ("锁定"), "DisabledEnum"=T1."Disabled and Grayed Out" ("禁用")) -> ()  [unwired: 2 in, 2 out]
      n1323 = property on="井盖 2" class="Bool (严格)"("Value"=FALSE ("井盖 2"), "DisabledEnum"=T1."Disabled and Grayed Out" ("禁用")) -> ()  [unwired: 2 in, 2 out]
      n1324 = property on="压紧" class="Bool (严格)"("Value"=FALSE ("压紧"), "DisabledEnum"=T1."Disabled and Grayed Out" ("禁用")) -> ()  [unwired: 2 in, 2 out]
    }
  }
  n1325 = while {
    stop <- FALSE stop-if-true
    n1326 = case shown="真" "保存时间" {
      frame False {
      }
      frame True {
        n1327 = global read "全局变量.vi" "kaigaitm"() -> (w2124:dbl)
        n1328 = global read "全局变量.vi" "yajintm"() -> (w2130:dbl)
        n1329 = global read "全局变量.vi" "suodingtm"() -> (w2128:dbl)
        n1330 = global read "全局变量.vi" "guangaitm"() -> (w2088:dbl)
        n1331 = global read "全局变量.vi" "songkaitm"() -> (w2126:dbl)
        n1332 = global read "全局变量.vi" "jiesuotm"() -> (w2122:dbl)
        n1333 = Number To Fractional String(number=w2130) -> (F-format string=w2129:string)  [unwired: 3 in]
        n1334 = Number To Fractional String(number=w2124) -> (F-format string=w2123:string)  [unwired: 3 in]
        n1335 = Number To Fractional String(number=w2128) -> (F-format string=w2127:string)  [unwired: 3 in]
        n1336 = Number To Fractional String(number=w2122) -> (F-format string=w2121:string)  [unwired: 3 in]
        n1337 = Number To Fractional String(number=w2088) -> (F-format string=w2120:string)  [unwired: 3 in]
        n1338 = Number To Fractional String(number=w2126) -> (F-format string=w2125:string)  [unwired: 3 in]
        n1339 = Concatenate Strings("开盖时间为：" ("字符串"), w2123, "s" ("字符串"), "\r") -> (w2133:string)
        n1340 = Concatenate Strings("锁定时间为：" ("字符串"), w2127, "s" ("字符串"), "\r") -> (w2135:string)
        n1341 = Concatenate Strings("压紧时间为：" ("字符串"), w2129, "s" ("字符串"), "\r") -> (w2136:string)
        n1342 = Concatenate Strings("松开时间为：" ("字符串"), w2125, "s" ("字符串"), "\r") -> (w2134:string)
        n1343 = Concatenate Strings("解锁时间为：" ("字符串"), w2121, "s" ("字符串"), "\r") -> (w2132:string)
        n1344 = Concatenate Strings("关盖时间为：" ("字符串"), w2120, "s" ("字符串"), "\r") -> (w2131:string)
        n1345 = Concatenate Strings(w2131, w2132, w2133, w2134, w2135, w2136) -> (w2095:string)
        n1346 = property on="保存路径" class="Path"() -> ("Value"=w2089:path)  [unwired: 2 in, 2 out]
        n1347 = Format Date/Time String(time format string (%c)="%m-%d_%H-%M-%S" ("时间格式字符串(%c)")) -> (date/time string=w2093:string)  [unwired: 2 in]
        n1348 = Concatenate Strings("时间记录", w2093, ".txt" ("字符串")) -> (w2096:string)
        n1349 = Build Path(base path=w2089, name or relative path=w2096) -> (appended path=w2100:path)
        n1350 = Open/Create/Replace File(file path (use dialog)=w2100, operation (0:open)=T2."open or create" ("操作(0:open)")) -> (refnum out=w2099:refnum<file>)  [unwired: 4 in, 2 out]
        n1351 = Set File Position(refnum=w2099, from (0:start)=enum16{"start", "end", "current"}."end" ("自（0:起始）")) -> (refnum out=w2097:refnum<file>)  [unwired: 2 in, 1 out]
        n1352 = Write to Text File(file (use dialog)=w2097, text=w2095) -> (refnum out=w2101:refnum<file>)  [unwired: 2 in, 2 out]
        n1353 = Close File(refnum=w2101) -> ()  [unwired: 1 in, 2 out]
      }
    }
    n1354 = Wait (ms)(milliseconds to wait=u32 40 ("等待时间（毫秒）")) -> ()  [unwired: 1 out]
  }
  n1355 = while {
    stop <- FALSE stop-if-true
    n1356 = event shown="[1] \"系统启动\": 值改变" {
      selector: _ -> [_ _ _ _]
      dyn-events: _ -> [_ _ _ _]
      timeout: _ -> [_ _ _ _]
      event Timeout {
        n1357 = event-data() -> ()  [unwired: 1 in, 3 out]
      }
      event "系统启动": Value Change {
        n1358 = event-data() -> ("NewVal"=w2148:bool)  [unwired: 1 in, 5 out]
        n1359 = case shown="真" w2148 {
          tunnel: [w2150 w2157] -> w2145
          tunnel: [w2149 w2154] -> w2141
          tunnel: [w2150 w2157] -> w2147
          tunnel: [w2150 w2157] -> w2146
          tunnel: [w2149 T1."Enabled" ("禁用")] -> w2138
          tunnel: [w2149 w2154] -> w2143
          tunnel: [w2150 FALSE ("调试模式")] -> w2144
          tunnel: [w2150 FALSE ("井盖 5")] -> w2142
          tunnel: [w2150 FALSE ("间隔时间4s")] -> w2140
          tunnel: [w2149 T1."Enabled" ("禁用")] -> w2139
          frame False {
            w2150 = FALSE ("调试模式")
            w2149 = T1."Disabled and Grayed Out" ("禁用")
          }
          frame True {
            w2154 = T1."Disabled and Grayed Out" ("禁用")
            w2157 = FALSE ("调试模式")
          }
        }
        n1360 = property on="间隔时间2s" class="Bool (严格)"("Value"=w2140, "DisabledEnum"=w2139) -> ()  [unwired: 2 in, 2 out]
        n1361 = property on="间隔时间3s" class="Bool (严格)"("Value"=w2140, "DisabledEnum"=w2139) -> ()  [unwired: 2 in, 2 out]
        n1362 = property on="间隔时间4s" class="Bool (严格)"("Value"=w2140, "DisabledEnum"=w2139) -> ()  [unwired: 2 in, 2 out]
        n1363 = property on="调试模式" class="Bool (严格)"("Value"=w2145, "DisabledEnum"=w2138) -> ()  [unwired: 2 in, 2 out]
        n1364 = property on="自动操作" class="Bool (严格)"("Value"=w2147, "DisabledEnum"=w2138) -> ()  [unwired: 2 in, 2 out]
        n1365 = property on="手动操作" class="Bool (严格)"("Value"=w2146, "DisabledEnum"=w2138) -> ()  [unwired: 2 in, 2 out]
        n1366 = property on="井盖 8" class="Bool (严格)"("Value"=w2142, "DisabledEnum"=w2141) -> ()  [unwired: 2 in, 2 out]
        n1367 = property on="井盖 5" class="Bool (严格)"("Value"=w2142, "DisabledEnum"=w2141) -> ()  [unwired: 2 in, 2 out]
        n1368 = property on="井盖1" class="Bool (严格)"("Value"=w2142, "DisabledEnum"=w2141) -> ()  [unwired: 2 in, 2 out]
        n1369 = property on="井盖 2" class="Bool (严格)"("Value"=w2142, "DisabledEnum"=w2141) -> ()  [unwired: 2 in, 2 out]
        n1370 = property on="井盖 3" class="Bool (严格)"("Value"=w2142, "DisabledEnum"=w2141) -> ()  [unwired: 2 in, 2 out]
        n1371 = property on="井盖 4" class="Bool (严格)"("Value"=w2142, "DisabledEnum"=w2141) -> ()  [unwired: 2 in, 2 out]
        n1372 = property on="松开" class="Bool (严格)"("Value"=w2144, "DisabledEnum"=w2143) -> ()  [unwired: 2 in, 2 out]
        n1373 = property on="解锁" class="Bool (严格)"("Value"=w2144, "DisabledEnum"=w2143) -> ()  [unwired: 2 in, 2 out]
        n1374 = property on="开盖" class="Bool (严格)"("Value"=w2144, "DisabledEnum"=w2143) -> ()  [unwired: 2 in, 2 out]
        n1375 = property on="关盖" class="Bool (严格)"("Value"=w2144, "DisabledEnum"=w2143) -> ()  [unwired: 2 in, 2 out]
        n1376 = property on="井盖 6" class="Bool (严格)"("Value"=w2142, "DisabledEnum"=w2141) -> ()  [unwired: 2 in, 2 out]
        n1377 = property on="压紧" class="Bool (严格)"("Value"=w2144, "DisabledEnum"=w2143) -> ()  [unwired: 2 in, 2 out]
        n1378 = property on="锁定" class="Bool (严格)"("Value"=w2144, "DisabledEnum"=w2143) -> ()  [unwired: 2 in, 2 out]
        n1379 = property on="井盖 7" class="Bool (严格)"("Value"=w2142, "DisabledEnum"=w2141) -> ()  [unwired: 2 in, 2 out]
      }
      event "手动操作": Value Change {
        n1380 = event-data() -> ("NewVal"=w2164:bool)  [unwired: 1 in, 5 out]
        n1381 = case shown="真" w2164 {
          tunnel: [w2167 w2173] -> w2162
          tunnel: [w2168 T1."Enabled" ("禁用")] -> w2163
          tunnel: [w2167 w2173] -> w2161
          tunnel: [w2168 T1."Disabled and Grayed Out" ("禁用")] -> w2160
          tunnel: [FALSE ("自动操作") FALSE ("自动操作")] -> w2159
          tunnel: [T1."Enabled" ("禁用") T1."Disabled and Grayed Out" ("禁用")] -> w2158
          frame False {
            w2168 = T1."Disabled and Grayed Out" ("禁用")
            w2167 = FALSE ("自动操作")
          }
          frame True {
            w2173 = FALSE ("自动操作")
          }
        }
        n1382 = property on="自动操作" class="Bool (严格)"("Value"=w2159, "DisabledEnum"=w2158) -> ()  [unwired: 2 in, 2 out]
        n1383 = property on="井盖1" class="Bool (严格)"("Value"=w2162, "DisabledEnum"=w2163) -> ()  [unwired: 2 in, 2 out]
        n1384 = property on="井盖 2" class="Bool (严格)"("Value"=w2162, "DisabledEnum"=w2163) -> ()  [unwired: 2 in, 2 out]
        n1385 = property on="井盖 4" class="Bool (严格)"("Value"=w2162, "DisabledEnum"=w2163) -> ()  [unwired: 2 in, 2 out]
        n1386 = property on="井盖 3" class="Bool (严格)"("Value"=w2162, "DisabledEnum"=w2163) -> ()  [unwired: 2 in, 2 out]
        n1387 = property on="井盖 6" class="Bool (严格)"("Value"=w2162, "DisabledEnum"=w2163) -> ()  [unwired: 2 in, 2 out]
        n1388 = property on="井盖 5" class="Bool (严格)"("Value"=w2162, "DisabledEnum"=w2163) -> ()  [unwired: 2 in, 2 out]
        n1389 = property on="井盖 8" class="Bool (严格)"("Value"=w2162, "DisabledEnum"=w2163) -> ()  [unwired: 2 in, 2 out]
        n1390 = property on="井盖 7" class="Bool (严格)"("Value"=w2162, "DisabledEnum"=w2163) -> ()  [unwired: 2 in, 2 out]
        n1391 = property on="开盖" class="Bool (严格)"("Value"=w2161, "DisabledEnum"=w2160) -> ()  [unwired: 2 in, 2 out]
        n1392 = property on="压紧" class="Bool (严格)"("Value"=w2161, "DisabledEnum"=w2160) -> ()  [unwired: 2 in, 2 out]
        n1393 = property on="松开" class="Bool (严格)"("Value"=w2161, "DisabledEnum"=w2160) -> ()  [unwired: 2 in, 2 out]
        n1394 = property on="锁定" class="Bool (严格)"("Value"=w2161, "DisabledEnum"=w2160) -> ()  [unwired: 2 in, 2 out]
        n1395 = property on="解锁" class="Bool (严格)"("Value"=w2161, "DisabledEnum"=w2160) -> ()  [unwired: 2 in, 2 out]
        n1396 = property on="关盖" class="Bool (严格)"("Value"=w2161, "DisabledEnum"=w2160) -> ()  [unwired: 2 in, 2 out]
      }
      event "自动操作": Value Change {
        n1397 = event-data() -> ("NewVal"=w2180:bool)  [unwired: 1 in, 5 out]
        n1398 = case shown="真" w2180 {
          tunnel: [FALSE ("手动操作") FALSE ("手动操作")] -> w2179
          tunnel: [T1."Enabled" ("禁用") T1."Disabled and Grayed Out" ("禁用")] -> w2178
          tunnel: [FALSE ("井盖1") FALSE ("井盖1")] -> w2177
          tunnel: [T1."Disabled and Grayed Out" ("禁用") T1."Enabled" ("禁用")] -> w2176
          tunnel: [FALSE ("松开") FALSE ("松开")] -> w2175
          tunnel: [T1."Disabled and Grayed Out" ("禁用") T1."Disabled and Grayed Out" ("禁用")] -> w2174
          frame False {
          }
          frame True {
          }
        }
        n1399 = property on="手动操作" class="Bool (严格)"("Value"=w2179, "DisabledEnum"=w2178) -> ()  [unwired: 2 in, 2 out]
        n1400 = property on="井盖 5" class="Bool (严格)"("Value"=w2177, "DisabledEnum"=w2176) -> ()  [unwired: 2 in, 2 out]
        n1401 = property on="井盖1" class="Bool (严格)"("Value"=w2177, "DisabledEnum"=w2176) -> ()  [unwired: 2 in, 2 out]
        n1402 = property on="井盖 6" class="Bool (严格)"("Value"=w2177, "DisabledEnum"=w2176) -> ()  [unwired: 2 in, 2 out]
        n1403 = property on="井盖 2" class="Bool (严格)"("Value"=w2177, "DisabledEnum"=w2176) -> ()  [unwired: 2 in, 2 out]
        n1404 = property on="井盖 7" class="Bool (严格)"("Value"=w2177, "DisabledEnum"=w2176) -> ()  [unwired: 2 in, 2 out]
        n1405 = property on="井盖 3" class="Bool (严格)"("Value"=w2177, "DisabledEnum"=w2176) -> ()  [unwired: 2 in, 2 out]
        n1406 = property on="井盖 8" class="Bool (严格)"("Value"=w2177, "DisabledEnum"=w2176) -> ()  [unwired: 2 in, 2 out]
        n1407 = property on="井盖 4" class="Bool (严格)"("Value"=w2177, "DisabledEnum"=w2176) -> ()  [unwired: 2 in, 2 out]
        n1408 = property on="关盖" class="Bool (严格)"("Value"=w2175, "DisabledEnum"=w2174) -> ()  [unwired: 2 in, 2 out]
        n1409 = property on="开盖" class="Bool (严格)"("Value"=w2175, "DisabledEnum"=w2174) -> ()  [unwired: 2 in, 2 out]
        n1410 = property on="压紧" class="Bool (严格)"("Value"=w2175, "DisabledEnum"=w2174) -> ()  [unwired: 2 in, 2 out]
        n1411 = property on="锁定" class="Bool (严格)"("Value"=w2175, "DisabledEnum"=w2174) -> ()  [unwired: 2 in, 2 out]
        n1412 = property on="松开" class="Bool (严格)"("Value"=w2175, "DisabledEnum"=w2174) -> ()  [unwired: 2 in, 2 out]
        n1413 = property on="解锁" class="Bool (严格)"("Value"=w2175, "DisabledEnum"=w2174) -> ()  [unwired: 2 in, 2 out]
      }
    }
  }
  n1414 = while {
    shift-right: [w2277] -> _
    shift-left: w217 -> [w2202]
    shift-left: w217 -> [w2281]
    shift-right: [w2267] -> _
    shift-left: w216 -> [w2201]
    shift-left: w216 -> [w2271]
    shift-right: [w2217] -> _
    shift-left: w215 -> [w2200]
    shift-left: w215 -> [w2218]
    shift-right: [w2215] -> _
    shift-left: w214 -> [w2199]
    shift-left: w214 -> [w2216]
    shift-right: [w2213] -> _
    shift-left: w213 -> [w2198]
    shift-left: w213 -> [w2214]
    shift-right: [w2211] -> _
    shift-left: w212 -> [w2197]
    shift-left: w212 -> [w2212]
    shift-right: [w2209] -> _
    shift-left: w211 -> [w2196]
    shift-left: w211 -> [w2210]
    shift-right: [w2207] -> _
    shift-left: w210 -> [w2195]
    shift-left: w210 -> [w2208]
    shift-right: [w2205] -> _
    shift-left: w209 -> [w2194]
    shift-left: w209 -> [w2206]
    shift-right: [w2203] -> _
    shift-left: w208 -> [w2193]
    shift-left: w208 -> [w2204]
    stop <- FALSE stop-if-true
    n1415 = Not Equal?(x=w2193, y=w2204) -> (x != y?=w2223:bool)
    n1416 = Not Equal?(x=w2198, y=w2214) -> (x != y?=w2253:bool)
    n1417 = Not Equal?(x=w2200, y=w2218) -> (x != y?=w2265:bool)
    n1418 = Not Equal?(x=w2196, y=w2210) -> (x != y?=w2241:bool)
    n1419 = Equal?(x=w2193, y=TRUE) -> (x = y?=w2222:bool)
    n1420 = Not Equal?(x=w2197, y=w2212) -> (x != y?=w2247:bool)
    n1421 = Equal?(x=w2198, y=TRUE) -> (x = y?=w2252:bool)
    n1422 = Not Equal?(x=w2194, y=w2206) -> (x != y?=w2229:bool)
    n1423 = Equal?(x=w2200, y=TRUE) -> (x = y?=w2264:bool)
    n1424 = Equal?(x=w2196, y=TRUE) -> (x = y?=w2240:bool)
    n1425 = Not Equal?(x=w2195, y=w2208) -> (x != y?=w2235:bool)
    n1426 = Equal?(x=w2197, y=TRUE) -> (x = y?=w2246:bool)
    n1427 = Not Equal?(x=w2199, y=w2216) -> (x != y?=w2259:bool)
    n1428 = Equal?(x=w2194, y=TRUE) -> (x = y?=w2228:bool)
    n1429 = Equal?(x=w2195, y=TRUE) -> (x = y?=w2234:bool)
    n1430 = And(x=w2223, y=w2222) -> (x .and. y?=w2221:bool)
    n1431 = Equal?(x=w2199, y=TRUE) -> (x = y?=w2258:bool)
    n1432 = And(x=w2253, y=w2252) -> (x .and. y?=w2251:bool)
    n1433 = Not Equal?(x=w2202, y=w2281) -> (x != y?=w2279:bool)
    n1434 = And(x=w2265, y=w2264) -> (x .and. y?=w2263:bool)
    n1435 = And(x=w2241, y=w2240) -> (x .and. y?=w2239:bool)
    n1436 = Not Equal?(x=w2201, y=w2271) -> (x != y?=w2273:bool)
    n1437 = And(x=w2247, y=w2246) -> (x .and. y?=w2245:bool)
    n1438 = And(x=w2229, y=w2228) -> (x .and. y?=w2227:bool)
    n1439 = Equal?(x=w2202, y=TRUE) -> (x = y?=w2278:bool)
    n1440 = And(x=w2235, y=w2234) -> (x .and. y?=w2233:bool)
    n1441 = Equal?(x=w2201, y=TRUE) -> (x = y?=w2272:bool)
    n1442 = And(x=w2259, y=w2258) -> (x .and. y?=w2257:bool)
    n1443 = case shown="假" w2221 {
      frame False {
      }
      frame True {
        n1444 = property on="解锁到位" class="Bool (严格)"("Val(Sgnl)"=TRUE) -> ()  [unwired: 2 in, 2 out]
      }
    }
    n1445 = case shown="真" w2251 {
      frame False {
      }
      frame True {
        n1446 = property on="开盖缓冲" class="Bool (严格)"("Val(Sgnl)"=TRUE) -> ()  [unwired: 2 in, 2 out]
      }
    }
    n1447 = case shown="真" w2263 {
      frame False {
      }
      frame True {
        n1448 = property on="关盖到位1" class="Bool (严格)"("Val(Sgnl)"=TRUE) -> ()  [unwired: 2 in, 2 out]
      }
    }
    n1449 = And(x=w2279, y=w2278) -> (x .and. y?=w2280:bool)
    n1450 = case shown="真" w2239 {
      frame False {
      }
      frame True {
        n1451 = property on="锁定到位" class="Bool (严格)"("Val(Sgnl)"=TRUE) -> ()  [unwired: 2 in, 2 out]
      }
    }
    n1452 = case shown="真" w2245 {
      frame False {
      }
      frame True {
        n1453 = property on="关盖缓冲" class="Bool (严格)"("Val(Sgnl)"=TRUE) -> ()  [unwired: 2 in, 2 out]
      }
    }
    n1454 = And(x=w2273, y=w2272) -> (x .and. y?=w2270:bool)
    n1455 = case shown="真" w2227 {
      frame False {
      }
      frame True {
        n1456 = property on="松开到位" class="Bool (严格)"("Val(Sgnl)"=TRUE) -> ()  [unwired: 2 in, 2 out]
      }
    }
    n1457 = case shown="真" w2233 {
      frame False {
      }
      frame True {
        n1458 = property on="压紧到位" class="Bool (严格)"("Val(Sgnl)"=TRUE) -> ()  [unwired: 2 in, 2 out]
      }
    }
    n1459 = case shown="真" w2257 {
      frame False {
      }
      frame True {
        n1460 = property on="关盖到位2" class="Bool (严格)"("Val(Sgnl)"=TRUE) -> ()  [unwired: 2 in, 2 out]
      }
    }
    n1461 = case shown="真" w2280 {
      frame False {
      }
      frame True {
        n1462 = property on="开盖到位1" class="Bool (严格)"("Val(Sgnl)"=TRUE) -> ()  [unwired: 2 in, 2 out]
      }
    }
    n1463 = case shown="真" w2270 {
      frame False {
      }
      frame True {
        n1464 = property on="开盖到位2" class="Bool (严格)"("Val(Sgnl)"=TRUE) -> ()  [unwired: 2 in, 2 out]
      }
    }
    n1465 = global read "全局变量.vi" "开盖到位1"() -> (w2276:bool)
    n1466 = global read "全局变量.vi" "解锁到位"() -> (w2220:bool)
    n1467 = global read "全局变量.vi" "开盖到位2"() -> (w2269:bool)
    n1468 = global read "全局变量.vi" "关盖到位1"() -> (w2262:bool)
    n1469 = global read "全局变量.vi" "开盖缓冲"() -> (w2250:bool)
    n1470 = global read "全局变量.vi" "锁定到位"() -> (w2238:bool)
    n1471 = global read "全局变量.vi" "关盖缓冲"() -> (w2244:bool)
    n1472 = global read "全局变量.vi" "松开到位"() -> (w2226:bool)
    n1473 = global read "全局变量.vi" "压紧到位"() -> (w2232:bool)
    n1474 = global read "全局变量.vi" "关盖到位2"() -> (w2256:bool)
    n1475 = Boolean To (0,1)(Boolean=w2276) -> (0, 1=w2275:i16)
    n1476 = Boolean To (0,1)(Boolean=w2220) -> (0, 1=w2219:i16)
    n1477 = Boolean To (0,1)(Boolean=w2250) -> (0, 1=w2249:i16)
    n1478 = Boolean To (0,1)(Boolean=w2269) -> (0, 1=w2268:i16)
    n1479 = Boolean To (0,1)(Boolean=w2262) -> (0, 1=w2261:i16)
    n1480 = Boolean To (0,1)(Boolean=w2238) -> (0, 1=w2237:i16)
    n1481 = Not Equal To 0?(x=w2275) -> (x != 0?=w2277:bool)
    n1482 = Boolean To (0,1)(Boolean=w2244) -> (0, 1=w2243:i16)
    n1483 = Boolean To (0,1)(Boolean=w2226) -> (0, 1=w2225:i16)
    n1484 = Boolean To (0,1)(Boolean=w2232) -> (0, 1=w2231:i16)
    n1485 = Boolean To (0,1)(Boolean=w2256) -> (0, 1=w2255:i16)
    n1486 = Not Equal To 0?(x=w2219) -> (x != 0?=w2203:bool)
    n1487 = Not Equal To 0?(x=w2249) -> (x != 0?=w2213:bool)
    n1488 = Not Equal To 0?(x=w2268) -> (x != 0?=w2267:bool)
    n1489 = Not Equal To 0?(x=w2261) -> (x != 0?=w2217:bool)
    n1490 = Not Equal To 0?(x=w2237) -> (x != 0?=w2209:bool)
    n1491 = Not Equal To 0?(x=w2243) -> (x != 0?=w2211:bool)
    n1492 = Not Equal To 0?(x=w2225) -> (x != 0?=w2205:bool)
    n1493 = Not Equal To 0?(x=w2231) -> (x != 0?=w2207:bool)
    n1494 = Not Equal To 0?(x=w2255) -> (x != 0?=w2215:bool)
  }
  n1495 = while {
    shift-right: [w2360] -> _
    shift-left: w200 -> [w2301]
    shift-left: w200 -> [w2364]
    shift-right: [w2350] -> _
    shift-left: w207 -> [w2300]
    shift-left: w207 -> [w2354]
    shift-right: [w2312] -> _
    shift-left: w206 -> [w2299]
    shift-left: w206 -> [w2313]
    shift-right: [w2310] -> _
    shift-left: w205 -> [w2298]
    shift-left: w205 -> [w2311]
    shift-right: [w2308] -> _
    shift-left: w204 -> [w2297]
    shift-left: w204 -> [w2309]
    shift-right: [w2306] -> _
    shift-left: w203 -> [w2296]
    shift-left: w203 -> [w2307]
    shift-right: [w2304] -> _
    shift-left: w202 -> [w2295]
    shift-left: w202 -> [w2305]
    shift-right: [w2302] -> _
    shift-left: w201 -> [w2294]
    shift-left: w201 -> [w2303]
    stop <- FALSE stop-if-true
    n1496 = Not Equal?(x=w2294, y=w2303) -> (x != y?=w2318:bool)
    n1497 = Not Equal?(x=w2299, y=w2313) -> (x != y?=w2348:bool)
    n1498 = Not Equal?(x=w2296, y=w2307) -> (x != y?=w2330:bool)
    n1499 = Equal?(x=w2294, y=TRUE) -> (x = y?=w2317:bool)
    n1500 = Not Equal?(x=w2297, y=w2309) -> (x != y?=w2336:bool)
    n1501 = Not Equal?(x=w2295, y=w2305) -> (x != y?=w2324:bool)
    n1502 = Equal?(x=w2299, y=TRUE) -> (x = y?=w2347:bool)
    n1503 = Equal?(x=w2296, y=TRUE) -> (x = y?=w2329:bool)
    n1504 = Equal?(x=w2297, y=TRUE) -> (x = y?=w2335:bool)
    n1505 = Not Equal?(x=w2298, y=w2311) -> (x != y?=w2342:bool)
    n1506 = Equal?(x=w2295, y=TRUE) -> (x = y?=w2323:bool)
    n1507 = And(x=w2318, y=w2317) -> (x .and. y?=w2316:bool)
    n1508 = Equal?(x=w2298, y=TRUE) -> (x = y?=w2341:bool)
    n1509 = Not Equal?(x=w2301, y=w2364) -> (x != y?=w2362:bool)
    n1510 = And(x=w2348, y=w2347) -> (x .and. y?=w2346:bool)
    n1511 = And(x=w2330, y=w2329) -> (x .and. y?=w2328:bool)
    n1512 = Not Equal?(x=w2300, y=w2354) -> (x != y?=w2356:bool)
    n1513 = And(x=w2336, y=w2335) -> (x .and. y?=w2334:bool)
    n1514 = And(x=w2324, y=w2323) -> (x .and. y?=w2322:bool)
    n1515 = Equal?(x=w2301, y=TRUE) -> (x = y?=w2361:bool)
    n1516 = Equal?(x=w2300, y=TRUE) -> (x = y?=w2355:bool)
    n1517 = And(x=w2342, y=w2341) -> (x .and. y?=w2340:bool)
    n1518 = case shown="假" w2316 {
      frame False {
      }
      frame True {
        n1519 = property on="关盖指令2" class="Bool (严格)"("Val(Sgnl)"=TRUE) -> ()  [unwired: 2 in, 2 out]
      }
    }
    n1520 = case shown="假" w2346 {
      frame False {
      }
      frame True {
        n1521 = property on="开盖指令1" class="Bool (严格)"("Val(Sgnl)"=TRUE) -> ()  [unwired: 2 in, 2 out]
      }
    }
    n1522 = And(x=w2362, y=w2361) -> (x .and. y?=w2363:bool)
    n1523 = case shown="假" w2328 {
      frame False {
      }
      frame True {
        n1524 = property on="关盖换向阀" class="Bool (严格)"("Val(Sgnl)"=TRUE) -> ()  [unwired: 2 in, 2 out]
      }
    }
    n1525 = case shown="假" w2334 {
      frame False {
      }
      frame True {
        n1526 = property on="压紧换向阀" class="Bool (严格)"("Val(Sgnl)"=TRUE) -> ()  [unwired: 2 in, 2 out]
      }
    }
    n1527 = And(x=w2356, y=w2355) -> (x .and. y?=w2353:bool)
    n1528 = case shown="假" w2322 {
      frame False {
      }
      frame True {
        n1529 = property on="关盖指令1" class="Bool (严格)"("Val(Sgnl)"=TRUE) -> ()  [unwired: 2 in, 2 out]
      }
    }
    n1530 = case shown="假" w2340 {
      frame False {
      }
      frame True {
        n1531 = property on="开盖指令2" class="Bool (严格)"("Val(Sgnl)"=TRUE) -> ()  [unwired: 2 in, 2 out]
      }
    }
    n1532 = case shown="真" w2363 {
      frame False {
      }
      frame True {
        n1533 = property on="松开换向阀" class="Bool (严格)"("Val(Sgnl)"=TRUE) -> ()  [unwired: 2 in, 2 out]
      }
    }
    n1534 = case shown="真" w2353 {
      frame False {
      }
      frame True {
        n1535 = property on="开盖换向阀" class="Bool (严格)"("Val(Sgnl)"=TRUE) -> ()  [unwired: 2 in, 2 out]
      }
    }
    n1536 = global read "全局变量.vi" "松开换向阀"() -> (w2359:bool)
    n1537 = global read "全局变量.vi" "关盖指令2"() -> (w2315:bool)
    n1538 = global read "全局变量.vi" "开盖换向阀"() -> (w2352:bool)
    n1539 = global read "全局变量.vi" "关盖换向阀"() -> (w2327:bool)
    n1540 = global read "全局变量.vi" "开盖指令1"() -> (w2345:bool)
    n1541 = global read "全局变量.vi" "压紧换向阀"() -> (w2333:bool)
    n1542 = global read "全局变量.vi" "关盖指令1"() -> (w2321:bool)
    n1543 = global read "全局变量.vi" "开盖指令2"() -> (w2339:bool)
    n1544 = Boolean To (0,1)(Boolean=w2359) -> (0, 1=w2358:i16)
    n1545 = Boolean To (0,1)(Boolean=w2315) -> (0, 1=w2314:i16)
    n1546 = Boolean To (0,1)(Boolean=w2352) -> (0, 1=w2351:i16)
    n1547 = Boolean To (0,1)(Boolean=w2345) -> (0, 1=w2344:i16)
    n1548 = Boolean To (0,1)(Boolean=w2327) -> (0, 1=w2326:i16)
    n1549 = Not Equal To 0?(x=w2358) -> (x != 0?=w2360:bool)
    n1550 = Boolean To (0,1)(Boolean=w2333) -> (0, 1=w2332:i16)
    n1551 = Boolean To (0,1)(Boolean=w2321) -> (0, 1=w2320:i16)
    n1552 = Boolean To (0,1)(Boolean=w2339) -> (0, 1=w2338:i16)
    n1553 = Not Equal To 0?(x=w2314) -> (x != 0?=w2302:bool)
    n1554 = Not Equal To 0?(x=w2351) -> (x != 0?=w2350:bool)
    n1555 = Not Equal To 0?(x=w2344) -> (x != 0?=w2312:bool)
    n1556 = Not Equal To 0?(x=w2326) -> (x != 0?=w2306:bool)
    n1557 = Not Equal To 0?(x=w2332) -> (x != 0?=w2308:bool)
    n1558 = Not Equal To 0?(x=w2320) -> (x != 0?=w2304:bool)
    n1559 = Not Equal To 0?(x=w2338) -> (x != 0?=w2310:bool)
  }
  n1560 = while {
    shift-right: [w2424] -> _
    shift-left: w199 -> [w2422]
    shift-left: w199 -> [w2435]
    shift-right: [w2414] -> _
    shift-left: w181 -> [w2417]
    shift-left: w181 -> [w2416]
    shift-right: [w2406] -> _
    shift-left: w182 -> [w2408]
    shift-left: w182 -> [w2407]
    shift-right: [w2403] -> _
    shift-left: w180 -> [w2405]
    shift-left: w180 -> [w2404]
    shift-right: [w2402] -> _
    shift-left: w179 -> [w2396]
    shift-left: w179 -> [w2401]
    shift-right: [w2399] -> _
    shift-left: w178 -> [w2395]
    shift-left: w178 -> [w2400]
    shift-right: [w2397] -> _
    shift-left: w177 -> [w2394]
    shift-left: w177 -> [w2398]
    shift-right: [w2391] -> _
    shift-left: w176 -> [w2392]
    shift-left: w176 -> [w2393]
    shift-right: [w2389] -> _
    shift-left: w175 -> [w2388]
    shift-left: w175 -> [w2390]
    shift-right: [w2385] -> _
    shift-left: w174 -> [w2386]
    shift-left: w174 -> [w2387]
    shift-right: [w2382] -> _
    shift-left: w173 -> [w2383]
    shift-left: w173 -> [w2384]
    shift-right: [w2378] -> _
    shift-left: w172 -> [w2379]
    shift-left: w172 -> [w2381]
    shift-right: [w2377] -> _
    shift-left: w171 -> [w2376]
    shift-left: w171 -> [w2375]
    stop <- w2423 stop-if-true
    n1561 = Not Equal?(x=w2408, y=w2407) -> (x != y?=w2411:bool)
    n1562 = Equal?(x=w2408, y=TRUE) -> (x = y?=w2410:bool)
    n1563 = And(x=w2411, y=w2410) -> (x .and. y?=w2412:bool)
    n1564 = Not Equal?(x=w2396, y=w2401) -> (x != y?=w2472:bool)
    n1565 = Not Equal?(x=w2376, y=w2375) -> (x != y?=w2437:bool)
    n1566 = Not Equal?(x=w2395, y=w2400) -> (x != y?=w2468:bool)
    n1567 = Not Equal?(x=w2383, y=w2384) -> (x != y?=w2444:bool)
    n1568 = Not Equal?(x=w2379, y=w2381) -> (x != y?=w2441:bool)
    n1569 = Not Equal?(x=w2392, y=w2393) -> (x != y?=w2460:bool)
    n1570 = Not Equal?(x=w2388, y=w2390) -> (x != y?=w2456:bool)
    n1571 = Not Equal?(x=w2394, y=w2398) -> (x != y?=w2464:bool)
    n1572 = Not Equal?(x=w2386, y=w2387) -> (x != y?=w2448:bool)
    n1573 = Not Equal?(x=w2417, y=w2416) -> (x != y?=w2419:bool)
    n1574 = Not Equal?(x=w2405, y=w2404) -> (x != y?=w2477:bool)
    n1575 = Not Equal?(x=w2422, y=w2435) -> (x != y?=w2453:bool)
    n1576 = Equal?(x=w2396, y=TRUE) -> (x = y?=w2471:bool)
    n1577 = Equal?(x=w2376, y=TRUE) -> (x = y?=w2436:bool)
    n1578 = Equal?(x=w2395, y=TRUE) -> (x = y?=w2467:bool)
    n1579 = Equal?(x=w2383, y=TRUE) -> (x = y?=w2443:bool)
    n1580 = Equal?(x=w2379, y=TRUE) -> (x = y?=w2440:bool)
    n1581 = Equal?(x=w2392, y=TRUE) -> (x = y?=w2459:bool)
    n1582 = Equal?(x=w2388, y=TRUE) -> (x = y?=w2455:bool)
    n1583 = Equal?(x=w2394, y=TRUE) -> (x = y?=w2463:bool)
    n1584 = Equal?(x=w2386, y=TRUE) -> (x = y?=w2447:bool)
    n1585 = Equal?(x=w2417, y=TRUE) -> (x = y?=w2418:bool)
    n1586 = Equal?(x=w2405, y=TRUE) -> (x = y?=w2476:bool)
    n1587 = Equal?(x=w2422, y=TRUE) -> (x = y?=w2454:bool)
    n1588 = case shown="真" w2412 {
      frame False {
      }
      frame True {
        n1589 = property on="自动操作" class="Bool (严格)"("Val(Sgnl)"=TRUE) -> ()  [unwired: 2 in, 2 out]
      }
    }
    n1590 = And(x=w2472, y=w2471) -> (x .and. y?=w2473:bool)
    n1591 = And(x=w2437, y=w2436) -> (x .and. y?=w2438:bool)
    n1592 = And(x=w2468, y=w2467) -> (x .and. y?=w2469:bool)
    n1593 = And(x=w2444, y=w2443) -> (x .and. y?=w2445:bool)
    n1594 = And(x=w2441, y=w2440) -> (x .and. y?=w2442:bool)
    n1595 = And(x=w2460, y=w2459) -> (x .and. y?=w2461:bool)
    n1596 = And(x=w2456, y=w2455) -> (x .and. y?=w2457:bool)
    n1597 = And(x=w2464, y=w2463) -> (x .and. y?=w2465:bool)
    n1598 = And(x=w2448, y=w2447) -> (x .and. y?=w2449:bool)
    n1599 = And(x=w2419, y=w2418) -> (x .and. y?=w2420:bool)
    n1600 = And(x=w2477, y=w2476) -> (x .and. y?=w2478:bool)
    n1601 = And(x=w2453, y=w2454) -> (x .and. y?=w2452:bool)
    n1602 = case shown="真" w2473 {
      frame False {
      }
      frame True {
        n1603 = property on="调试模式" class="Bool (严格)"("Val(Sgnl)"=TRUE) -> ()  [unwired: 2 in, 2 out]
      }
    }
    n1604 = case shown="真" w2438 {
      frame False {
      }
      frame True {
        n1605 = property on="井盖 8" class="Bool (严格)"("Val(Sgnl)"=TRUE) -> ()  [unwired: 2 in, 2 out]
      }
    }
    n1606 = case shown="真" w2469 {
      frame False {
      }
      frame True {
        n1607 = property on="退出系统" class="Bool (严格)"("Val(Sgnl)"=TRUE) -> ()  [unwired: 2 in, 2 out]
      }
    }
    n1608 = case shown="真" w2445 {
      frame False {
      }
      frame True {
        n1609 = property on="井盖 6" class="Bool (严格)"("Val(Sgnl)"=TRUE) -> ()  [unwired: 2 in, 2 out]
      }
    }
    n1610 = case shown="真" w2442 {
      frame False {
      }
      frame True {
        n1611 = property on="井盖 7" class="Bool (严格)"("Val(Sgnl)"=TRUE) -> ()  [unwired: 2 in, 2 out]
      }
    }
    n1612 = case shown="真" w2461 {
      frame False {
      }
      frame True {
        n1613 = property on="井盖 2" class="Bool (严格)"("Val(Sgnl)"=TRUE) -> ()  [unwired: 2 in, 2 out]
      }
    }
    n1614 = case shown="真" w2457 {
      frame False {
      }
      frame True {
        n1615 = property on="井盖 3" class="Bool (严格)"("Val(Sgnl)"=TRUE) -> ()  [unwired: 2 in, 2 out]
      }
    }
    n1616 = case shown="真" w2465 {
      frame False {
      }
      frame True {
        n1617 = property on="井盖1" class="Bool (严格)"("Val(Sgnl)"=TRUE) -> ()  [unwired: 2 in, 2 out]
      }
    }
    n1618 = case shown="真" w2449 {
      frame False {
      }
      frame True {
        n1619 = property on="井盖 5" class="Bool (严格)"("Val(Sgnl)"=TRUE) -> ()  [unwired: 2 in, 2 out]
      }
    }
    n1620 = case shown="真" w2420 {
      frame False {
      }
      frame True {
        n1621 = property on="手动操作" class="Bool (严格)"("Val(Sgnl)"=TRUE) -> ()  [unwired: 2 in, 2 out]
      }
    }
    n1622 = case shown="真" w2478 {
      frame False {
      }
      frame True {
        n1623 = property on="系统启动" class="Bool (严格)"("Val(Sgnl)"=TRUE) -> ()  [unwired: 2 in, 2 out]
      }
    }
    n1624 = case shown="真" w2452 {
      frame False {
      }
      frame True {
        n1625 = property on="井盖 4" class="Bool (严格)"("Val(Sgnl)"=TRUE) -> ()  [unwired: 2 in, 2 out]
      }
    }
    n1626 = global read "全局变量.vi" "qidongzd"() -> (w2409:dbl)
    n1627 = global read "全局变量.vi" "qidongsd"() -> (w2415:dbl)
    n1628 = global read "全局变量.vi" "tiaoshimoshi"() -> (w2434:dbl)
    n1629 = global read "全局变量.vi" "kaishi1"() -> (w2432:dbl)
    n1630 = global read "全局变量.vi" "kaishi2"() -> (w2431:dbl)
    n1631 = global read "全局变量.vi" "kaishi5"() -> (w2428:dbl)
    n1632 = global read "全局变量.vi" "jieshu"() -> (w2433:dbl)
    n1633 = global read "全局变量.vi" "kaishi8"() -> (w2425:dbl)
    n1634 = global read "全局变量.vi" "kaishi3"() -> (w2430:dbl)
    n1635 = global read "全局变量.vi" "kaishi4"() -> (w2429:dbl)
    n1636 = global read "全局变量.vi" "kaishi6"() -> (w2427:dbl)
    n1637 = global read "全局变量.vi" "kaishi7"() -> (w2426:dbl)
    n1638 = global read "全局变量.vi" "start"() -> (w2475:dbl)
    n1639 = Not Equal To 0?(x=w2409) -> (x != 0?=w2406:bool)
    n1640 = global read "全局变量.vi" "退出系统"() -> (w2423:bool)
    n1641 = Not Equal To 0?(x=w2415) -> (x != 0?=w2414:bool)
    n1642 = Not Equal To 0?(x=w2434) -> (x != 0?=w2402:bool)
    n1643 = Not Equal To 0?(x=w2425) -> (x != 0?=w2377:bool)
    n1644 = Not Equal To 0?(x=w2432) -> (x != 0?=w2397:bool)
    n1645 = Not Equal To 0?(x=w2433) -> (x != 0?=w2399:bool)
    n1646 = Not Equal To 0?(x=w2431) -> (x != 0?=w2391:bool)
    n1647 = Not Equal To 0?(x=w2428) -> (x != 0?=w2385:bool)
    n1648 = Not Equal To 0?(x=w2430) -> (x != 0?=w2389:bool)
    n1649 = Not Equal To 0?(x=w2429) -> (x != 0?=w2424:bool)
    n1650 = Not Equal To 0?(x=w2475) -> (x != 0?=w2403:bool)
    n1651 = Not Equal To 0?(x=w2427) -> (x != 0?=w2382:bool)
    n1652 = Not Equal To 0?(x=w2426) -> (x != 0?=w2378:bool)
  }
  n1653 = while {
    stop <- FALSE stop-if-true
    n1654 = event shown="[1] \"井盖1\": 值改变" {
      selector: _ -> [_ _ _ _ _ _ _ _ _]
      dyn-events: _ -> [_ _ _ _ _ _ _ _ _]
      timeout: _ -> [_ _ _ _ _ _ _ _ _]
      event Timeout {
        n1655 = event-data() -> ()  [unwired: 1 in, 3 out]
      }
      event "井盖1": Value Change {
        n1656 = event-data() -> ("NewVal"=w2498:bool)  [unwired: 1 in, 5 out]
        n1657 = case shown="假" w2498 {
          tunnel: [FALSE ("松开") FALSE ("松开")] -> w2497
          tunnel: [T1."Disabled and Grayed Out" ("禁用") T1."Enabled" ("禁用")] -> w2496
          tunnel: [FALSE ("井盖1") FALSE ("井盖1")] -> w2495
          tunnel: [T1."Enabled" ("禁用") T1."Disabled and Grayed Out" ("禁用")] -> w2494
          frame False {
          }
          frame True {
          }
        }
        n1658 = property on="井盖 3" class="Bool (严格)"("Value"=w2495, "DisabledEnum"=w2494) -> ()  [unwired: 2 in, 2 out]
        n1659 = property on="井盖 2" class="Bool (严格)"("Value"=w2495, "DisabledEnum"=w2494) -> ()  [unwired: 2 in, 2 out]
        n1660 = property on="井盖 4" class="Bool (严格)"("Value"=w2495, "DisabledEnum"=w2494) -> ()  [unwired: 2 in, 2 out]
        n1661 = property on="井盖 5" class="Bool (严格)"("Value"=w2495, "DisabledEnum"=w2494) -> ()  [unwired: 2 in, 2 out]
        n1662 = property on="井盖 6" class="Bool (严格)"("Value"=w2495, "DisabledEnum"=w2494) -> ()  [unwired: 2 in, 2 out]
        n1663 = property on="井盖 8" class="Bool (严格)"("Value"=w2495, "DisabledEnum"=w2494) -> ()  [unwired: 2 in, 2 out]
        n1664 = property on="井盖 7" class="Bool (严格)"("Value"=w2495, "DisabledEnum"=w2494) -> ()  [unwired: 2 in, 2 out]
        n1665 = property on="压紧" class="Bool (严格)"("Value"=w2497, "DisabledEnum"=w2496) -> ()  [unwired: 2 in, 2 out]
        n1666 = property on="开盖" class="Bool (严格)"("Value"=w2497, "DisabledEnum"=w2496) -> ()  [unwired: 2 in, 2 out]
        n1667 = property on="关盖" class="Bool (严格)"("Value"=w2497, "DisabledEnum"=w2496) -> ()  [unwired: 2 in, 2 out]
        n1668 = property on="锁定" class="Bool (严格)"("Value"=w2497, "DisabledEnum"=w2496) -> ()  [unwired: 2 in, 2 out]
        n1669 = property on="解锁" class="Bool (严格)"("Value"=w2497, "DisabledEnum"=w2496) -> ()  [unwired: 2 in, 2 out]
        n1670 = property on="松开" class="Bool (严格)"("Value"=w2497, "DisabledEnum"=w2496) -> ()  [unwired: 2 in, 2 out]
      }
      event "井盖 2": Value Change {
        n1671 = event-data() -> ("NewVal"=w2511:bool)  [unwired: 1 in, 5 out]
        n1672 = case shown="真" w2511 {
          tunnel: [FALSE ("开盖") FALSE ("开盖")] -> w2509
          tunnel: [T1."Disabled and Grayed Out" ("禁用") T1."Enabled" ("禁用")] -> w2510
          tunnel: [FALSE ("井盖1") FALSE ("井盖1")] -> w2508
          tunnel: [T1."Enabled" ("禁用") T1."Disabled and Grayed Out" ("禁用")] -> w2507
          frame False {
          }
          frame True {
          }
        }
        n1673 = property on="井盖 6" class="Bool (严格)"("Value"=w2508, "DisabledEnum"=w2507) -> ()  [unwired: 2 in, 2 out]
        n1674 = property on="井盖1" class="Bool (严格)"("Value"=w2508, "DisabledEnum"=w2507) -> ()  [unwired: 2 in, 2 out]
        n1675 = property on="井盖 7" class="Bool (严格)"("Value"=w2508, "DisabledEnum"=w2507) -> ()  [unwired: 2 in, 2 out]
        n1676 = property on="井盖 3" class="Bool (严格)"("Value"=w2508, "DisabledEnum"=w2507) -> ()  [unwired: 2 in, 2 out]
        n1677 = property on="井盖 4" class="Bool (严格)"("Value"=w2508, "DisabledEnum"=w2507) -> ()  [unwired: 2 in, 2 out]
        n1678 = property on="井盖 8" class="Bool (严格)"("Value"=w2508, "DisabledEnum"=w2507) -> ()  [unwired: 2 in, 2 out]
        n1679 = property on="井盖 5" class="Bool (严格)"("Value"=w2508, "DisabledEnum"=w2507) -> ()  [unwired: 2 in, 2 out]
        n1680 = property on="压紧" class="Bool (严格)"("Value"=w2509, "DisabledEnum"=w2510) -> ()  [unwired: 2 in, 2 out]
        n1681 = property on="松开" class="Bool (严格)"("Value"=w2509, "DisabledEnum"=w2510) -> ()  [unwired: 2 in, 2 out]
        n1682 = property on="解锁" class="Bool (严格)"("Value"=w2509, "DisabledEnum"=w2510) -> ()  [unwired: 2 in, 2 out]
        n1683 = property on="开盖" class="Bool (严格)"("Value"=w2509, "DisabledEnum"=w2510) -> ()  [unwired: 2 in, 2 out]
        n1684 = property on="关盖" class="Bool (严格)"("Value"=w2509, "DisabledEnum"=w2510) -> ()  [unwired: 2 in, 2 out]
        n1685 = property on="锁定" class="Bool (严格)"("Value"=w2509, "DisabledEnum"=w2510) -> ()  [unwired: 2 in, 2 out]
      }
      event "井盖 3": Value Change {
        n1686 = event-data() -> ("NewVal"=w2524:bool)  [unwired: 1 in, 5 out]
        n1687 = case shown="真" w2524 {
          tunnel: [FALSE ("松开") FALSE ("松开")] -> w2523
          tunnel: [T1."Disabled and Grayed Out" ("禁用") T1."Enabled" ("禁用")] -> w2522
          tunnel: [FALSE ("井盖1") FALSE ("井盖1")] -> w2521
          tunnel: [T1."Enabled" ("禁用") T1."Disabled and Grayed Out" ("禁用")] -> w2520
          frame False {
          }
          frame True {
          }
        }
        n1688 = property on="井盖 4" class="Bool (严格)"("Value"=w2521, "DisabledEnum"=w2520) -> ()  [unwired: 2 in, 2 out]
        n1689 = property on="井盖1" class="Bool (严格)"("Value"=w2521, "DisabledEnum"=w2520) -> ()  [unwired: 2 in, 2 out]
        n1690 = property on="井盖 2" class="Bool (严格)"("Value"=w2521, "DisabledEnum"=w2520) -> ()  [unwired: 2 in, 2 out]
        n1691 = property on="井盖 5" class="Bool (严格)"("Value"=w2521, "DisabledEnum"=w2520) -> ()  [unwired: 2 in, 2 out]
        n1692 = property on="井盖 6" class="Bool (严格)"("Value"=w2521, "DisabledEnum"=w2520) -> ()  [unwired: 2 in, 2 out]
        n1693 = property on="井盖 7" class="Bool (严格)"("Value"=w2521, "DisabledEnum"=w2520) -> ()  [unwired: 2 in, 2 out]
        n1694 = property on="井盖 8" class="Bool (严格)"("Value"=w2521, "DisabledEnum"=w2520) -> ()  [unwired: 2 in, 2 out]
        n1695 = property on="锁定" class="Bool (严格)"("Value"=w2523, "DisabledEnum"=w2522) -> ()  [unwired: 2 in, 2 out]
        n1696 = property on="解锁" class="Bool (严格)"("Value"=w2523, "DisabledEnum"=w2522) -> ()  [unwired: 2 in, 2 out]
        n1697 = property on="关盖" class="Bool (严格)"("Value"=w2523, "DisabledEnum"=w2522) -> ()  [unwired: 2 in, 2 out]
        n1698 = property on="开盖" class="Bool (严格)"("Value"=w2523, "DisabledEnum"=w2522) -> ()  [unwired: 2 in, 2 out]
        n1699 = property on="压紧" class="Bool (严格)"("Value"=w2523, "DisabledEnum"=w2522) -> ()  [unwired: 2 in, 2 out]
        n1700 = property on="松开" class="Bool (严格)"("Value"=w2523, "DisabledEnum"=w2522) -> ()  [unwired: 2 in, 2 out]
      }
      event "井盖 4": Value Change {
        n1701 = event-data() -> ("NewVal"=w2537:bool)  [unwired: 1 in, 5 out]
        n1702 = case shown="假" w2537 {
          tunnel: [FALSE ("松开") FALSE ("松开")] -> w2536
          tunnel: [T1."Disabled and Grayed Out" ("禁用") T1."Enabled" ("禁用")] -> w2535
          tunnel: [FALSE ("井盖1") FALSE ("井盖1")] -> w2534
          tunnel: [T1."Enabled" ("禁用") T1."Disabled and Grayed Out" ("禁用")] -> w2533
          frame False {
          }
          frame True {
          }
        }
        n1703 = property on="井盖 5" class="Bool (严格)"("Value"=w2534, "DisabledEnum"=w2533) -> ()  [unwired: 2 in, 2 out]
        n1704 = property on="井盖1" class="Bool (严格)"("Value"=w2534, "DisabledEnum"=w2533) -> ()  [unwired: 2 in, 2 out]
        n1705 = property on="井盖 2" class="Bool (严格)"("Value"=w2534, "DisabledEnum"=w2533) -> ()  [unwired: 2 in, 2 out]
        n1706 = property on="井盖 6" class="Bool (严格)"("Value"=w2534, "DisabledEnum"=w2533) -> ()  [unwired: 2 in, 2 out]
        n1707 = property on="井盖 7" class="Bool (严格)"("Value"=w2534, "DisabledEnum"=w2533) -> ()  [unwired: 2 in, 2 out]
        n1708 = property on="井盖 3" class="Bool (严格)"("Value"=w2534, "DisabledEnum"=w2533) -> ()  [unwired: 2 in, 2 out]
        n1709 = property on="井盖 8" class="Bool (严格)"("Value"=w2534, "DisabledEnum"=w2533) -> ()  [unwired: 2 in, 2 out]
        n1710 = property on="松开" class="Bool (严格)"("Value"=w2536, "DisabledEnum"=w2535) -> ()  [unwired: 2 in, 2 out]
        n1711 = property on="开盖" class="Bool (严格)"("Value"=w2536, "DisabledEnum"=w2535) -> ()  [unwired: 2 in, 2 out]
        n1712 = property on="关盖" class="Bool (严格)"("Value"=w2536, "DisabledEnum"=w2535) -> ()  [unwired: 2 in, 2 out]
        n1713 = property on="解锁" class="Bool (严格)"("Value"=w2536, "DisabledEnum"=w2535) -> ()  [unwired: 2 in, 2 out]
        n1714 = property on="压紧" class="Bool (严格)"("Value"=w2536, "DisabledEnum"=w2535) -> ()  [unwired: 2 in, 2 out]
        n1715 = property on="锁定" class="Bool (严格)"("Value"=w2536, "DisabledEnum"=w2535) -> ()  [unwired: 2 in, 2 out]
      }
      event "井盖 5": Value Change {
        n1716 = event-data() -> ("NewVal"=w2550:bool)  [unwired: 1 in, 5 out]
        n1717 = case shown="假" w2550 {
          tunnel: [FALSE ("松开") FALSE ("松开")] -> w2549
          tunnel: [T1."Disabled and Grayed Out" ("禁用") T1."Enabled" ("禁用")] -> w2548
          tunnel: [FALSE ("井盖1") FALSE ("井盖1")] -> w2547
          tunnel: [T1."Enabled" ("禁用") T1."Disabled and Grayed Out" ("禁用")] -> w2546
          frame False {
          }
          frame True {
          }
        }
        n1718 = property on="井盖1" class="Bool (严格)"("Value"=w2547, "DisabledEnum"=w2546) -> ()  [unwired: 2 in, 2 out]
        n1719 = property on="井盖 6" class="Bool (严格)"("Value"=w2547, "DisabledEnum"=w2546) -> ()  [unwired: 2 in, 2 out]
        n1720 = property on="井盖 2" class="Bool (严格)"("Value"=w2547, "DisabledEnum"=w2546) -> ()  [unwired: 2 in, 2 out]
        n1721 = property on="井盖 7" class="Bool (严格)"("Value"=w2547, "DisabledEnum"=w2546) -> ()  [unwired: 2 in, 2 out]
        n1722 = property on="井盖 3" class="Bool (严格)"("Value"=w2547, "DisabledEnum"=w2546) -> ()  [unwired: 2 in, 2 out]
        n1723 = property on="井盖 8" class="Bool (严格)"("Value"=w2547, "DisabledEnum"=w2546) -> ()  [unwired: 2 in, 2 out]
        n1724 = property on="井盖 4" class="Bool (严格)"("Value"=w2547, "DisabledEnum"=w2546) -> ()  [unwired: 2 in, 2 out]
        n1725 = property on="松开" class="Bool (严格)"("Value"=w2549, "DisabledEnum"=w2548) -> ()  [unwired: 2 in, 2 out]
        n1726 = property on="解锁" class="Bool (严格)"("Value"=w2549, "DisabledEnum"=w2548) -> ()  [unwired: 2 in, 2 out]
        n1727 = property on="锁定" class="Bool (严格)"("Value"=w2549, "DisabledEnum"=w2548) -> ()  [unwired: 2 in, 2 out]
        n1728 = property on="开盖" class="Bool (严格)"("Value"=w2549, "DisabledEnum"=w2548) -> ()  [unwired: 2 in, 2 out]
        n1729 = property on="关盖" class="Bool (严格)"("Value"=w2549, "DisabledEnum"=w2548) -> ()  [unwired: 2 in, 2 out]
        n1730 = property on="压紧" class="Bool (严格)"("Value"=w2549, "DisabledEnum"=w2548) -> ()  [unwired: 2 in, 2 out]
      }
      event "井盖 6": Value Change {
        n1731 = event-data() -> ("NewVal"=w2563:bool)  [unwired: 1 in, 5 out]
        n1732 = case shown="假" w2563 {
          tunnel: [FALSE ("松开") FALSE ("松开")] -> w2562
          tunnel: [T1."Disabled and Grayed Out" ("禁用") T1."Enabled" ("禁用")] -> w2561
          tunnel: [FALSE ("井盖1") FALSE ("井盖1")] -> w2560
          tunnel: [T1."Enabled" ("禁用") T1."Disabled and Grayed Out" ("禁用")] -> w2559
          frame False {
          }
          frame True {
          }
        }
        n1733 = property on="井盖1" class="Bool (严格)"("Value"=w2560, "DisabledEnum"=w2559) -> ()  [unwired: 2 in, 2 out]
        n1734 = property on="井盖 5" class="Bool (严格)"("Value"=w2560, "DisabledEnum"=w2559) -> ()  [unwired: 2 in, 2 out]
        n1735 = property on="井盖 2" class="Bool (严格)"("Value"=w2560, "DisabledEnum"=w2559) -> ()  [unwired: 2 in, 2 out]
        n1736 = property on="井盖 7" class="Bool (严格)"("Value"=w2560, "DisabledEnum"=w2559) -> ()  [unwired: 2 in, 2 out]
        n1737 = property on="井盖 3" class="Bool (严格)"("Value"=w2560, "DisabledEnum"=w2559) -> ()  [unwired: 2 in, 2 out]
        n1738 = property on="井盖 8" class="Bool (严格)"("Value"=w2560, "DisabledEnum"=w2559) -> ()  [unwired: 2 in, 2 out]
        n1739 = property on="井盖 4" class="Bool (严格)"("Value"=w2560, "DisabledEnum"=w2559) -> ()  [unwired: 2 in, 2 out]
        n1740 = property on="关盖" class="Bool (严格)"("Value"=w2562, "DisabledEnum"=w2561) -> ()  [unwired: 2 in, 2 out]
        n1741 = property on="解锁" class="Bool (严格)"("Value"=w2562, "DisabledEnum"=w2561) -> ()  [unwired: 2 in, 2 out]
        n1742 = property on="开盖" class="Bool (严格)"("Value"=w2562, "DisabledEnum"=w2561) -> ()  [unwired: 2 in, 2 out]
        n1743 = property on="压紧" class="Bool (严格)"("Value"=w2562, "DisabledEnum"=w2561) -> ()  [unwired: 2 in, 2 out]
        n1744 = property on="松开" class="Bool (严格)"("Value"=w2562, "DisabledEnum"=w2561) -> ()  [unwired: 2 in, 2 out]
        n1745 = property on="锁定" class="Bool (严格)"("Value"=w2562, "DisabledEnum"=w2561) -> ()  [unwired: 2 in, 2 out]
      }
      event "井盖 7": Value Change {
        n1746 = event-data() -> ("NewVal"=w2576:bool)  [unwired: 1 in, 5 out]
        n1747 = case shown="假" w2576 {
          tunnel: [FALSE ("松开") FALSE ("松开")] -> w2575
          tunnel: [T1."Disabled and Grayed Out" ("禁用") T1."Enabled" ("禁用")] -> w2574
          tunnel: [FALSE ("井盖1") FALSE ("井盖1")] -> w2573
          tunnel: [T1."Enabled" ("禁用") T1."Disabled and Grayed Out" ("禁用")] -> w2572
          frame False {
          }
          frame True {
          }
        }
        n1748 = property on="井盖 4" class="Bool (严格)"("Value"=w2573, "DisabledEnum"=w2572) -> ()  [unwired: 2 in, 2 out]
        n1749 = property on="井盖1" class="Bool (严格)"("Value"=w2573, "DisabledEnum"=w2572) -> ()  [unwired: 2 in, 2 out]
        n1750 = property on="井盖 5" class="Bool (严格)"("Value"=w2573, "DisabledEnum"=w2572) -> ()  [unwired: 2 in, 2 out]
        n1751 = property on="井盖 2" class="Bool (严格)"("Value"=w2573, "DisabledEnum"=w2572) -> ()  [unwired: 2 in, 2 out]
        n1752 = property on="井盖 3" class="Bool (严格)"("Value"=w2573, "DisabledEnum"=w2572) -> ()  [unwired: 2 in, 2 out]
        n1753 = property on="井盖 6" class="Bool (严格)"("Value"=w2573, "DisabledEnum"=w2572) -> ()  [unwired: 2 in, 2 out]
        n1754 = property on="井盖 8" class="Bool (严格)"("Value"=w2573, "DisabledEnum"=w2572) -> ()  [unwired: 2 in, 2 out]
        n1755 = property on="锁定" class="Bool (严格)"("Value"=w2575, "DisabledEnum"=w2574) -> ()  [unwired: 2 in, 2 out]
        n1756 = property on="关盖" class="Bool (严格)"("Value"=w2575, "DisabledEnum"=w2574) -> ()  [unwired: 2 in, 2 out]
        n1757 = property on="压紧" class="Bool (严格)"("Value"=w2575, "DisabledEnum"=w2574) -> ()  [unwired: 2 in, 2 out]
        n1758 = property on="解锁" class="Bool (严格)"("Value"=w2575, "DisabledEnum"=w2574) -> ()  [unwired: 2 in, 2 out]
        n1759 = property on="开盖" class="Bool (严格)"("Value"=w2575, "DisabledEnum"=w2574) -> ()  [unwired: 2 in, 2 out]
        n1760 = property on="松开" class="Bool (严格)"("Value"=w2575, "DisabledEnum"=w2574) -> ()  [unwired: 2 in, 2 out]
      }
      event "井盖 8": Value Change {
        n1761 = event-data() -> ("NewVal"=w2589:bool)  [unwired: 1 in, 5 out]
        n1762 = case shown="假" w2589 {
          tunnel: [FALSE ("松开") FALSE ("松开")] -> w2588
          tunnel: [T1."Disabled and Grayed Out" ("禁用") T1."Enabled" ("禁用")] -> w2587
          tunnel: [FALSE ("井盖1") FALSE ("井盖1")] -> w2586
          tunnel: [T1."Enabled" ("禁用") T1."Disabled and Grayed Out" ("禁用")] -> w2585
          frame False {
          }
          frame True {
          }
        }
        n1763 = property on="井盖 5" class="Bool (严格)"("Value"=w2586, "DisabledEnum"=w2585) -> ()  [unwired: 2 in, 2 out]
        n1764 = property on="井盖1" class="Bool (严格)"("Value"=w2586, "DisabledEnum"=w2585) -> ()  [unwired: 2 in, 2 out]
        n1765 = property on="井盖 6" class="Bool (严格)"("Value"=w2586, "DisabledEnum"=w2585) -> ()  [unwired: 2 in, 2 out]
        n1766 = property on="井盖 2" class="Bool (严格)"("Value"=w2586, "DisabledEnum"=w2585) -> ()  [unwired: 2 in, 2 out]
        n1767 = property on="井盖 3" class="Bool (严格)"("Value"=w2586, "DisabledEnum"=w2585) -> ()  [unwired: 2 in, 2 out]
        n1768 = property on="井盖 7" class="Bool (严格)"("Value"=w2586, "DisabledEnum"=w2585) -> ()  [unwired: 2 in, 2 out]
        n1769 = property on="井盖 4" class="Bool (严格)"("Value"=w2586, "DisabledEnum"=w2585) -> ()  [unwired: 2 in, 2 out]
        n1770 = property on="开盖" class="Bool (严格)"("Value"=w2588, "DisabledEnum"=w2587) -> ()  [unwired: 2 in, 2 out]
        n1771 = property on="解锁" class="Bool (严格)"("Value"=w2588, "DisabledEnum"=w2587) -> ()  [unwired: 2 in, 2 out]
        n1772 = property on="锁定" class="Bool (严格)"("Value"=w2588, "DisabledEnum"=w2587) -> ()  [unwired: 2 in, 2 out]
        n1773 = property on="关盖" class="Bool (严格)"("Value"=w2588, "DisabledEnum"=w2587) -> ()  [unwired: 2 in, 2 out]
        n1774 = property on="压紧" class="Bool (严格)"("Value"=w2588, "DisabledEnum"=w2587) -> ()  [unwired: 2 in, 2 out]
        n1775 = property on="松开" class="Bool (严格)"("Value"=w2588, "DisabledEnum"=w2587) -> ()  [unwired: 2 in, 2 out]
      }
    }
  }
  n1776 = while {
    stop <- FALSE stop-if-true
    n1777 = flat-sequence {
      tunnel: [w2606] -> w2603
      tunnel: [w2605] -> w2600
      tunnel: w2603 -> [w2614]
      tunnel: [w2614] -> w2602
      tunnel: [w2613] -> w2601
      tunnel: w2600 -> [w2613]
      tunnel: w2602 -> [w2619]
      tunnel: w2601 -> [w2617]
      tunnel: [w2616] -> w2598
      tunnel: [w2969] -> w2599
      tunnel: w2598 -> [w2969]
      tunnel: w2599 -> [w2974]
      frame #0 {
        n1778 = Concatenate Strings("保存文件名", ".txt" ("字符串")) -> (w2610:string)
        n1779 = Build Path(base path="保存路径", name or relative path=w2610) -> (appended path=w2612:path)
        n1780 = Open/Create/Replace File(file path (use dialog)=w2612, operation (0:open)=T2."open or create" ("操作(0:open)")) -> (refnum out=w2606:refnum<file>, error out=w2605:errorcluster)  [unwired: 4 in, 1 out]
      }
      frame #1 {
        n1781 = Wait (ms)(milliseconds to wait=u32 10 ("等待时间（毫秒）")) -> ()  [unwired: 1 out]
      }
      frame #2 {
        n1782 = case shown="真" "显示/保存数据" {
          tunnel: w2619 -> [_ w2624]
          tunnel: w2617 -> [_ w2620]
          tunnel: [_ w2620] -> w2616
          frame False {
          }
          frame True {
            n1783 = event shown="[1] \"系统启动\": 值改变" {
              selector: _ -> [_ _ _ _ _ _ _ _ _ _ _ _ _ _ _ _ _ _ _ _ _ _ _ _ _ _ _ _ _ _ _ _]
              dyn-events: _ -> [_ _ _ _ _ _ _ _ _ _ _ _ _ _ _ _ _ _ _ _ _ _ _ _ _ _ _ _ _ _ _ _]
              timeout: _ -> [_ _ _ _ _ _ _ _ _ _ _ _ _ _ _ _ _ _ _ _ _ _ _ _ _ _ _ _ _ _ _ _]
              tunnel: [_ w2628 w2639 w2651 w2661 w2672 w2683 w2694 w2705 w2716 w2727 w2738 w2749 w2760 w2771 w2782 w2794 w2804 w2815 w2826 w2837 w2848 w2859 w2870 w2881 w2892 w2904 w2915 w2925 w2936 w2947 w2958] -> w2623
              event Timeout {
                n1784 = event-data() -> ()  [unwired: 1 in, 3 out]
              }
              event "系统启动": Value Change {
                n1785 = event-data() -> ("NewVal"=w2629:bool)  [unwired: 1 in, 5 out]
                n1786 = case shown="真" w2629 {
                  tunnel: ["" w2632] -> w2628
                  frame False {
                  }
                  frame True {
                    n1787 = call <vilib>:"Space Constant.vi"() -> ("String"=w2636:string)
                    n1788 = Format Date/Time String(time format string (%c)="%H : %M : %S" ("时间格式字符串(%c)")) -> (date/time string=w2634:string)  [unwired: 2 in]
                    n1789 = Format Date/Time String(time format string (%c)="%Y/%m/%d" ("时间格式字符串(%c)")) -> (date/time string=w2637:string)  [unwired: 2 in]
                    n1790 = Concatenate Strings(w2637, w2636, w2634, "系统开始运行" ("字符串"), "\r") -> (w2632:string)
                  }
                }
              }
              event "开盖到位1": Value Change {
                n1791 = event-data() -> ("NewVal"=w2640:bool)  [unwired: 1 in, 5 out]
                n1792 = case shown="真" w2640 {
                  tunnel: ["" w2642] -> w2639
                  frame False {
                  }
                  frame True {
                    n1793 = call <vilib>:"Space Constant.vi"() -> ("String"=w2647:string)
                    n1794 = Format Date/Time String(time format string (%c)="%H : %M : %S" ("时间格式字符串(%c)")) -> (date/time string=w2645:string)  [unwired: 2 in]
                    n1795 = Format Date/Time String(time format string (%c)="%Y/%m/%d" ("时间格式字符串(%c)")) -> (date/time string=w2648:string)  [unwired: 2 in]
                    n1796 = Concatenate Strings(w2648, w2647, w2645, "开盖到位1" ("字符串"), "\r") -> (w2642:string)
                  }
                }
              }
              event "开盖到位2": Value Change {
                n1797 = event-data() -> ("NewVal"=w2650:bool)  [unwired: 1 in, 5 out]
                n1798 = case shown="真" w2650 {
                  tunnel: ["" w2653] -> w2651
                  frame False {
                  }
                  frame True {
                    n1799 = call <vilib>:"Space Constant.vi"() -> ("String"=w2658:string)
                    n1800 = Format Date/Time String(time format string (%c)="%H : %M : %S" ("时间格式字符串(%c)")) -> (date/time string=w2656:string)  [unwired: 2 in]
                    n1801 = Format Date/Time String(time format string (%c)="%Y/%m/%d" ("时间格式字符串(%c)")) -> (date/time string=w2659:string)  [unwired: 2 in]
                    n1802 = Concatenate Strings(w2659, w2658, w2656, "开盖到位2" ("字符串"), "\r") -> (w2653:string)
                  }
                }
              }
              event "关盖到位1": Value Change {
                n1803 = event-data() -> ("NewVal"=w2662:bool)  [unwired: 1 in, 5 out]
                n1804 = case shown="真" w2662 {
                  tunnel: ["" w2664] -> w2661
                  frame False {
                  }
                  frame True {
                    n1805 = call <vilib>:"Space Constant.vi"() -> ("String"=w2669:string)
                    n1806 = Format Date/Time String(time format string (%c)="%H : %M : %S" ("时间格式字符串(%c)")) -> (date/time string=w2667:string)  [unwired: 2 in]
                    n1807 = Format Date/Time String(time format string (%c)="%Y/%m/%d" ("时间格式字符串(%c)")) -> (date/time string=w2670:string)  [unwired: 2 in]
                    n1808 = Concatenate Strings(w2670, w2669, w2667, "关盖到位1" ("字符串"), "\r") -> (w2664:string)
                  }
                }
              }
              event "关盖到位2": Value Change {
                n1809 = event-data() -> ("NewVal"=w2673:bool)  [unwired: 1 in, 5 out]
                n1810 = case shown="真" w2673 {
                  tunnel: ["" w2675] -> w2672
                  frame False {
                  }
                  frame True {
                    n1811 = call <vilib>:"Space Constant.vi"() -> ("String"=w2680:string)
                    n1812 = Format Date/Time String(time format string (%c)="%H : %M : %S" ("时间格式字符串(%c)")) -> (date/time string=w2678:string)  [unwired: 2 in]
                    n1813 = Format Date/Time String(time format string (%c)="%Y/%m/%d" ("时间格式字符串(%c)")) -> (date/time string=w2681:string)  [unwired: 2 in]
                    n1814 = Concatenate Strings(w2681, w2680, w2678, "关盖到位2" ("字符串"), "\r") -> (w2675:string)
                  }
                }
              }
              event "开盖缓冲": Value Change {
                n1815 = event-data() -> ("NewVal"=w2684:bool)  [unwired: 1 in, 5 out]
                n1816 = case shown="真" w2684 {
                  tunnel: ["" w2686] -> w2683
                  frame False {
                  }
                  frame True {
                    n1817 = call <vilib>:"Space Constant.vi"() -> ("String"=w2691:string)
                    n1818 = Format Date/Time String(time format string (%c)="%H : %M : %S" ("时间格式字符串(%c)")) -> (date/time string=w2689:string)  [unwired: 2 in]
                    n1819 = Format Date/Time String(time format string (%c)="%Y/%m/%d" ("时间格式字符串(%c)")) -> (date/time string=w2692:string)  [unwired: 2 in]
                    n1820 = Concatenate Strings(w2692, w2691, w2689, "开盖缓冲" ("字符串"), "\r") -> (w2686:string)
                  }
                }
              }
              event "关盖缓冲": Value Change {
                n1821 = event-data() -> ("NewVal"=w2695:bool)  [unwired: 1 in, 5 out]
                n1822 = case shown="真" w2695 {
                  tunnel: ["" w2697] -> w2694
                  frame False {
                  }
                  frame True {
                    n1823 = call <vilib>:"Space Constant.vi"() -> ("String"=w2702:string)
                    n1824 = Format Date/Time String(time format string (%c)="%H : %M : %S" ("时间格式字符串(%c)")) -> (date/time string=w2700:string)  [unwired: 2 in]
                    n1825 = Format Date/Time String(time format string (%c)="%Y/%m/%d" ("时间格式字符串(%c)")) -> (date/time string=w2703:string)  [unwired: 2 in]
                    n1826 = Concatenate Strings(w2703, w2702, w2700, "关盖缓冲" ("字符串"), "\r") -> (w2697:string)
                  }
                }
              }
              event "锁定到位": Value Change {
                n1827 = event-data() -> ("NewVal"=w2706:bool)  [unwired: 1 in, 5 out]
                n1828 = case shown="真" w2706 {
                  tunnel: ["" w2708] -> w2705
                  frame False {
                  }
                  frame True {
                    n1829 = call <vilib>:"Space Constant.vi"() -> ("String"=w2713:string)
                    n1830 = Format Date/Time String(time format string (%c)="%H : %M : %S" ("时间格式字符串(%c)")) -> (date/time string=w2711:string)  [unwired: 2 in]
                    n1831 = Format Date/Time String(time format string (%c)="%Y/%m/%d" ("时间格式字符串(%c)")) -> (date/time string=w2714:string)  [unwired: 2 in]
                    n1832 = Concatenate Strings(w2714, w2713, w2711, "锁定到位" ("字符串"), "\r") -> (w2708:string)
                  }
                }
              }
              event "压紧到位": Value Change {
                n1833 = event-data() -> ("NewVal"=w2717:bool)  [unwired: 1 in, 5 out]
                n1834 = case shown="真" w2717 {
                  tunnel: ["" w2719] -> w2716
                  frame False {
                  }
                  frame True {
                    n1835 = call <vilib>:"Space Constant.vi"() -> ("String"=w2724:string)
                    n1836 = Format Date/Time String(time format string (%c)="%H : %M : %S" ("时间格式字符串(%c)")) -> (date/time string=w2722:string)  [unwired: 2 in]
                    n1837 = Format Date/Time String(time format string (%c)="%Y/%m/%d" ("时间格式字符串(%c)")) -> (date/time string=w2725:string)  [unwired: 2 in]
                    n1838 = Concatenate Strings(w2725, w2724, w2722, "压紧到位" ("字符串"), "\r") -> (w2719:string)
                  }
                }
              }
              event "松开到位": Value Change {
                n1839 = event-data() -> ("NewVal"=w2728:bool)  [unwired: 1 in, 5 out]
                n1840 = case shown="真" w2728 {
                  tunnel: ["" w2730] -> w2727
                  frame False {
                  }
                  frame True {
                    n1841 = call <vilib>:"Space Constant.vi"() -> ("String"=w2735:string)
                    n1842 = Format Date/Time String(time format string (%c)="%H : %M : %S" ("时间格式字符串(%c)")) -> (date/time string=w2733:string)  [unwired: 2 in]
                    n1843 = Format Date/Time String(time format string (%c)="%Y/%m/%d" ("时间格式字符串(%c)")) -> (date/time string=w2736:string)  [unwired: 2 in]
                    n1844 = Concatenate Strings(w2736, w2735, w2733, "松开到位" ("字符串"), "\r") -> (w2730:string)
                  }
                }
              }
              event "解锁到位": Value Change {
                n1845 = event-data() -> ("NewVal"=w2739:bool)  [unwired: 1 in, 5 out]
                n1846 = case shown="真" w2739 {
                  tunnel: ["" w2741] -> w2738
                  frame False {
                  }
                  frame True {
                    n1847 = call <vilib>:"Space Constant.vi"() -> ("String"=w2746:string)
                    n1848 = Format Date/Time String(time format string (%c)="%H : %M : %S" ("时间格式字符串(%c)")) -> (date/time string=w2744:string)  [unwired: 2 in]
                    n1849 = Format Date/Time String(time format string (%c)="%Y/%m/%d" ("时间格式字符串(%c)")) -> (date/time string=w2747:string)  [unwired: 2 in]
                    n1850 = Concatenate Strings(w2747, w2746, w2744, "解锁到位" ("字符串"), "\r") -> (w2741:string)
                  }
                }
              }
              event "松开换向阀": Value Change {
                n1851 = event-data() -> ("NewVal"=w2750:bool)  [unwired: 1 in, 5 out]
                n1852 = case shown="真" w2750 {
                  tunnel: ["" w2752] -> w2749
                  frame False {
                  }
                  frame True {
                    n1853 = call <vilib>:"Space Constant.vi"() -> ("String"=w2757:string)
                    n1854 = Format Date/Time String(time format string (%c)="%H : %M : %S" ("时间格式字符串(%c)")) -> (date/time string=w2755:string)  [unwired: 2 in]
                    n1855 = Format Date/Time String(time format string (%c)="%Y/%m/%d" ("时间格式字符串(%c)")) -> (date/time string=w2758:string)  [unwired: 2 in]
                    n1856 = Concatenate Strings(w2758, w2757, w2755, "松开换向阀" ("字符串"), "\r") -> (w2752:string)
                  }
                }
              }
              event "开盖换向阀": Value Change {
                n1857 = event-data() -> ("NewVal"=w2761:bool)  [unwired: 1 in, 5 out]
                n1858 = case shown="真" w2761 {
                  tunnel: ["" w2763] -> w2760
                  frame False {
                  }
                  frame True {
                    n1859 = call <vilib>:"Space Constant.vi"() -> ("String"=w2768:string)
                    n1860 = Format Date/Time String(time format string (%c)="%H : %M : %S" ("时间格式字符串(%c)")) -> (date/time string=w2766:string)  [unwired: 2 in]
                    n1861 = Format Date/Time String(time format string (%c)="%Y/%m/%d" ("时间格式字符串(%c)")) -> (date/time string=w2769:string)  [unwired: 2 in]
                    n1862 = Concatenate Strings(w2769, w2768, w2766, "开盖换向阀" ("字符串"), "\r") -> (w2763:string)
                  }
                }
              }
              event "开盖指令1": Value Change {
                n1863 = event-data() -> ("NewVal"=w2772:bool)  [unwired: 1 in, 5 out]
                n1864 = case shown="真" w2772 {
                  tunnel: ["" w2774] -> w2771
                  frame False {
                  }
                  frame True {
                    n1865 = call <vilib>:"Space Constant.vi"() -> ("String"=w2779:string)
                    n1866 = Format Date/Time String(time format string (%c)="%H : %M : %S" ("时间格式字符串(%c)")) -> (date/time string=w2777:string)  [unwired: 2 in]
                    n1867 = Format Date/Time String(time format string (%c)="%Y/%m/%d" ("时间格式字符串(%c)")) -> (date/time string=w2780:string)  [unwired: 2 in]
                    n1868 = Concatenate Strings(w2780, w2779, w2777, "开盖指令1" ("字符串"), "\r") -> (w2774:string)
                  }
                }
              }
              event "开盖指令2": Value Change {
                n1869 = event-data() -> ("NewVal"=w2783:bool)  [unwired: 1 in, 5 out]
                n1870 = case shown="真" w2783 {
                  tunnel: ["" w2785] -> w2782
                  frame False {
                  }
                  frame True {
                    n1871 = call <vilib>:"Space Constant.vi"() -> ("String"=w2790:string)
                    n1872 = Format Date/Time String(time format string (%c)="%H : %M : %S" ("时间格式字符串(%c)")) -> (date/time string=w2788:string)  [unwired: 2 in]
                    n1873 = Format Date/Time String(time format string (%c)="%Y/%m/%d" ("时间格式字符串(%c)")) -> (date/time string=w2791:string)  [unwired: 2 in]
                    n1874 = Concatenate Strings(w2791, w2790, w2788, "开盖指令2" ("字符串"), "\r") -> (w2785:string)
                  }
                }
              }
              event "压紧换向阀": Value Change {
                n1875 = event-data() -> ("NewVal"=w2793:bool)  [unwired: 1 in, 5 out]
                n1876 = case shown="真" w2793 {
                  tunnel: ["" w2796] -> w2794
                  frame False {
                  }
                  frame True {
                    n1877 = call <vilib>:"Space Constant.vi"() -> ("String"=w2801:string)
                    n1878 = Format Date/Time String(time format string (%c)="%H : %M : %S" ("时间格式字符串(%c)")) -> (date/time string=w2799:string)  [unwired: 2 in]
                    n1879 = Format Date/Time String(time format string (%c)="%Y/%m/%d" ("时间格式字符串(%c)")) -> (date/time string=w2802:string)  [unwired: 2 in]
                    n1880 = Concatenate Strings(w2802, w2801, w2799, "压紧换向阀" ("字符串"), "\r") -> (w2796:string)
                  }
                }
              }
              event "关盖换向阀": Value Change {
                n1881 = event-data() -> ("NewVal"=w2805:bool)  [unwired: 1 in, 5 out]
                n1882 = case shown="真" w2805 {
                  tunnel: ["" w2807] -> w2804
                  frame False {
                  }
                  frame True {
                    n1883 = call <vilib>:"Space Constant.vi"() -> ("String"=w2812:string)
                    n1884 = Format Date/Time String(time format string (%c)="%H : %M : %S" ("时间格式字符串(%c)")) -> (date/time string=w2810:string)  [unwired: 2 in]
                    n1885 = Format Date/Time String(time format string (%c)="%Y/%m/%d" ("时间格式字符串(%c)")) -> (date/time string=w2813:string)  [unwired: 2 in]
                    n1886 = Concatenate Strings(w2813, w2812, w2810, "关盖换向阀" ("字符串"), "\r") -> (w2807:string)
                  }
                }
              }
              event "关盖指令1": Value Change {
                n1887 = event-data() -> ("NewVal"=w2816:bool)  [unwired: 1 in, 5 out]
                n1888 = case shown="真" w2816 {
                  tunnel: ["" w2818] -> w2815
                  frame False {
                  }
                  frame True {
                    n1889 = call <vilib>:"Space Constant.vi"() -> ("String"=w2823:string)
                    n1890 = Format Date/Time String(time format string (%c)="%H : %M : %S" ("时间格式字符串(%c)")) -> (date/time string=w2821:string)  [unwired: 2 in]
                    n1891 = Format Date/Time String(time format string (%c)="%Y/%m/%d" ("时间格式字符串(%c)")) -> (date/time string=w2824:string)  [unwired: 2 in]
                    n1892 = Concatenate Strings(w2824, w2823, w2821, "关盖指令1" ("字符串"), "\r") -> (w2818:string)
                  }
                }
              }
              event "关盖指令2": Value Change {
                n1893 = event-data() -> ("NewVal"=w2827:bool)  [unwired: 1 in, 5 out]
                n1894 = case shown="真" w2827 {
                  tunnel: ["" w2829] -> w2826
                  frame False {
                  }
                  frame True {
                    n1895 = call <vilib>:"Space Constant.vi"() -> ("String"=w2834:string)
                    n1896 = Format Date/Time String(time format string (%c)="%H : %M : %S" ("时间格式字符串(%c)")) -> (date/time string=w2832:string)  [unwired: 2 in]
                    n1897 = Format Date/Time String(time format string (%c)="%Y/%m/%d" ("时间格式字符串(%c)")) -> (date/time string=w2835:string)  [unwired: 2 in]
                    n1898 = Concatenate Strings(w2835, w2834, w2832, "关盖指令2" ("字符串"), "\r") -> (w2829:string)
                  }
                }
              }
              event "松开": Value Change {
                n1899 = event-data() -> ("NewVal"=w2838:bool)  [unwired: 1 in, 5 out]
                n1900 = case shown="真" w2838 {
                  tunnel: ["" w2840] -> w2837
                  frame False {
                  }
                  frame True {
                    n1901 = call <vilib>:"Space Constant.vi"() -> ("String"=w2845:string)
                    n1902 = Format Date/Time String(time format string (%c)="%H : %M : %S" ("时间格式字符串(%c)")) -> (date/time string=w2843:string)  [unwired: 2 in]
                    n1903 = Format Date/Time String(time format string (%c)="%Y/%m/%d" ("时间格式字符串(%c)")) -> (date/time string=w2846:string)  [unwired: 2 in]
                    n1904 = Concatenate Strings(w2846, w2845, w2843, "开始松开操作" ("字符串"), "\r") -> (w2840:string)
                  }
                }
              }
              event "解锁": Value Change {
                n1905 = event-data() -> ("NewVal"=w2849:bool)  [unwired: 1 in, 5 out]
                n1906 = case shown="真" w2849 {
                  tunnel: ["" w2851] -> w2848
                  frame False {
                  }
                  frame True {
                    n1907 = call <vilib>:"Space Constant.vi"() -> ("String"=w2856:string)
                    n1908 = Format Date/Time String(time format string (%c)="%H : %M : %S" ("时间格式字符串(%c)")) -> (date/time string=w2854:string)  [unwired: 2 in]
                    n1909 = Format Date/Time String(time format string (%c)="%Y/%m/%d" ("时间格式字符串(%c)")) -> (date/time string=w2857:string)  [unwired: 2 in]
                    n1910 = Concatenate Strings(w2857, w2856, w2854, "开始解锁操作" ("字符串"), "\r") -> (w2851:string)
                  }
                }
              }
              event "关盖": Value Change {
                n1911 = event-data() -> ("NewVal"=w2860:bool)  [unwired: 1 in, 5 out]
                n1912 = case shown="真" w2860 {
                  tunnel: ["" w2862] -> w2859
                  frame False {
                  }
                  frame True {
                    n1913 = call <vilib>:"Space Constant.vi"() -> ("String"=w2867:string)
                    n1914 = Format Date/Time String(time format string (%c)="%H : %M : %S" ("时间格式字符串(%c)")) -> (date/time string=w2865:string)  [unwired: 2 in]
                    n1915 = Format Date/Time String(time format string (%c)="%Y/%m/%d" ("时间格式字符串(%c)")) -> (date/time string=w2868:string)  [unwired: 2 in]
                    n1916 = Concatenate Strings(w2868, w2867, w2865, "开始关盖操作" ("字符串"), "\r") -> (w2862:string)
                  }
                }
              }
              event "开盖": Value Change {
                n1917 = event-data() -> ("NewVal"=w2871:bool)  [unwired: 1 in, 5 out]
                n1918 = case shown="真" w2871 {
                  tunnel: ["" w2873] -> w2870
                  frame False {
                  }
                  frame True {
                    n1919 = call <vilib>:"Space Constant.vi"() -> ("String"=w2878:string)
                    n1920 = Format Date/Time String(time format string (%c)="%H : %M : %S" ("时间格式字符串(%c)")) -> (date/time string=w2876:string)  [unwired: 2 in]
                    n1921 = Format Date/Time String(time format string (%c)="%Y/%m/%d" ("时间格式字符串(%c)")) -> (date/time string=w2879:string)  [unwired: 2 in]
                    n1922 = Concatenate Strings(w2879, w2878, w2876, "开始开盖操作" ("字符串"), "\r") -> (w2873:string)
                  }
                }
              }
              event "压紧": Value Change {
                n1923 = event-data() -> ("NewVal"=w2882:bool)  [unwired: 1 in, 5 out]
                n1924 = case shown="真" w2882 {
                  tunnel: ["" w2884] -> w2881
                  frame False {
                  }
                  frame True {
                    n1925 = call <vilib>:"Space Constant.vi"() -> ("String"=w2889:string)
                    n1926 = Format Date/Time String(time format string (%c)="%H : %M : %S" ("时间格式字符串(%c)")) -> (date/time string=w2887:string)  [unwired: 2 in]
                    n1927 = Format Date/Time String(time format string (%c)="%Y/%m/%d" ("时间格式字符串(%c)")) -> (date/time string=w2890:string)  [unwired: 2 in]
                    n1928 = Concatenate Strings(w2890, w2889, w2887, "开始压紧操作" ("字符串"), "\r") -> (w2884:string)
                  }
                }
              }
              event "锁定": Value Change {
                n1929 = event-data() -> ("NewVal"=w2893:bool)  [unwired: 1 in, 5 out]
                n1930 = case shown="真" w2893 {
                  tunnel: ["" w2896] -> w2892
                  frame False {
                  }
                  frame True {
                    n1931 = call <vilib>:"Space Constant.vi"() -> ("String"=w2900:string)
                    n1932 = Format Date/Time String(time format string (%c)="%H : %M : %S" ("时间格式字符串(%c)")) -> (date/time string=w2898:string)  [unwired: 2 in]
                    n1933 = Format Date/Time String(time format string (%c)="%Y/%m/%d" ("时间格式字符串(%c)")) -> (date/time string=w2901:string)  [unwired: 2 in]
                    n1934 = Concatenate Strings(w2901, w2900, w2898, "开始锁定操作" ("字符串"), "\r") -> (w2896:string)
                  }
                }
              }
              event "松开异常": Value Change {
                n1935 = event-data() -> ("NewVal"=w2903:bool)  [unwired: 1 in, 5 out]
                n1936 = case shown="真" w2903 {
                  tunnel: ["" w2907] -> w2904
                  frame False {
                  }
                  frame True {
                    n1937 = call <vilib>:"Space Constant.vi"() -> ("String"=w2911:string)
                    n1938 = Format Date/Time String(time format string (%c)="%H : %M : %S" ("时间格式字符串(%c)")) -> (date/time string=w2909:string)  [unwired: 2 in]
                    n1939 = Format Date/Time String(time format string (%c)="%Y/%m/%d" ("时间格式字符串(%c)")) -> (date/time string=w2912:string)  [unwired: 2 in]
                    n1940 = Concatenate Strings(w2912, w2911, w2909, "松开换向阀发生异常" ("字符串"), "\r") -> (w2907:string)
                  }
                }
              }
              event "开盖异常": Value Change {
                n1941 = event-data() -> ("NewVal"=w2914:bool)  [unwired: 1 in, 5 out]
                n1942 = case shown="真" w2914 {
                  tunnel: ["" w2918] -> w2915
                  frame False {
                  }
                  frame True {
                    n1943 = call <vilib>:"Space Constant.vi"() -> ("String"=w2922:string)
                    n1944 = Format Date/Time String(time format string (%c)="%H : %M : %S" ("时间格式字符串(%c)")) -> (date/time string=w2920:string)  [unwired: 2 in]
                    n1945 = Format Date/Time String(time format string (%c)="%Y/%m/%d" ("时间格式字符串(%c)")) -> (date/time string=w2923:string)  [unwired: 2 in]
                    n1946 = Concatenate Strings(w2923, w2922, w2920, "开盖换向阀发生异常" ("字符串"), "\r") -> (w2918:string)
                  }
                }
              }
              event "锁定异常": Value Change {
                n1947 = event-data() -> ("NewVal"=w2926:bool)  [unwired: 1 in, 5 out]
                n1948 = case shown="真" w2926 {
                  tunnel: ["" w2929] -> w2925
                  frame False {
                  }
                  frame True {
                    n1949 = call <vilib>:"Space Constant.vi"() -> ("String"=w2933:string)
                    n1950 = Format Date/Time String(time format string (%c)="%H : %M : %S" ("时间格式字符串(%c)")) -> (date/time string=w2931:string)  [unwired: 2 in]
                    n1951 = Format Date/Time String(time format string (%c)="%Y/%m/%d" ("时间格式字符串(%c)")) -> (date/time string=w2934:string)  [unwired: 2 in]
                    n1952 = Concatenate Strings(w2934, w2933, w2931, "锁定换向阀发生异常" ("字符串"), "\r") -> (w2929:string)
                  }
                }
              }
              event "解锁异常": Value Change {
                n1953 = event-data() -> ("NewVal"=w2937:bool)  [unwired: 1 in, 5 out]
                n1954 = case shown="真" w2937 {
                  tunnel: ["" w2940] -> w2936
                  frame False {
                  }
                  frame True {
                    n1955 = call <vilib>:"Space Constant.vi"() -> ("String"=w2944:string)
                    n1956 = Format Date/Time String(time format string (%c)="%H : %M : %S" ("时间格式字符串(%c)")) -> (date/time string=w2942:string)  [unwired: 2 in]
                    n1957 = Format Date/Time String(time format string (%c)="%Y/%m/%d" ("时间格式字符串(%c)")) -> (date/time string=w2945:string)  [unwired: 2 in]
                    n1958 = Concatenate Strings(w2945, w2944, w2942, "解锁换向阀发生异常" ("字符串"), "\r") -> (w2940:string)
                  }
                }
              }
              event "关盖异常": Value Change {
                n1959 = event-data() -> ("NewVal"=w2948:bool)  [unwired: 1 in, 5 out]
                n1960 = case shown="真" w2948 {
                  tunnel: ["" w2951] -> w2947
                  frame False {
                  }
                  frame True {
                    n1961 = call <vilib>:"Space Constant.vi"() -> ("String"=w2955:string)
                    n1962 = Format Date/Time String(time format string (%c)="%H : %M : %S" ("时间格式字符串(%c)")) -> (date/time string=w2953:string)  [unwired: 2 in]
                    n1963 = Format Date/Time String(time format string (%c)="%Y/%m/%d" ("时间格式字符串(%c)")) -> (date/time string=w2956:string)  [unwired: 2 in]
                    n1964 = Concatenate Strings(w2956, w2955, w2953, "关盖换向阀发生异常" ("字符串"), "\r") -> (w2951:string)
                  }
                }
              }
              event "压紧异常": Value Change {
                n1965 = event-data() -> ("NewVal"=w2959:bool)  [unwired: 1 in, 5 out]
                n1966 = case shown="真" w2959 {
                  tunnel: ["" w2962] -> w2958
                  frame False {
                  }
                  frame True {
                    n1967 = call <vilib>:"Space Constant.vi"() -> ("String"=w2966:string)
                    n1968 = Format Date/Time String(time format string (%c)="%H : %M : %S" ("时间格式字符串(%c)")) -> (date/time string=w2964:string)  [unwired: 2 in]
                    n1969 = Format Date/Time String(time format string (%c)="%Y/%m/%d" ("时间格式字符串(%c)")) -> (date/time string=w2967:string)  [unwired: 2 in]
                    n1970 = Concatenate Strings(w2967, w2966, w2964, "压紧换向阀发生异常" ("字符串"), "\r") -> (w2962:string)
                  }
                }
              }
            }
            n1971 = Set File Position(refnum=w2624, from (0:start)=enum16{"start", "end", "current"}."end" ("自（0:起始）"), error in=w2620) -> (refnum out=w2626:refnum<file>, error out=w2622:errorcluster)  [unwired: 1 in]
            n1972 = Write to Text File(file (use dialog)=w2626, text=w2623, error in=w2622) -> (refnum out=w2627:refnum<file>, error out=w2621:errorcluster)  [unwired: 1 in, 1 out]
            n1973 = Close File(refnum=w2627, error in=w2621) -> ()  [unwired: 2 out]
          }
        }
      }
      frame #3 {
        n1974 = Wait (ms)(milliseconds to wait=u32 10 ("等待时间（毫秒）")) -> ()  [unwired: 1 out]
      }
      frame #4 {
        n1975 = property on="保存路径" class="Path"() -> ("Value"=w2987:path)  [unwired: 2 in, 2 out]
        n1976 = Path To String(path=w2987) -> (string=w2986:string)
        n1977 = property on="保存文件名" class="Str"() -> ("Value"=w2984:string)  [unwired: 2 in, 2 out]
        n1978 = Concatenate Strings(w2986, "\\" ("字符串"), w2984, ".txt") -> (w2982:string)
        n1979 = String To Path(string=w2982) -> (path=w2981:path)
        n1980 = Open/Create/Replace File(file path (use dialog)=w2981, error in=w2974, operation (0:open)=T2."open or create" ("操作(0:open)"), access (0:read/write)=enum16{"read/write", "read-only", "write-only"}."read-only" ("权限(0:read/write)")) -> (refnum out=w2978:refnum<file>, error out=w2973:errorcluster)  [unwired: 2 in, 1 out]
        n1981 = Set File Position(refnum=w2978, error in=w2973) -> (refnum out=w2977:refnum<file>, error out=w2972:errorcluster)  [unwired: 2 in]
        n1982 = Read from Text File(file (use dialog)=w2977, error in=w2972) -> (refnum out=w2976:refnum<file>, text=→"状态记录":string, error out=w2971:errorcluster)  [unwired: 2 in, 1 out]
        n1983 = Close File(refnum=w2976, error in=w2971) -> ()  [unwired: 2 out]
      }
    }
  }
  n1984 = flat-sequence {
    frame #0 {
      n1985 = property on="显示/保存数据" class="Bool (严格)"("Value"=FALSE ("显示/保存数据")) -> ()  [unwired: 2 in, 2 out]
      n1986 = Format Date/Time String(time format string (%c)="%y-%m-%d-%H-%M-%S") -> (date/time string=w2989:string)  [unwired: 2 in]
      n1987 = Concatenate Strings("状态保存", w2989) -> (w2992:string)
      n1988 = property on="保存文件名" class="Str"("Value"=w2992) -> ()  [unwired: 2 in, 2 out]
      n1989 = property on="状态记录" class="Str"("Text.Scroll Position"=inf) -> ()  [unwired: 2 in, 2 out]
      n1990 = property on="状态记录" class="Str"("Value"="") -> ()  [unwired: 2 in, 2 out]
    }
  }
